vi "main BK20240228.vi"() -> ()   [LabVIEW 2024]
doc: "Main VI for FLS imaging system."
uses:
  <userlib>/_OpenG.lib/file/file.llb/openg_file.lvlib
  <vilib>/event_ctls.llb/usereventprio.ctl
  <instrlib>/niScope/Acquire/Fetch/niScope Multi Fetch Binary 16.vi
  <instrlib>/niScope/Controls/niScope trigger source.ctl
  <userlib>/_OpenG.lib/time/time.llb/openg_time.lvlib
  LaguerreDeconLib/DeconEngineClass/LaguerreDeconEngineClass.lvclass
  SubVI/GlobalVariables.vi
  SubVI/LabJack/LJ Pin Setting.ctl
  <vilib>/Utility/error.llb/DialogType.ctl
  <vilib>/Analysis/NI_AALBase.lvlib
  <vilib>/Utility/miscctls.llb/LVMinMaxIncTypeDef.ctl
  <vilib>/Analysis/baseanly.llb/Mean (DBL).vi
  <vilib>/Utility/miscctls.llb/LVPointTypeDef.ctl
  SubVI/APD/APDClass.lvclass
  ConfigFiles/AimingBeamVideoConfig.ctl
  <vilib>/addons/control/pid/NI_PID_pid.lvlib
  <vilib>/addons/control/pid/pid.llb/PID (DBL).vi
  <vilib>/Instr/_visa.llb/VISA Configure Serial Port (Instr).vi
  SubVI/DigitizerConfiguration/FLImDAQ.ctl
panel:
  out "RunStartTime":u32
  out "Dig1 Temp":dbl
  out "Dig2 Temp":dbl
  out "Visualization PC video source":T1
  in  "V target(1.0)":dbl=1.0 caption="V target(1.5)" min=0.3 max=1.5 step=0.1 format="%#_4g"
  out "SNR3":dbl format="%#_3g"
  out "SNR2":dbl format="%#_3g"
  out "SNR1":dbl format="%#_3g"
  in  "Show BG removed?":bool=TRUE
  out "IntR3":dbl format="%#_2g"
  out "IntR2":dbl format="%#_2g"
  out "IntR1":dbl format="%#_2g"
  in  "Video Display":bool
  out "Gain3":dbl
  out "Gain2":dbl
  out "Gain1":dbl
  in  "Skip Data Save?":bool
  out "Aq Loop?":bool
  out "ML?":bool
  out "aquisition loop Error Out":errorcluster
  out "Laser f (Hz)":dbl
  out "Record Backlog":i32
  out "Fetch Record #":i32
  out "Sync Success?":bool
  out "Disclamer":picture
  out "Calibration #":i8
  out "BG #":i8
  in  "TCP Connect":bool
  out "Help":string
  in  "355nm Laser toggle":bool caption="355nm 460Hz"
  in  "Cali&iRF alignment":bool
  in  "Background":bool
  in  "Aiming beam toggle":bool caption="445nm 15Hz 35mA"
  out "Lifetime 3":dbl
  out "Lifetime 2":dbl
  in  "Auto gain ch3":bool=TRUE
  in  "Auto gain ch2":bool=TRUE
  in  "Auto gain ch1":bool=TRUE
  out "Run #":i8
  in  "StopButton":bool caption="Stop"
  out "Aquisition Status:":bool
  in  "StartButton":bool caption="Start"
  in  "V 3":dbl caption="Gain 3" min=0.0 max=4.6494 step=0.1
  in  "V 2":dbl caption="Gain 2" min=0.0 max=4.61 step=0.1
  out "Lifetime 1":dbl
  in  "V 1":dbl caption="Gain 1" min=0.0 max=4.6492 step=0.1 format="%#_4g"
  in  "Video Source":enum32{"Camera", "FrameGrabber"}(radio)
  out "Case #":string
  out "System Hardware Connection Status":T2
  out "Channel 3":dbl[][](graph)
  out "Channel 2":dbl[][](graph)
  out "Channel 1":dbl[][](graph)
  in  "Tab Control":T3(tab)
  out "display loop timing(ms)":u32
  out "Aquisition loop timing(ms)":u32 format="%.2f"
  out "DisplayLoop":i32
  out "PID loop":i32 caption="processing loop"
  out "PID loop timing(ms)":u32 caption="processing loop timing(ms)"
  out "Communication loop(ms)":u32
  out "laser EM lamp V":dbl format="%0.6f"
  out "Decon Loop timing (ms)":dbl
  out "Auisition Loop idx":i32
  in  "Show BG":bool
  out "iRF length":i32
  out "BG length":i32
  out "data length":i32
  out "SysConfigCluster":T4
  out "LJ Pinout":T5={"Ch1 Bias"="DAC0", "Ch2 Bias"="DAC1", "Ch3 Bias"="DAC2", "Ch4 Bias"="DAC0", "355 PWM"="FIO0", "AimingBeam PWM"="FIO2", "Laser Ready"="FIO3", "Interlock"="FIO1", "Laser Start/Stop"="FIO1", "Red LED"="FIO1", "Green LED"="DIO3", "Foot Pedal"="DIO15"}
  out "FLImDAQ":T6={"Digitizer 1"="", "Digitizer 2"="", "Channel"=enum."Channel 0", "trigger source"="VAL_EXTERNAL", "trigger level"=0.5, "trigger delay"=1.35e-07, "min sample rate"=12500000000.0, "min record length"=2500, "vertical range"=1.0, "vertical offset"=-0.25, "Waveform to Avg"=2000} caption="FLIm DAQ Configuration" {"trigger delay" format="%^#.4e"; "trigger level" min=0.0 max=3.5 step=0.5 format="%.2f"; "vertical offset" format="%.4f"; "vertical range" format="%.2f"; "min sample rate" format="%#.2p"}
  in  "Sys Reconfig":bool
  out "data out(communcation loop)":string
  out "PID loop error out":errorcluster caption="processing Error Out"
  out "decon error out":errorcluster
  out "Laser Rep Rate":dbl
  in  "Data Class":enum16{"Data", "BG", "Cali"}(ring)
  out "V1 Size":i32
  out "V2 Size":i32
  out "V3 Size":i32
  out "data Size":i32[](array[numeric])
  out "State log":string
  in  "Ch3 PID gains":T8={"proportional gain (Kc)"=30.0, "integral time (Ti, min)"=0.0003, "derivative time (Td, min)"=1e-05}
  in  "Ch2 PID gains":T8={"proportional gain (Kc)"=30.0, "integral time (Ti, min)"=0.0003, "derivative time (Td, min)"=1e-05}
  in  "Ch1 PID gains":T8={"proportional gain (Kc)"=30.0, "integral time (Ti, min)"=0.0003, "derivative time (Td, min)"=1e-05}
  in  "Quit":bool
  in  "Radio Buttons":enum32{"No Selection", "Ch1", "Ch2", "Ch3"}(radio)=enum."Ch2" caption="DeCon Chan"
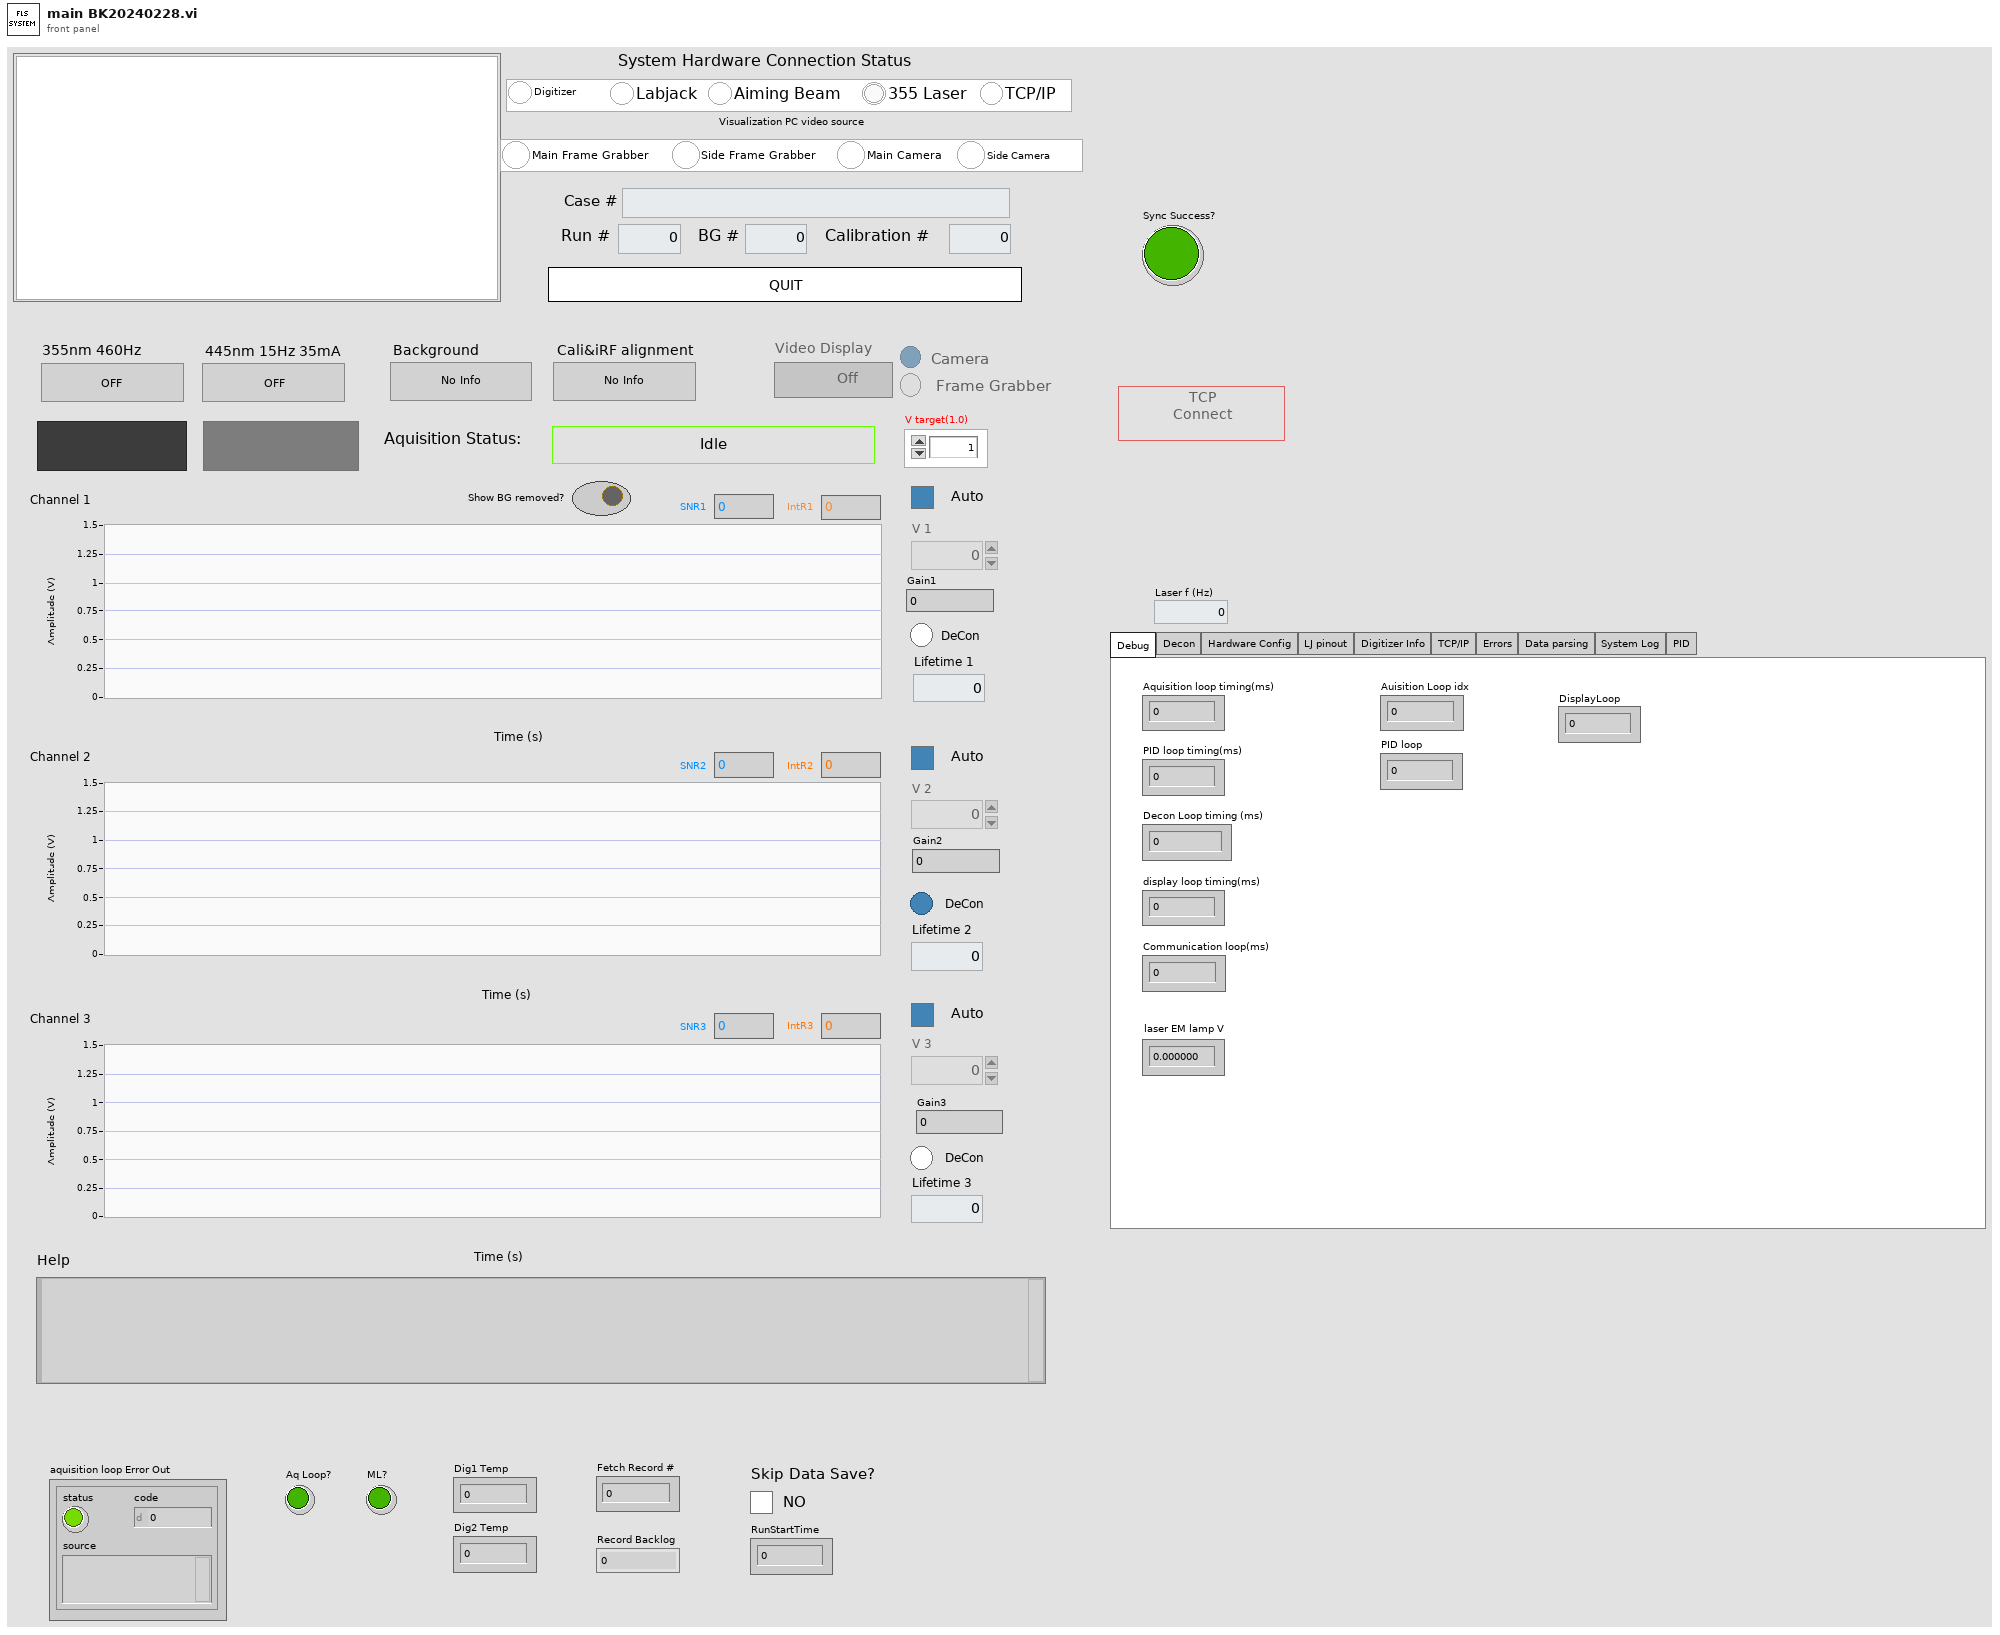
[diagram p1: front panel]
types:
  T1 = cluster{"Main Frame Grabber":bool, "Side Frame Grabber":bool, "Main Camera":bool, "Side Camera":bool}
  T2 = cluster{"Digitizer":bool, "Labjack":bool, "Aiming Beam":bool, "355 Laser":bool, "TCP/IP":bool}
  T3 = enum32{"Debug", "Decon", "Hardware Config", "LJ pinout", "Digitizer Info", "TCP/IP", "Errors", "Data parsing", "System Log", "PID"}
  T4 = cluster{"Ch1Enable?":bool, "Ch2Enable?":bool, "Ch3Enable?":bool, "Ch1AutoGain?":bool, "Ch2AutoGain?":bool, "Ch3AutoGain?":bool, "AimingBeamEnable?":bool}
  T5 = typedef "LJ Pin Setting.ctl" = cluster{"Ch1 Bias":string, "Ch2 Bias":string, "Ch3 Bias":string, "Ch4 Bias":string, "355 PWM":string, "AimingBeam PWM":string, "Laser Ready":string, "Interlock":string, "Laser Start/Stop":string, "Red LED":string, "Green LED":string, "Foot Pedal":string}
  T6 = typedef "FLImDAQ.ctl" = cluster{"Digitizer 1":refnum<k15>, "Digitizer 2":refnum<k15>, "Channel":enum16{"Channel 0", "Channel 1", "Channel 0&1"}, "trigger source":T7, "trigger level":dbl, "trigger delay":dbl, "min sample rate":dbl, "min record length":i32, "vertical range":dbl, "vertical offset":dbl, "Waveform to Avg":i16}
  T7 = typedef "niScope trigger source.ctl" = string
  T8 = cluster{"proportional gain (Kc)":dbl, "integral time (Ti, min)":dbl, "derivative time (Td, min)":dbl}
  T9 = cluster{"remote start event":refnum<user-event>, "remote stop  event":refnum<user-event>}
  T10 = enum8{"Enabled", "Disabled", "Disabled and Grayed Out"}
  T11 = enum16{"open", "replace", "create", "open or create", "replace or create", "replace or create with confirmation"}
  T12 = cluster{"CH1":dbl[][], "CH2":dbl[][], "CH3":dbl[][], "Gain cluster":cluster{"V1":dbl, "V2":dbl, "V3":dbl}}
  T13 = cluster{"idx":i32, "CH1&2":dbl[][], "CH3":dbl[][], "V cluster":cluster{"V1":dbl, "V2":dbl, "V3":dbl}}
  T14 = typedef "usereventprio.ctl" = enum32{"high priority", "normal priority"}
  T15 = cluster{"actualSamples":i32, "absoluteInitialX":dbl, "relativeInitialX":dbl, "xIncrement":dbl, "offset":dbl, "gain":dbl, "reserved1":dbl, "reserved2":dbl}[]
  T16 = cluster{"V1 out":dbl, "V2 out":dbl, "V3 out":dbl}
  T17 = cluster{i32, dbl[][], dbl[][], cluster{"V1 out":dbl, "V2 out":dbl, "V3 out":dbl}}
  T18 = cluster{"Ch1 WF":dbl[], "Ch2 WF":dbl[], "Ch3 WF":dbl[], "V1":dbl, "V2":dbl, "V3":dbl}
  T19 = enum16{"open", "open or create", "create or replace", "create", "open (read-only)"}
  T20 = enum32{"Invalid", "Standard", "Closed", "Hidden", "Minimized", "Maximized"}
  T21 = enum32{"invalid app kind", "Development System", "Run Time System", "Student Edition", "Embedded LabVIEW", "Evaluation", "Custom"}
  T22 = enum32{"Bad", "Idle", "Run top level", "Running"}
  T23 = enum16{"Standard", "Buffered", "CRLF", "Immediate"}
  T24 = typedef "AimingBeamVideoConfig.ctl" = cluster{"DeCon Channel":enum16{"1", "2", "3"}, "Scale Bar":bool, "Scale Low":dbl, "Scale High":dbl, "ANSI":dbl, "Radius":dbl, "3D?":bool, "Firefly?":bool, "Pentero?":bool}
  T25 = cluster{"Core":cluster{"Current VI Reference":refnum<vi>, "Close Panel on Exit?":bool}, "SysConfigCluster":cluster{"Ch1Enable?":bool, "Ch2Enable?":bool, "Ch3Enable?":bool, "Ch1AutoGain?":bool, "Ch2AutoGain?":bool, "Ch3AutoGain?":bool, "AimingBeamEnable?":bool}, "System Status":cluster{"Digitizer":bool, "Labjack":bool, "Aiming Beam":bool, "355 Laser":bool, "TCP/IP":bool}, "IDs":cluster{"RunID":i8, "BG ID":i8, "Cali ID":i8}, "CaseID":string, "DefaultPath":path, "Pathes":cluster{"DataPath":path, "BG Path":path, "iRFPath":path, "CaliPath":path}, "FLImDAQ":cluster{"resource name":refnum<k15>, "resource name 2":refnum<k15>, "Channel":enum16{"Channel 0", "Channel 1", "Channel 0&1"}, "trigger source":T7, "trigger level":dbl, "trigger delay":dbl, "min sample rate":dbl, "min record length":i32, "vertical range":dbl, "vertical offset":dbl, "Waveform to Avg":i32}, "SysRunning?":bool, "AB Cluster":cluster{"Aiming Beam COM Port":refnum<visa-resource-name>, "Min Current":dbl, "Max Current":dbl, "Default Current":dbl, "Freq":i32}, "LJ Pinout":T5, "355 PWM setting":cluster{"DIO_EF_CLOCK1_DIVISOR":i16, "DIO_EF_CLOCK1_ROLL_VALUE":i32, "DIO#_EF_INDEX":i16, "DIO#_EF_OPTIONS":i16, "DIO#_EF_CONFIG_A":i32}, "AB PWM setting":cluster{"DIO_EF_CLOCK1_DIVISOR":i16, "DIO_EF_CLOCK1_ROLL_VALUE":i32, "DIO#_EF_INDEX":i16, "DIO#_EF_OPTIONS":i16, "DIO#_EF_CONFIG_A":i32}, "Last Trigger":u32, "niTClk sessions":refnum<k20>[], "Laser start tic":u32, "TCP attempt count":i32, "Ch1Data":dbl[][], "Ch2Data":dbl[][], "Ch3Data":dbl[][], "V1":dbl[], "V2":dbl[], "V3":dbl[], "SlowTimer":u32, "FastTimer":u32, "listener ID":refnum<k5>, "TempPath":path, "LED vi reference":refnum<vi>, "Aquisition Timer":u32, "APDSerialNum":cluster{"Ch1APDSerial#":string, "Ch2APDSerial#":string, "Ch3APDSerial#":string}, "VideoConfig":T24, "CaliPath":path, "LED vi ref open?":bool, "video source":cluster{"Main Frame Grabber":bool, "Side Frame Grabber":bool, "Main Camera":bool, "Side Camera":bool}, "bothVidSourceAvail":bool}
  T26 = typedef "LVCursorListTypeDef.ctl" = cluster{"Name":string, "Color":u32, "Style":u8, "Point Style":u8, "Name Visible":bool, "Allow Drag":bool, "Cursor Mode":u32, "Plot":i32, "Index":i32, "Position":cluster{"X":dbl, "Y":dbl}, "X Scale":u32, "Y Scale":u32, "Watch Plots":i32[], "Watch All Plots":bool, "Plot Area":i32, "Label Offset":cluster{"X":dbl, "Y":dbl}}[]
  T27 = cluster{"Name":string, "Color":u32, "Style":u8, "Point Style":u8, "Name Visible":bool, "Allow Drag":bool, "Cursor Mode":u32, "Plot":i32, "Index":i32, "Position":cluster{"X":dbl, "Y":dbl}, "X Scale":u32, "Y Scale":u32, "Watch Plots":i32[], "Watch All Plots":bool, "Plot Area":i32, "Label Offset":cluster{"X":dbl, "Y":dbl}}
  T28 = cluster{"Ch1APDSerial#":string, "Ch2APDSerial#":string, "Ch3APDSerial#":string}
  T29 = cluster{"DataPath":path, "BG Path":path, "iRFPath":path, "CaliPath":path}
  T30 = cluster{"DIO_EF_CLOCK1_DIVISOR":i16, "DIO_EF_CLOCK1_ROLL_VALUE":i32, "DIO#_EF_INDEX":i16, "DIO#_EF_OPTIONS":i16, "DIO#_EF_CONFIG_A":i32}
  T31 = cluster{"Aiming Beam COM Port":refnum<visa-resource-name>, "Min Current":dbl, "Max Current":dbl, "Default Current":dbl, "Freq":i32}
  T32 = cluster{"resource name":refnum<k15>, "resource name 2":refnum<k15>, "Channel":enum16{"Channel 0", "Channel 1", "Channel 0&1"}, "trigger source":T7, "trigger level":dbl, "trigger delay":dbl, "min sample rate":dbl, "min record length":i32, "vertical range":dbl, "vertical offset":dbl, "Waveform to Avg":i32}
  T33 = cluster{"Current VI Reference":refnum<vi>, "Close Panel on Exit?":bool}
  T34 = typedef "iRFData.ctl" = cluster{"dt":dbl, "NumOfWFs":i32, "WFLength":i32, "iRFCtrlV":dbl[], "iRFWFsAvg":dbl[][], "iRFRaw":dbl[][]}
  T35 = cluster{"iRFWFsAvg":dbl[], "iRFWFsAvg":dbl[], "iRFWFsAvg":dbl[]}
  T36 = cluster{"V 1":dbl[], "V 2":dbl[], "V 3":dbl[], "V 4":dbl[]}
  T37 = cluster{"Channel 1":dbl[], "Channel 2":dbl[], "Channel 3":dbl[], "Channel 4":dbl[]}
  T38 = cluster{"DataPath":path, "CaseID":string, "RunID":i8, "Ch1Data":dbl[][], "Ch2Data":dbl[][], "Ch3Data":dbl[][], "V1":dbl[], "V2":dbl[], "V3":dbl[], "LaserRepRate":u32, "WFAverage":i16, "RunStartTime":u32}
  T39 = typedef "DialogType.ctl" = u16
  T40 = cluster{"Ch1 iRF":dbl[], "Ch2 iRF":dbl[], "Ch3 iRF":dbl[], "Ch4 iRF":dbl[]}
  T41 = cluster{"Ch1APDSerial#":string, "Ch2APDSerial#":string, "Ch3APDSerial#":string, "Ch4APDSerial#":string}
  T42 = typedef "LJ PWM Setting.ctl" = cluster{"DIO_EF_CLOCK1_DIVISOR":i16, "DIO_EF_CLOCK1_ROLL_VALUE":i32, "DIO#_EF_INDEX":i16, "DIO#_EF_OPTIONS":i16, "DIO#_EF_CONFIG_A":i32}
  T43 = typedef "AimingBeam.ctl" = cluster{"Aiming Beam COM Port":refnum<visa-resource-name>, "Min Current":dbl, "Max Current":dbl, "Default Current":dbl, "Frequency(Hz)":u32}
  T44 = cluster{"DC1":i32, "DC2":i32, "BG1":i32, "BG2":i32}
  T45 = typedef "LVMinMaxIncTypeDef.ctl" = cluster{"Minimum":dbl, "Maximum":dbl, "Increment":dbl}
  T46 = typedef "LVBoundsTypeDef.ctl" = cluster{"Width":u32, "Height":u32}
  T47 = typedef "imagedata.ctl" = cluster{"image type":i32, "image depth":i32, "image":u8[], "mask":u8[], "colors":u32[], "Rectangle":cluster{"left":i16, "top":i16, "right":i16, "bottom":i16}}
  T48 = enum32{"No Selection", "Ch1", "Ch2", "Ch3", "Ch4"}
  T49 = cluster{"DC Idx1":i32, "DC Idx2":i32, "BG Idx1":i32, "BG Idx2":i32}
  T50 = cluster{dbl[][], dbl[][], dbl[][], "V cluster":cluster{"V1":dbl, "V2":dbl, "V3":dbl}}
  T51 = typedef "LVPointTypeDef.ctl" = cluster{"Horizontal":i16, "Vertical":i16}
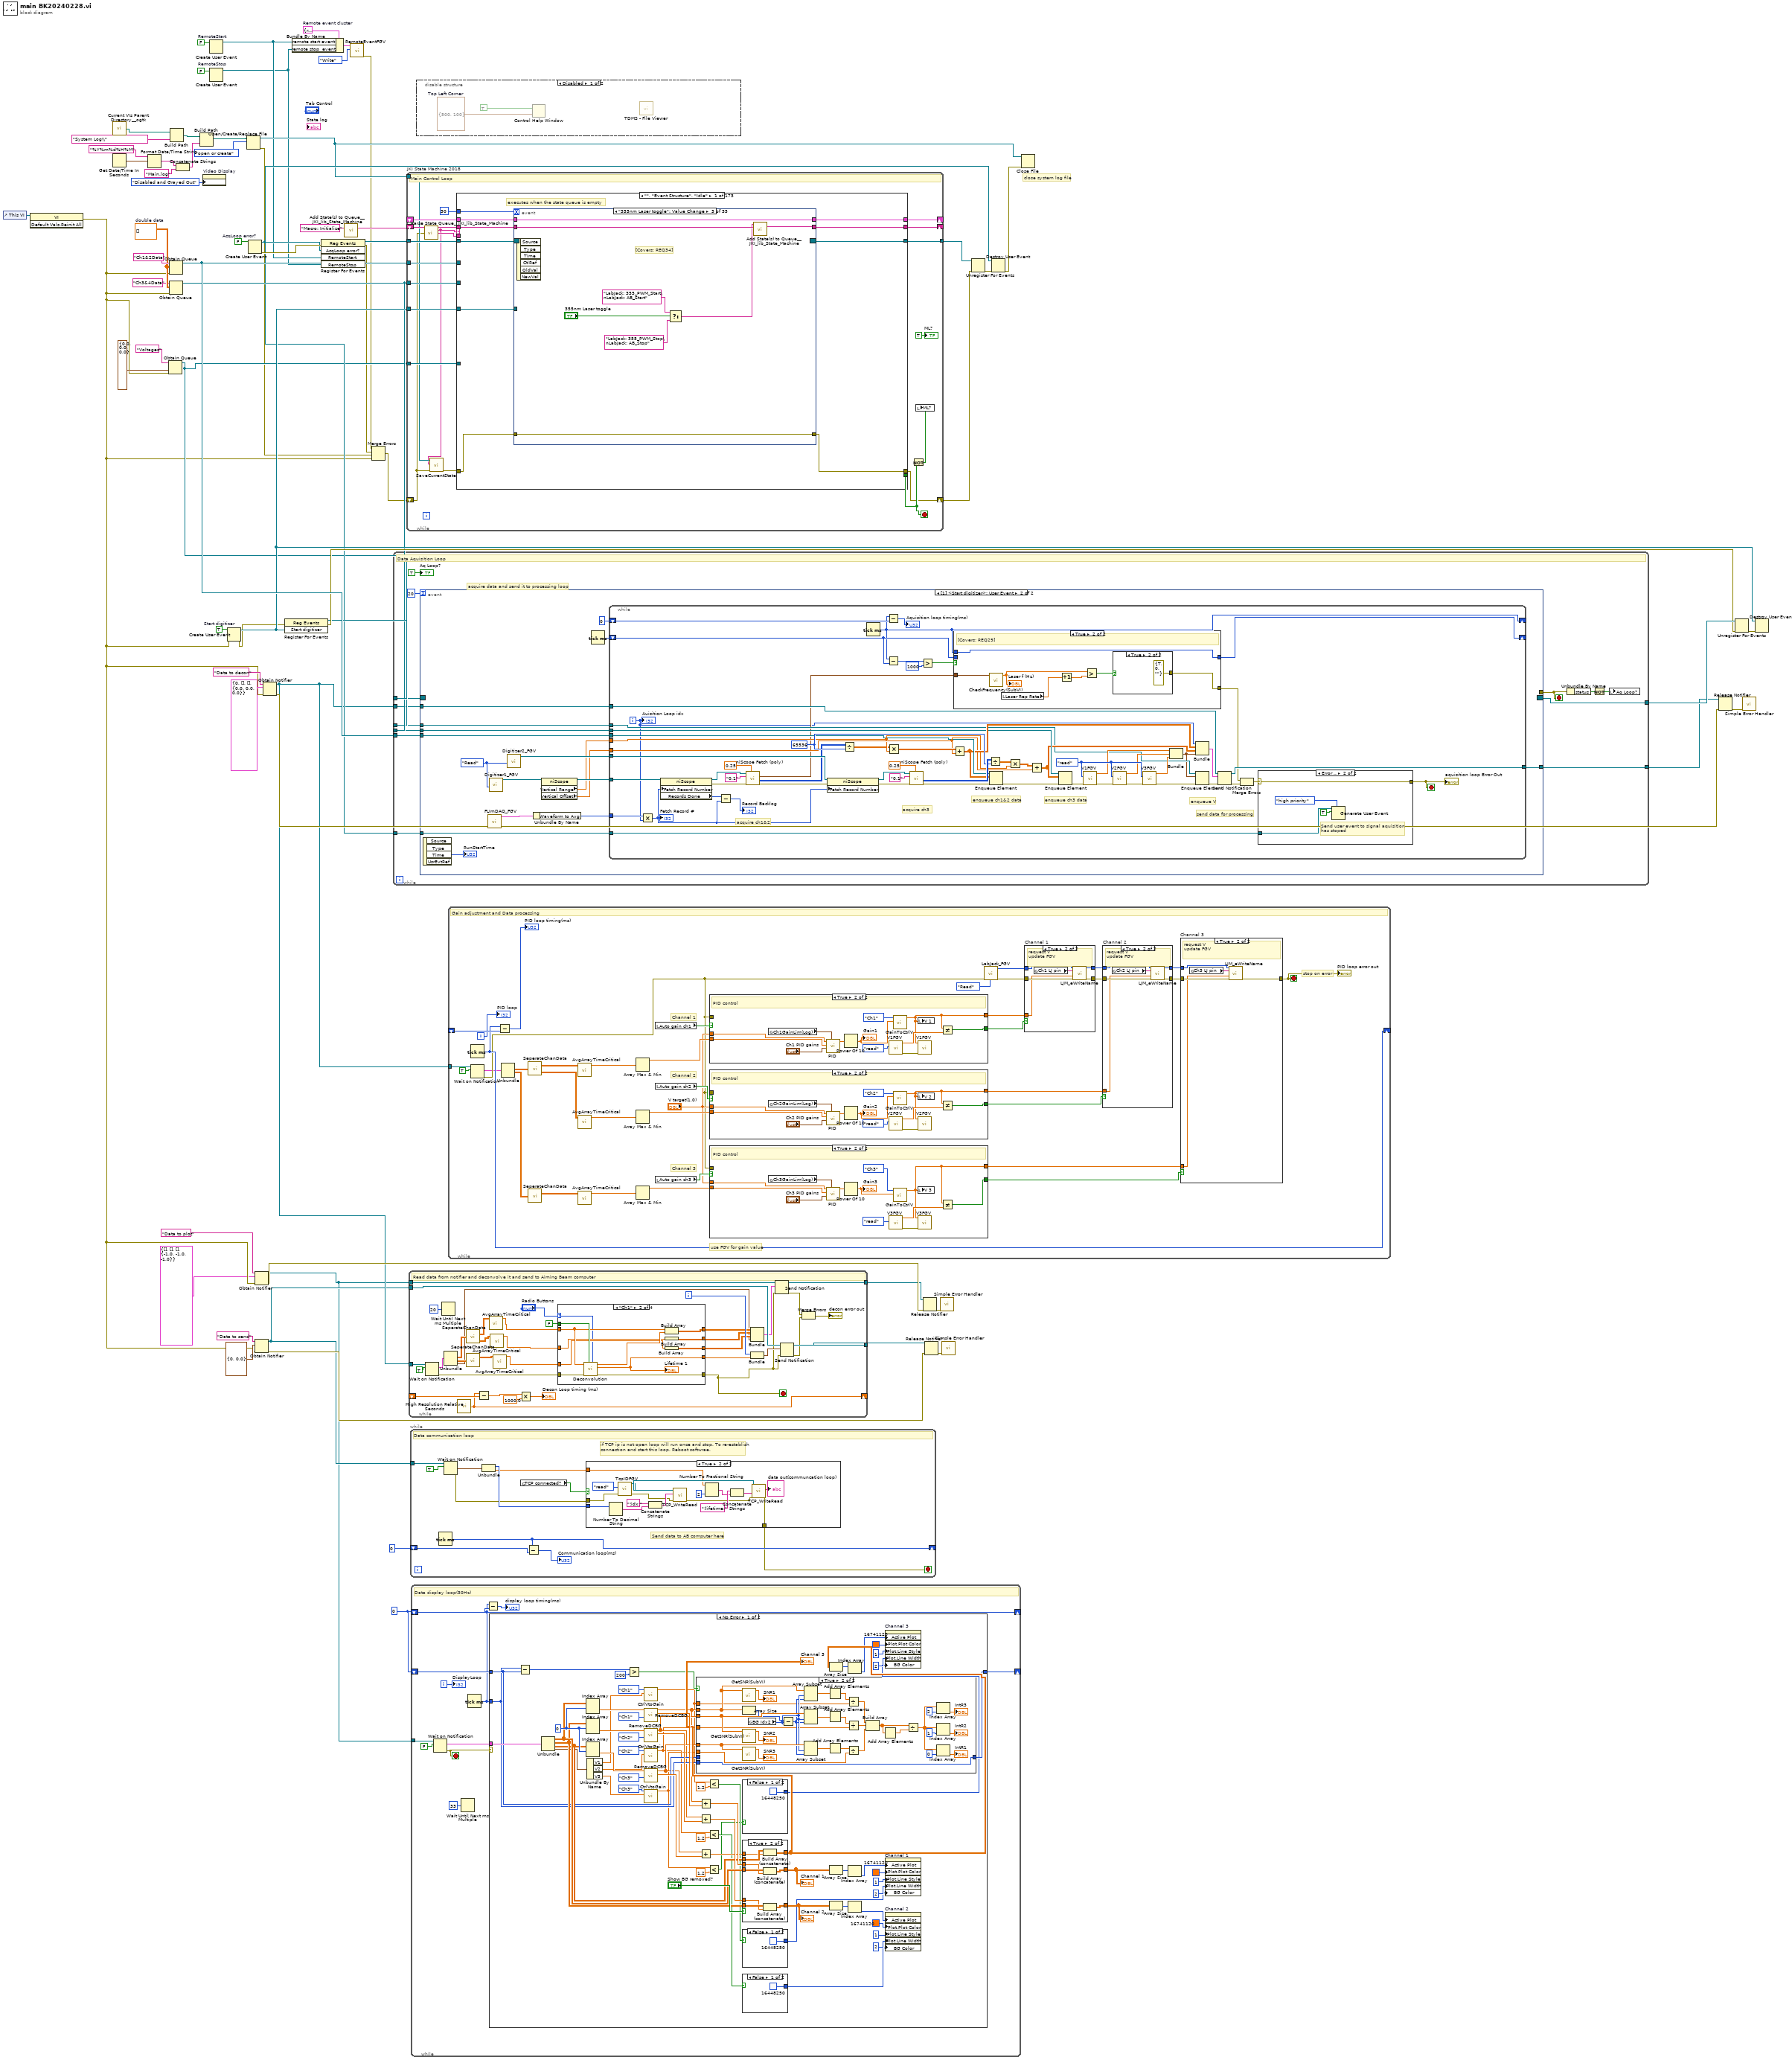
[diagram p0: block diagram]
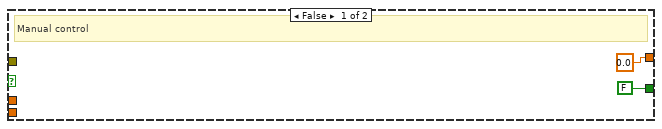
[diagram p2: hidden frame]
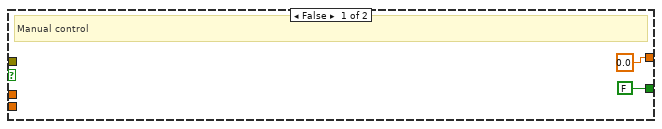
[diagram p6: hidden frame]
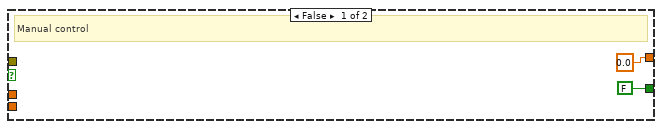
[diagram p7: hidden frame]
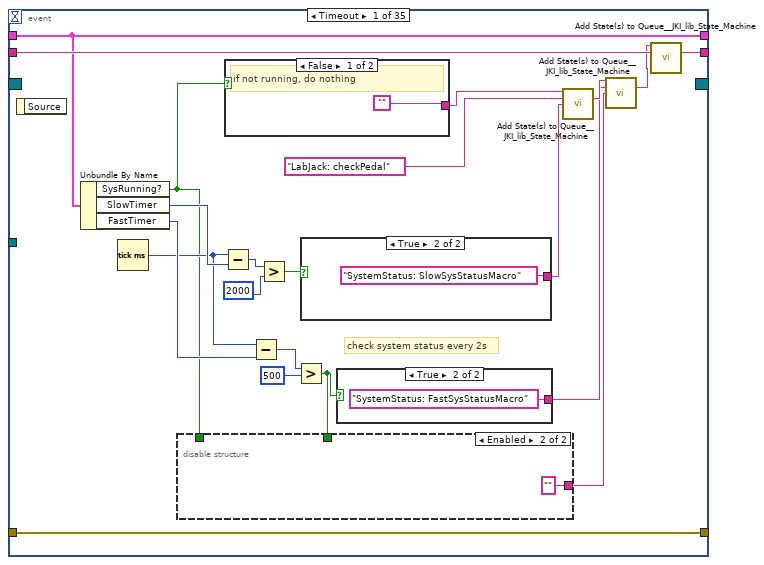
[diagram p8: hidden frame]
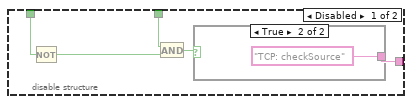
[diagram p9: hidden frame]
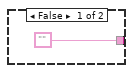
[diagram p10: hidden frame]
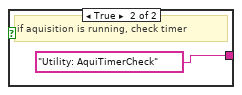
[diagram p11: hidden frame]
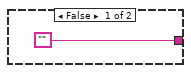
[diagram p12: hidden frame]
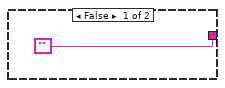
[diagram p13: hidden frame]
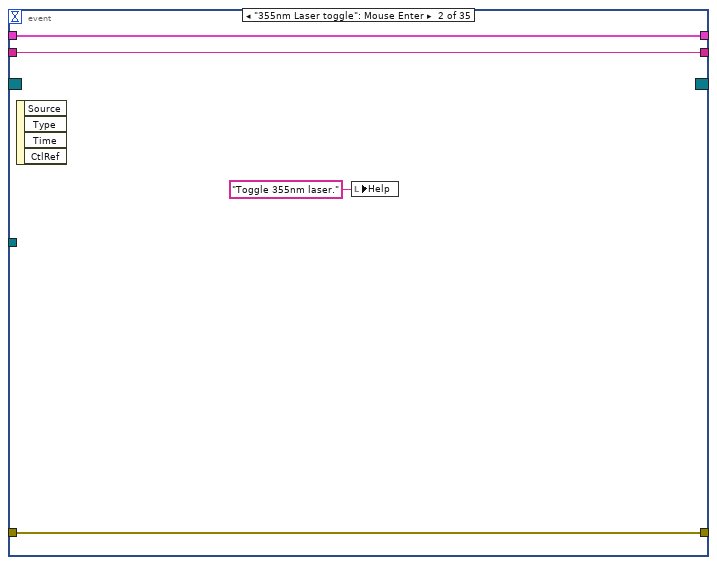
[diagram p14: hidden frame]
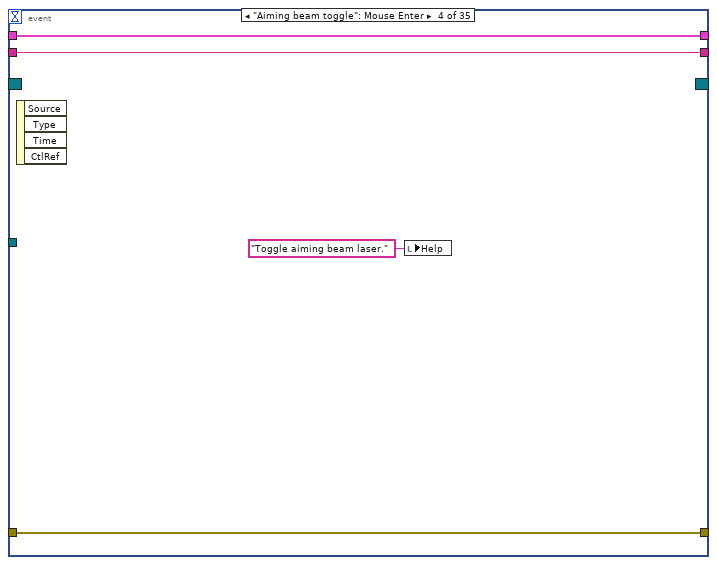
[diagram p15: hidden frame]
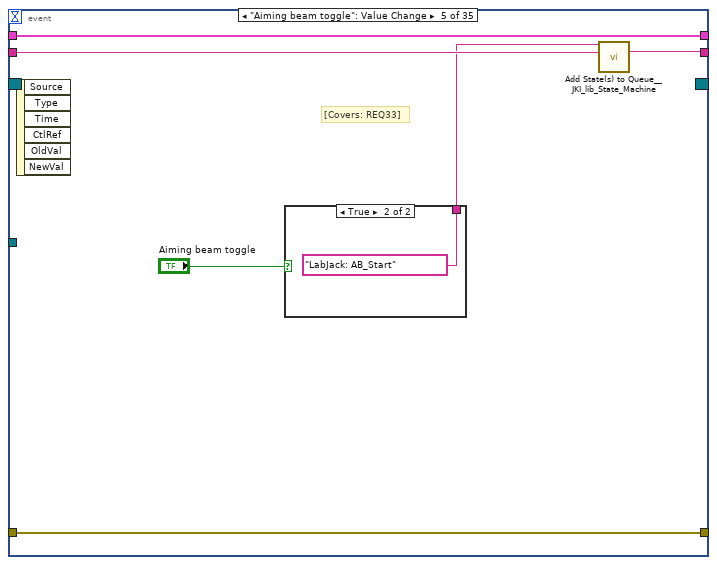
[diagram p16: hidden frame]
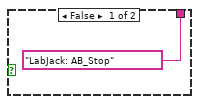
[diagram p17: hidden frame]
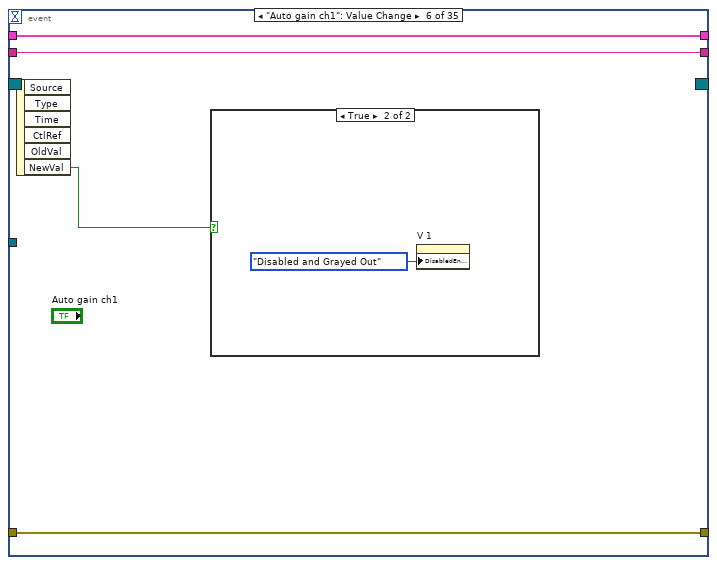
[diagram p18: hidden frame]
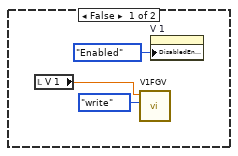
[diagram p19: hidden frame]
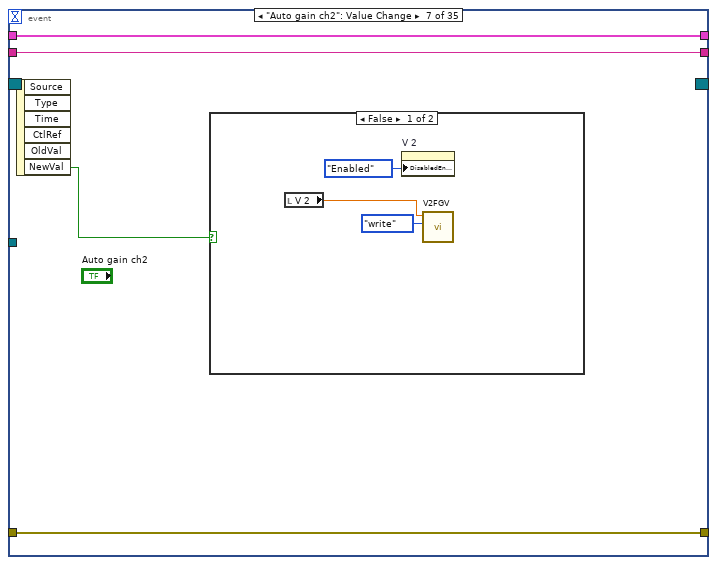
[diagram p20: hidden frame]
diagram:
  w7 = T9 {"remote start event"=refnum, "remote stop  event"=refnum}  # Remote event cluster
  w10 = FALSE  # RemoteStop
  w11 = FALSE  # RemoteStart
  w14 = u32 0 ("millisecond timer value")
  w53 = FALSE  # AcqLoop error?
  w63 = TRUE  # Start digitizer
  w66 = dbl[][] []  # double data
  # "close system log file"
  n1 = control-ref of="This VI"() -> (w68:refnum<vi>)
  n2 = invoke on="Invoke Node" class="VI" method="Default Vals.Reinit All"(reference=w68) -> (error out=w22:errorcluster)  [unwired: 2 in, 2 out]
  n3 = call <userlib>:"Current VIs Parent Directory__ogtk.vi"() -> ("Parent Directory (+ Relative)"=w33:path)  [unwired: 5 in]
  n4 = Get Date/Time In Seconds() -> (seconds since 1Jan1904=w31:timestamp)
  n5 = Format Date/Time String(time format string (%c)="%Y%m%d%H%M", seconds (now)=w31) -> (date/time string=w28:string)  [unwired: 1 in]
  n6 = Obtain Queue(name (unnamed)="Voltages", element data type=cluster{"V1":dbl, "V2":dbl, "V3":dbl} {"V1"=0.0, "V2"=0.0, "V3"=0.0}, error in (no error)=w22) -> (queue out=w34:refnum<queue>)  [unwired: 2 in, 2 out]
  n7 = Obtain Queue(name (unnamed)="Ch3&4Data", element data type=w66, error in (no error)=w22) -> (queue out=w47:refnum<queue>)  [unwired: 2 in, 2 out]
  n8 = Obtain Queue(name (unnamed)="Ch1&2Data", element data type=w66, error in (no error)=w22) -> (queue out=w64:refnum<queue>)  [unwired: 2 in, 2 out]
  n9 = Build Path(base path=w33, name or relative path="System Log\\") -> (appended path=w24:path)
  n10 = Concatenate Strings(w28, "Main.log" ("string")) -> (w26:string)
  n11 = Build Path(base path=w24, name or relative path=w26) -> (appended path=w29:path)
  n12 = property on="Video Display" class="Bool (strict)"("DisabledEnum"=T10."Disabled and Grayed Out" ("Disabled")) -> ()  [unwired: 2 in, 2 out]
  n13 = Create User Event(user event datatype=w11) -> (user event=w9:refnum<user-event>)  [unwired: 1 in, 1 out]
  n14 = Create User Event(user event datatype=w10) -> (user event=w8:refnum<user-event>)  [unwired: 1 in, 1 out]
  n15 = Create User Event(user event datatype=w63, error in=w22) -> (user event=w52:refnum<user-event>, error out=w39:errorcluster)
  n16 = Open/Create/Replace File(file path (use dialog)=w29, operation (0:open)=T11."open or create") -> (refnum out=w20:refnum<file>, error out=w21:errorcluster)  [unwired: 4 in, 1 out]
  n17 = Create User Event(user event datatype=w53) -> (user event=w38:refnum<user-event>, error out=w40:errorcluster)  [unwired: 1 in]
  n18 = Obtain Notifier(name (unnamed)="Data to plot", notification data type=T12 {"CH1"=[], "CH2"=[], "CH3"=[], "Gain cluster"={"V1"=-1.0, "V2"=-1.0, "V3"=-1.0}}, error in (no error)=w22) -> (notifier out=w12:refnum<notifier>, error out=w48:errorcluster)  [unwired: 1 in, 1 out]
  n19 = Obtain Notifier(name (unnamed)="Data to send", notification data type=cluster{"idx":i32, "lifetime":dbl} {"idx"=0, "lifetime"=0.0}, error in (no error)=w22) -> (notifier out=w17:refnum<notifier>, error out=w37:errorcluster)  [unwired: 1 in, 1 out]
  n20 = Obtain Notifier(name (unnamed)="Data to decon", notification data type=T13 {"idx"=0, "CH1&2"=[], "CH3"=[], "V cluster"={"V1"=0.0, "V2"=0.0, "V3"=0.0}}, error in (no error)=w22) -> (notifier out=w18:refnum<notifier>, error out=w57:errorcluster)  [unwired: 1 in, 1 out]
  n21 = register-events(error in=w39, w52) -> (reference out=w54:refnum<event-registration>, error out=w60:errorcluster)  [unwired: 1 in]
  n22 = Bundle By Name(cluster=w7, "remote start event"=w9, "remote stop  event"=w8) -> (w5:T9)
  n23 = register-events(error in=w40, w38, w9, w8) -> (reference out=w46:refnum<event-registration>, error out=w4:errorcluster)  [unwired: 1 in]
  n24 = call <vilib>:"Add State(s) to Queue__JKI_lib_State_Machine.vi"("State(s) in (\"\")"="Macro: Initialize") -> ("States Out"=w70:string)  [unwired: 14 in]
  n25 = call "RemoteEventFGV.vi"("Operation (Read)"=enum16{"Read", "Write"}."Write", "Remote Event in"=w5) -> ("Error Out"=w1:errorcluster)  [unwired: 8 in, 1 out]
  n26 = Merge Errors(w1, w4, w21, w22) -> (w23:errorcluster)
  n27 = while {
    tunnel: w64 -> [w83]
    tunnel: w54 -> [w82]
    tunnel: [w81] -> w62
    tunnel: w18 -> [w80]
    tunnel: [w79] -> w58
    tunnel: w38 -> [w77]
    tunnel: w47 -> [w76]
    tunnel: w34 -> [w71]
    stop <- w74 stop-if-true
    # "acquire data and send it to processing loop"
    # "Data Aquisition Loop"
    n28 = event shown="[1] <Start digitizer>: User Event" {
      selector: w82 -> [_ _]
      dyn-events: [_ _] -> w81
      timeout: 20 -> [_ _]
      tunnel: w83 -> [w89 w99]
      tunnel: [w84 _] -> w74
      tunnel: w80 -> [w88 w106]
      tunnel: [w88 w105] -> w79
      tunnel: w77 -> [_ w103]
      tunnel: w76 -> [w87 w98]
      tunnel: w71 -> [_ w96]
      event Timeout {
        # "use queue to stop data loop\nwhen queue ref is released, error will stop this loop"
        n29 = event-data() -> ()  [unwired: 1 in, 3 out]
        n30 = Get Queue Status(queue=w89) -> (error out=w86:errorcluster)  [unwired: 2 in, 7 out]
        n31 = Get Queue Status(queue=w87) -> (error out=w85:errorcluster)  [unwired: 2 in, 7 out]
        n32 = Merge Errors(w86, w85) -> (w84:errorcluster)
      }
      event User Event {
        w104 = enum16{"Write", "Read"}."Read" ("Operation")
        n33 = event-data() -> ("Time"=→"RunStartTime":u32)  [unwired: 1 in, 3 out]
        n34 = call "FLImDAQ_FGV.vi"() -> ("Read data"=w101:T6)  [unwired: 10 in, 1 out]
        n35 = call "Digitizer1_FGV.vi"("Operation (Read)"=w104) -> ("Read data"=w95:refnum<k15>)  [unwired: 9 in, 1 out]
        n36 = call "Digitizer2_FGV.vi"("Operation (Read)"=w104) -> ("Read data"=w102:refnum<k15>)  [unwired: 9 in, 1 out]
        n37 = Unbundle By Name(w101) -> ("Waveform to Avg"=w100:i16)
        n38 = property on="Property Node" class="niScope"(reference=w95) -> (reference out=w94:refnum<k15>, "Vertical Range"=w93:dbl, "Vertical Offset"=w92:dbl)  [unwired: 1 in, 1 out]
        n39 = Tick Count (ms)() -> (millisecond timer value=w91:u32)
        n40 = while {
          tunnel: w106 -> [w161]
          tunnel: [w160] -> w105
          tunnel: w102 -> [w154]
          tunnel: w94 -> [w153]
          tunnel: w103 -> [w152]
          shift-right: [w115] -> _
          shift-left: u32 0 ("millisecond timer value") -> [w146]
          tunnel: w100 -> [w143]
          tunnel: w99 -> [w141]
          tunnel: w98 -> [w139]
          tunnel: w96 -> [w130]
          tunnel: w93 -> [w126]
          tunnel: w92 -> [w127]
          shift-right: [w121] -> _
          shift-left: w91 -> [w120]
          i -> [w107]
          stop <- w118 stop-if-true
          w134 = enum16{"write", "read"}."read" ("action")
          w147 = 65536
          # "enqueue V"
          # "enqueue ch3 data"
          # "enqueue ch1&2 data"
          # "acquire ch3"
          # "acquire ch1&2"
          # "send data for processing"
          n41 = Multiply(x=w143, y=w107) -> (x*y=w128:i32)
          "Fetch Record #" <- w128
          n42 = property on="Property Node" class="niScope"(reference=w153, "Fetch Record Number"=w128) -> (reference out=w165:refnum<k15>, error out=w164:errorcluster, "Records Done"=w129:i32)  [unwired: 1 in]
          n43 = Subtract(x=w129, y=w128) -> (x-y=→"Record Backlog":i32)
          n44 = call-poly <instrlib>:"niScope Fetch (poly).vi"("timeout"=0.25, "error in"=w164, "channels"="0,1", "instrument handle"=w165) -> ("error out"=w111:errorcluster, "wfm"=w144:i16[][], "wfm info"=w125:T15)  [unwired: 4 in, 1 out]
          n45 = property on="Property Node" class="niScope"(reference=w154, error in=w111, "Fetch Record Number"=w128) -> (reference out=w158:refnum<k15>, error out=w155:errorcluster)
          n46 = Divide(x=w144, y=w147) -> (x/y=w114:dbl[][])
          n47 = Tick Count (ms)() -> (millisecond timer value=w115:u32)
          n48 = Subtract(x=w115, y=w146) -> (x-y=→"Aquisition loop timing(ms)":u32)
          n49 = Subtract(x=w115, y=w120) -> (x-y=w124:u32)
          n50 = Multiply(x=w114, y=w126) -> (x*y=w151:dbl[][])
          n51 = call-poly <instrlib>:"niScope Fetch (poly).vi"("timeout"=0.25, "error in"=w155, "channels"="0,1", "instrument handle"=w158) -> ("error out"=w110:errorcluster, "wfm"=w148:i16[][])  [unwired: 4 in, 2 out]
          n52 = Greater?(x=w124, y=u32 1000) -> (0:w122:bool)
          n53 = Add(x=w151, y=w127) -> (x+y=w140:dbl[][])
          n54 = case shown="True" w122 {
            tunnel: w125 -> [_ w174]
            tunnel: w115 -> [_ w173]
            tunnel: [w167 w173] -> w121
            tunnel: w120 -> [w167 _]
            tunnel: [errorcluster {"status"=FALSE, "code"=0, "source"=""} ("error constant") w170] -> w116
            frame False {
            }
            frame True {
              # "[Covers: REQ29]"
              n55 = call "CheckFrequency(SubVI).vi"("wfm info"=w174) -> ("f (Hz)"=w172:dbl)  [unwired: 10 in]
              "Laser f (Hz)" <- w172
              n56 = local read "Laser Rep Rate"() -> (w169:dbl)
              n57 = Increment(x=w169) -> (x+1=w168:dbl)
              n58 = Greater?(x=w172, y=w168) -> (0:w171:bool)
              n59 = case shown="True" w171 {
                tunnel: [errorcluster {"status"=FALSE, "code"=0, "source"=""} ("error constant") errorcluster {"status"=TRUE, "code"=0, "source"=""} ("error constant")] -> w170
                frame False {
                }
                frame True {
                }
              }
            }
          }
          n60 = Divide(x=w148, y=w147) -> (x/y=w150:dbl[][])
          n61 = Enqueue Element(queue=w141, element=w140, error in (no error)=w110) -> (error out=w119:errorcluster)  [unwired: 1 in, 2 out]
          n62 = Multiply(x=w150, y=w126) -> (x*y=w149:dbl[][])
          n63 = Add(x=w149, y=w127) -> (x+y=w138:dbl[][])
          n64 = Enqueue Element(queue=w139, element=w138, error in (no error)=w119) -> (error out=w109:errorcluster)  [unwired: 1 in, 2 out]
          n65 = call "V1FGV.vi"("Error In"=w109, "action (write)"=w134) -> ("Error Out"=w136:errorcluster, "V1 out"=w133:dbl)  [unwired: 8 in]
          n66 = call "V2FGV.vi"("Error In"=w136, "action(write)"=w134) -> ("Error Out"=w135:errorcluster, "V2 out"=w132:dbl)  [unwired: 8 in]
          n67 = call "V3FGV.vi"("Error In"=w135, "action(write)"=w134) -> ("Error Out"=w112:errorcluster, "V3 out"=w131:dbl)  [unwired: 8 in]
          n68 = Bundle("V1 out"=w133, "V2 out"=w132, "V3 out"=w131) -> (w113:T16)  [unwired: 1 in]
          n69 = Bundle(w107, w140, w138, w113) -> (w142:T17)  [unwired: 1 in]
          n70 = Enqueue Element(queue=w130, element=w113, error in (no error)=w112) -> (error out=w108:errorcluster)  [unwired: 1 in, 2 out]
          n71 = Send Notification(notification=w142, notifier=w161, error in (no error)=w108) -> (notifier out=w160:refnum<notifier>, error out=w117:errorcluster)
          n72 = Merge Errors(w116, w117) -> (w137:errorcluster)
          n73 = case shown="Error .." w137 {
            selector: w137 -> [w177 w178]
            tunnel: w152 -> [_ w181]
            tunnel: [w177 w178] -> w118
            frame No Error {
            }
            frame Error {
              # "Send user event to signal aquisition has stoped"
              n74 = Generate User Event(priority (normal)=usereventprio."high priority", user event=w181, event data cluster=TRUE ("event data")) -> ()  [unwired: 1 in, 2 out]
            }
          }
          "aquisition loop Error Out" <- w118
          "Auisition Loop idx" <- w107
        }
      }
    }
    n75 = Unbundle By Name(w74) -> ("status"=w73:bool)
    n76 = Not(x=w73) -> (.not. x?=w72:bool)
    n77 = local write "Aq Loop?"(w72) -> ()
    "Aq Loop?" <- TRUE ("Aq L?")
  }
  n78 = while "JKI State Machine 2018" {
    shift-right: [w198] -> _
    shift-left: _ -> [w197]
    shift-right: [w182] -> w3
    shift-left: w23 -> [w184]
    shift-right: [w199] -> _
    shift-left: w70 -> [w200]
    tunnel: w64 -> [w195]
    tunnel: w47 -> [w194]
    tunnel: w52 -> [w193]
    tunnel: w46 -> [w192]
    tunnel: [w191] -> w45
    tunnel: w34 -> [w187]
    tunnel: w20 -> [w186]
    stop <- w190 stop-if-true
    # "Main Control Loop"
    n79 = call <vilib>:"Parse State Queue__JKI_lib_State_Machine.vi"("State Queue"=w200, "Error In (no error)"=w184) -> ("Remaining States"=w202:string, "Current State"=w185:string, "Arguments"=w201:string)  [unwired: 11 in]
    n80 = call "SaveCurrentState.vi"("error in (no error)"=w184, "Current State"=w185, "Byte Stream File in"=w186) -> ("error out"=w183:errorcluster)  [unwired: 8 in]
    n81 = case shown="\"\", \"Event Structure\", \"Idle\"" w185 {
      selector: w185 -> [_ _ _ _ _ _ _ _ _ _ _ _ _ _ _ _ _ _ _ _ _ _ _ w1047 _ _ _ _ _ _ _ _ _ _ _ _ _ _ _ _ _ _ _ _ _ _ _ _ _ _ _ _ _ _ _ _ _ _ _ _ _ _ _ _ _ _ _ _ _ _ _ _ _ _ _ _ _ _ _ _ _ _ _ _ _ _ _ _ _ _ _ _ _ _ _ _ _ _ _ _ _ _ _ _ _ _ _ _ _ _ _ _ _ _ _ _ _ _ _ _ _ _ _ _ _ _ _ _ _ _ _ _ _ _ _ _ _ _ _ _ _ _ _ _ _ _ _ _ _ _ _ _ _ _ _ _ _ _ _ _ _ _ _ _ _ _ _ _ _ _ _ _ _]
      tunnel: w202 -> [w212 w566 w575 w581 w587 w609 w622 w662 w696 w711 w740 w778 w790 w814 w842 w854 w880 w893 w959 w992 w1027 w1040 w1045 w1051 w1078 w1086 w1109 w1114 w1127 w1146 w1174 w1202 w1240 w1245 w1251 w1277 w1303 w1329 w1334 w1351 w1398 w1420 w1436 w1451 w1471 w1476 w1488 w1517 w1541 w1553 w1591 w1602 w1608 w1619 w1631 w1662 w1675 w1689 w1704 w1723 w1758 w1763 w1777 w1787 w1803 w1815 w1827 w1855 w1870 w1875 w1886 w1898 w1903 w1911 w1919 w1928 w1937 w1942 w1950 w1959 w1977 w1993 w2013 w2024 w2046 w2061 w2078 w2083 w2091 w2099 w2104 w2112 w2119 w2127 w2134 w2144 w2172 w2180 w2187 w2195 w2200 w2208 w2215 w2221 w2230 w2246 w2251 w2258 w2270 w2340 w2352 w2361 w2378 w2387 w2410 w2427 w2438 w2451 w2476 w2499 w2505 w2521 w2543 w2551 w2557 w2562 w2569 w2579 w2591 w2600 w2605 w2617 w2622 w2632 w2640 w2648 w2653 w2658 w2663 w2673 w2695 w2714 w2719 w2730 w2751 w2773 w2792 w2797 w2812 w2863 w2909 w2954 w2965 w2983 w3003 w3017 w3030 w3038 w3055 w3077 w3101 w3120 w3138 w3156 w3174 w3188 w3202 w3221 w3235 w3250 w3265 w3274 w3279]
      tunnel: w201 -> [_ _ _ _ _ _ _ _ _ _ _ _ _ _ _ _ _ _ _ _ _ _ _ _ _ _ _ _ _ _ _ _ _ _ _ _ _ _ _ _ _ _ _ _ _ _ _ _ _ _ _ _ _ _ w1629 _ _ _ _ _ _ _ _ _ _ _ _ _ _ _ _ _ _ _ _ _ _ _ _ _ _ _ _ _ _ _ _ _ _ _ _ _ _ _ _ w2135 _ _ _ _ _ _ _ _ _ _ _ w2253 w2264 _ _ _ _ w2384 _ _ _ _ _ w2495 _ _ _ _ _ _ w2564 _ _ _ _ _ _ w2628 _ _ _ _ _ _ _ _ _ _ _ _ _ _ _ _ _ _ _ _ _ _ _ _ _ _ _ _ _ _ _ _ _ _ _ _ _ _ _]
      tunnel: w197 -> [w210 w563 w571 w578 w584 w606 w619 _ w693 w701 w736 w774 w786 w806 w832 w851 w877 w890 w918 w984 w1014 w1035 w1042 w1049 w1071 w1083 w1107 w1111 w1115 w1136 w1166 w1194 w1236 w1242 w1248 w1255 w1282 w1308 w1331 w1344 w1388 w1417 w1421 w1448 w1468 w1473 w1477 w1506 w1531 w1546 w1570 w1600 w1605 w1612 w1627 w1645 w1670 w1681 w1699 w1716 w1741 w1760 w1773 w1781 w1800 w1812 w1824 w1843 w1859 w1872 w1884 w1896 w1900 w1905 w1912 w1924 w1933 w1939 w1946 w1956 w1964 w1980 w2008 w2014 w2043 w2054 w2076 w2080 w2084 w2092 w2101 w2110 w2116 w2124 w2131 w2141 w2169 w2177 w2184 w2192 w2197 w2202 w2213 w2218 w2224 w2243 w2248 w2256 w2266 w2337 w2342 w2355 w2376 w2385 w2400 w2424 w2435 w2445 w2469 w2496 w2502 w2514 w2539 w2548 w2554 w2559 w2566 w2573 w2587 w2597 w2602 w2614 w2619 w2625 w2637 w2645 w2650 w2655 w2660 w2670 w2693 w2712 w2716 w2728 w2749 w2771 w2790 w2794 w2805 w2857 w2905 w2951 w2961 w2978 w2998 w3012 w3026 w3032 w3050 w3072 w3096 w3115 w3133 w3151 w3169 w3183 w3197 w3216 w3230 w3245 w3262 w3272 w3276]
      tunnel: [w203 w564 w573 w579 w585 w607 w620 w660 w691 w709 w732 w770 w788 w794 w819 w843 w868 w891 w953 w981 w1013 w1036 w1043 w1053 w1075 errorcluster {"status"=FALSE, "code"=0, "source"=""} ("error out") w1106 w1112 w1125 w1144 w1158 w1181 w1238 w1243 w1249 w1256 w1283 w1309 w1332 w1335 w1380 w1411 w1425 w1449 w1459 w1474 w1480 w1504 w1527 w1545 w1558 w1594 w1606 w1617 w1621 w1636 w1665 w1677 w1695 w1715 w1732 w1761 w1765 w1783 w1798 w1810 w1822 w1845 w1860 w1873 w1876 w1893 w1901 w1909 w1917 w1921 w1930 w1940 w1943 w1952 w1967 w1988 w2007 w2018 w2036 w2058 w2074 w2081 w2089 w2097 w2102 w2109 w2117 w2125 w2132 w2142 w2170 w2178 w2185 w2193 w2198 w2206 w2212 w2219 w2227 w2244 w2249 w2254 w2267 w2338 w2346 w2358 w2368 w2381 w2401 w2425 w2434 w2447 w2471 w2497 w2503 w2511 w2533 w2549 w2555 w2560 w2567 w2577 w2589 w2598 w2603 w2615 w2620 w2630 w2638 w2646 w2651 w2656 w2661 w2671 w2683 w2705 w2717 w2721 w2735 w2761 w2782 w2795 w2799 w2858 w2906 w2952 w2960 w2980 w3000 w3014 w3028 w3034 w3052 w3074 w3098 w3117 w3135 w3153 w3171 w3185 w3199 w3218 w3232 w3246 w3263 w3270 w3277] -> w182
      tunnel: w183 -> [w209 w564 w573 w579 w585 w607 w620 w660 w691 w709 w730 w771 w788 w795 w828 w843 w858 w891 w953 w982 w1016 w1037 w1043 w1052 w1075 w1079 w1106 w1112 w1125 w1144 w1157 w1193 w1238 w1243 w1249 w1260 w1287 w1313 w1332 w1342 w1383 w1410 w1424 w1449 w1461 w1474 w1479 w1505 w1530 w1551 w1563 w1593 w1606 w1614 w1624 w1635 w1664 w1680 w1694 w1714 w1731 w1761 w1771 w1784 w1797 w1809 w1821 w1844 w1861 w1873 w1880 w1888 w1901 w1909 w1917 w1920 w1929 w1940 w1944 w1953 w1972 w1987 w2006 w2017 w2042 w2057 w2073 w2081 w2089 w2097 w2102 w2109 w2117 w2125 w2132 w2142 w2170 w2178 w2185 w2193 w2198 w2206 w2212 w2219 w2227 w2244 w2249 w2255 w2268 w2338 w2347 w2357 w2364 w2380 w2402 w2425 w2434 w2442 w2474 w2497 w2503 w2516 w2532 w2549 w2555 w2560 w2567 w2577 w2589 w2598 w2603 w2615 w2620 w2630 w2638 w2646 w2651 w2656 w2661 w2671 w2682 w2704 w2717 w2720 w2734 w2766 w2787 w2795 _ w2859 w2906 w2952 w2959 w2979 w2999 w3013 w3028 w3033 w3051 w3073 w3097 w3116 w3134 w3152 w3170 w3184 w3198 w3217 w3231 w3244 w3263 w3269 w3277]
      tunnel: [w211 w565 w574 w580 w586 w608 w621 w661 w695 w710 w739 w777 w789 w813 w841 w853 w879 w892 w958 w991 w1026 w1039 w1044 w1050 w1077 w1085 w1108 w1113 w1126 w1145 w1173 w1201 w1239 w1244 w1250 w1276 w1302 w1328 w1333 w1350 w1397 w1419 w1435 w1450 w1470 w1475 w1487 w1516 w1540 w1552 w1590 w1601 w1607 w1618 w1630 w1661 w1674 w1688 w1703 w1722 w1757 w1762 w1776 w1786 w1802 w1814 w1826 w1854 w1869 w1874 w1885 w1897 w1902 w1910 w1918 w1927 w1936 w1941 w1949 w1958 w1976 w1992 w2012 w2023 w2045 w2060 w2077 w2082 w2090 w2098 w2103 w2111 w2118 w2126 w2133 w2143 w2171 w2179 w2186 w2194 w2199 w2207 w2214 w2220 w2229 w2245 w2250 w2257 w2269 w2339 w2351 w2360 w2377 w2386 w2409 w2426 w2437 w2450 w2475 w2498 w2504 w2520 w2542 w2550 w2556 w2561 w2568 w2578 w2590 w2599 w2604 w2616 w2621 w2631 w2639 w2647 w2652 w2657 w2662 w2672 w2694 w2713 w2718 w2729 w2750 w2772 w2791 w2796 w2811 w2862 w2908 w2953 w2964 w2982 w3002 w3016 w3029 w3037 w3054 w3076 w3100 w3119 w3137 w3155 w3173 w3187 w3201 w3220 w3234 w3249 w3264 w3273 w3278] -> w199
      tunnel: [_ _ _ _ _ _ _ _ _ _ _ _ _ _ _ _ _ _ _ _ _ _ _ _ _ _ TRUE _ _ _ _ _ _ _ _ _ _ _ _ _ _ _ _ _ _ _ _ _ _ _ _ _ _ _ _ _ _ _ _ _ _ _ _ _ _ _ _ _ _ _ _ _ _ _ _ _ _ _ _ _ _ _ _ _ _ _ _ _ _ _ _ _ _ _ _ _ _ _ _ _ _ _ _ _ _ _ _ _ _ _ _ _ _ _ _ _ _ _ _ _ _ _ _ _ _ _ _ _ _ _ _ _ _ _ _ _ _ _ _ _ _ _ _ _ _ _ _ _ _ _ _ _ _ _ _ _ _ _ _ _ _ _ _ _ _ _ _ _ _ _ _ _ _] -> w190
      tunnel: [w208 w563 w571 w578 w584 w606 w619 w635 w693 w701 w736 w774 w786 w806 w832 w851 w877 w890 w918 w985 w1015 w1035 w1042 w1049 w1076 w1083 w1107 w1111 w1116 w1137 w1167 w1195 w1237 w1242 w1248 w1255 w1282 w1308 w1331 w1344 w1389 w1417 w1422 w1448 w1469 w1473 w1478 w1506 w1531 w1550 w1570 w1600 w1605 w1615 w1627 w1645 w1670 w1681 w1699 w1716 w1741 w1760 w1774 w1781 w1800 w1812 w1824 w1843 w1859 w1872 w1884 w1896 w1900 w1906 w1913 w1925 w1934 w1939 w1947 w1957 w1965 w1986 w1995 w2019 w2044 w2055 w2076 w2080 w2085 w2093 w2101 w2110 w2116 w2124 w2131 w2141 w2169 w2177 w2184 w2192 w2197 w2202 w2213 w2218 w2224 w2243 w2248 w2256 w2266 w2337 w2343 w2356 w2376 w2385 w2400 w2424 w2435 w2446 w2470 w2496 w2502 w2515 w2539 w2548 w2554 w2559 w2566 w2574 w2587 w2597 w2602 w2614 w2619 w2625 w2637 w2645 w2650 w2655 w2660 w2670 w2693 w2712 w2716 w2728 w2749 w2771 w2790 w2794 w2810 w2856 w2905 w2951 w2961 w2978 w2998 w3012 w3026 w3032 w3050 w3072 w3096 w3115 w3133 w3151 w3169 w3183 w3197 w3216 w3230 w3247 w3262 w3272 w3276] -> w198
      tunnel: 30 ("Timeout") -> [w207 _ _ _ _ _ _ _ _ _ _ _ _ _ _ _ _ _ _ _ _ _ _ _ _ _ _ _ _ _ _ _ _ _ _ _ _ _ _ _ _ _ _ _ _ _ _ _ _ _ _ _ _ _ _ _ _ _ _ _ _ _ _ _ _ _ _ _ _ _ _ _ _ _ _ _ _ _ _ _ _ _ _ _ _ _ _ _ _ _ _ _ _ _ _ _ _ _ _ _ _ _ _ _ _ _ _ _ _ _ _ _ _ _ _ _ _ _ _ _ _ _ _ _ _ _ _ _ _ _ _ _ _ _ _ _ _ _ _ _ _ _ _ _ _ _ _ _ _ _ _ _ _ _ _ _ _ _ _ _ _ _ _ _ _ _ _ _ _ _ _ _ _]
      tunnel: w195 -> [_ _ _ _ _ _ _ _ _ _ _ _ _ _ _ _ _ _ _ w989 _ _ _ _ _ _ _ _ _ _ _ _ _ _ _ _ _ _ _ _ _ _ _ _ _ _ _ _ _ _ _ _ _ _ _ _ _ _ _ _ _ _ _ _ _ _ _ _ _ _ w1881 w1892 _ _ _ _ _ _ _ _ _ _ _ _ _ _ _ _ _ _ _ _ _ _ _ _ _ _ _ _ _ _ _ _ _ _ _ _ _ _ _ _ _ _ _ _ _ _ _ _ _ _ _ _ _ _ _ _ _ _ _ _ _ _ _ _ _ _ _ _ _ _ _ _ _ _ _ _ _ _ _ _ _ _ _ _ _ _ _ _ _ _ _ _ _ _ _ _ _ _ _ _ _]
      tunnel: w194 -> [_ _ _ _ _ _ _ _ _ _ _ _ _ _ _ _ _ _ _ w988 _ _ _ _ _ _ _ _ _ _ _ _ _ _ _ _ _ _ _ _ _ _ _ _ _ _ _ _ _ _ _ _ _ _ _ _ _ _ _ _ _ _ _ _ _ _ _ _ _ _ w1882 w1891 _ _ _ _ _ _ _ _ _ _ _ _ _ _ _ _ _ _ _ _ _ _ _ _ _ _ _ _ _ _ _ _ _ _ _ _ _ _ _ _ _ _ _ _ _ _ _ _ _ _ _ _ _ _ _ _ _ _ _ _ _ _ _ _ _ _ _ _ _ _ _ _ _ _ _ _ _ _ _ _ _ _ _ _ _ _ _ _ _ _ _ _ _ _ _ _ _ _ _ _ _]
      tunnel: w193 -> [w206 _ _ _ _ _ _ _ _ _ _ _ _ _ _ _ _ _ _ _ _ _ _ _ _ _ _ _ _ _ _ _ _ _ _ _ _ _ _ _ _ w1413 _ _ _ _ _ _ _ _ _ _ _ _ _ _ _ _ _ _ _ _ _ _ _ _ _ _ _ _ _ _ _ _ _ _ _ _ _ _ _ _ _ _ _ _ _ _ _ _ _ _ _ _ _ _ _ _ _ _ _ _ _ _ _ _ _ _ _ _ _ _ _ _ _ _ _ _ _ _ _ _ _ _ _ _ _ _ _ _ _ _ _ _ _ _ _ _ _ _ _ _ _ _ _ _ _ _ _ _ _ _ _ _ _ _ _ _ _ _ _ _ _ _ _ _ _ _ _ _ _ _ _]
      tunnel: w192 -> [w205 w562 w572 w577 w583 w598 w618 w645 w694 w708 w738 w776 w787 w812 w840 w852 w878 w889 w957 w990 w1025 w1034 w1041 w1046 w1063 w1082 w1105 w1110 w1124 w1143 w1172 w1192 w1235 w1241 w1247 w1254 w1281 w1307 w1330 w1339 w1363 w1418 w1434 w1447 w1456 w1472 w1486 w1515 w1539 w1544 w1589 w1592 w1604 w1611 w1620 w1632 w1663 w1679 w1693 w1713 w1728 w1759 w1775 w1785 w1801 w1813 w1825 w1853 w1856 w1871 w1883 w1890 w1899 w1908 w1916 w1923 w1932 w1938 w1948 w1951 w1963 w1981 w1996 w2015 w2041 w2059 w2075 w2079 w2087 w2095 w2100 w2108 w2115 w2123 w2130 w2140 w2168 w2176 w2183 w2188 w2196 w2205 w2211 w2217 w2226 w2238 w2247 w2252 w2263 w2336 w2341 w2353 w2363 w2379 w2408 w2423 w2436 w2448 w2472 w2492 w2500 w2513 w2541 w2546 w2552 w2558 w2565 w2576 w2588 w2596 w2601 w2613 w2618 w2629 w2636 w2644 w2649 w2654 w2659 w2669 w2692 w2711 w2715 w2727 w2748 w2770 w2789 w2793 w2809 w2861 w2907 w2948 w2963 w2981 w3001 w3015 w3027 w3036 w3053 w3075 w3099 w3118 w3136 w3154 w3172 w3186 w3200 w3219 w3233 w3248 w3261 w3271 w3275]
      tunnel: [w204 w562 w572 w577 w583 w598 w618 w645 w694 w708 w738 w776 w787 w812 w840 w852 w878 w889 w957 w990 w1025 w1034 w1041 w1046 w1063 w1082 w1105 w1110 w1124 w1143 w1172 w1192 w1235 w1241 w1247 w1254 w1281 w1307 w1330 w1339 w1363 w1418 w1434 w1447 w1456 w1472 w1486 w1515 w1539 w1544 w1589 w1592 w1604 w1611 w1620 w1632 w1663 w1679 w1693 w1713 w1728 w1759 w1775 w1785 w1801 w1813 w1825 w1853 w1856 w1871 w1883 w1890 w1899 w1908 w1916 w1923 w1932 w1938 w1948 w1951 w1963 w1981 w1996 w2015 w2041 w2059 w2075 w2079 w2087 w2095 w2100 w2108 w2115 w2123 w2130 w2140 w2168 w2176 w2183 w2188 w2196 w2205 w2211 w2217 w2226 w2238 w2247 w2252 w2263 w2336 w2341 w2353 w2363 w2379 w2408 w2423 w2436 w2448 w2472 w2492 w2500 w2513 w2541 w2546 w2552 w2558 w2565 w2576 w2588 w2596 w2601 w2613 w2618 w2629 w2636 w2644 w2649 w2654 w2659 w2669 w2692 w2711 w2715 w2727 w2748 w2770 w2789 w2793 w2809 w2861 w2907 w2948 w2963 w2981 w3001 w3015 w3027 w3036 w3053 w3075 w3099 w3118 w3136 w3154 w3172 w3186 w3200 w3219 w3233 w3248 w3261 w3271 w3275] -> w191
      tunnel: w187 -> [_ _ _ _ _ _ _ _ _ _ _ _ _ _ _ _ _ _ _ w983 _ _ _ _ _ _ _ _ _ _ _ _ _ _ _ _ _ _ _ _ _ _ _ _ _ _ _ _ _ _ _ _ _ _ _ _ _ _ _ _ _ _ _ _ _ _ _ _ _ _ w1878 w1889 _ _ _ _ _ _ _ _ _ _ _ _ _ _ _ _ _ _ _ _ _ _ _ _ _ _ _ _ _ _ _ _ _ _ _ _ _ _ _ _ _ _ _ _ _ _ _ _ _ _ _ _ _ _ _ _ _ _ _ _ _ _ _ _ _ _ _ _ _ _ _ _ _ _ _ _ _ _ _ _ _ _ _ _ _ _ _ _ _ _ _ _ _ _ _ _ _ _ _ _ _]
      frame "", "Event Structure", "Idle" {
        # "executes when the state queue is empty"
        n82 = event shown="[2] \"355nm Laser toggle\": Value Change" {
          selector: w205 -> [_ _ _ _ _ _ _ _ _ _ _ _ _ _ _ _ _ _ _ _ _ _ _ _ _ _ _ _ _ _ _ _ _ _ _]
          dyn-events: [_ _ _ _ _ _ _ _ _ _ _ _ _ _ _ _ _ _ _ _ _ _ _ _ _ _ _ _ _ _ _ _ _ _ _] -> w204
          timeout: w207 -> [_ _ _ _ _ _ _ _ _ _ _ _ _ _ _ _ _ _ _ _ _ _ _ _ _ _ _ _ _ _ _ _ _ _ _]
          tunnel: w212 -> [w232 w251 w259 w263 w267 w275 w281 w289 w299 w306 w331 w347 w363 w367 w374 w397 w411 w425 w430 w433 w439 w446 w453 w459 w465 w471 w478 w491 w502 w514 w521 w525 w529 w545 w561]
          tunnel: [w233 w251 w258 w263 w266 w275 w281 w289 w299 w305 w331 w347 w363 w367 w373 w397 w411 w425 w429 w432 w439 w447 w454 w458 w464 w471 w479 w492 w502 w515 w521 w525 w528 w546 w560] -> w211
          tunnel: w210 -> [w216 w249 w253 w261 w268 w274 w282 w290 w297 w301 w329 w345 w361 w365 w369 w396 w410 w424 w426 w434 w437 w442 w449 w461 w466 w469 w473 w486 w500 w510 w519 w523 w530 w543 w558]
          tunnel: [w231 w250 w254 w262 w269 w273 w280 w288 w298 w307 w330 w346 w362 w366 w375 w394 w398 w421 w428 w435 w438 w443 w450 w462 w467 w470 w477 w490 w501 w511 w520 w524 w531 w547 w559] -> w203
          tunnel: w209 -> [w231 w250 w254 w262 w269 w273 w280 w288 w298 w307 w330 w346 w362 w366 w375 w391 w400 w412 w428 w435 w438 w443 w450 w462 w467 w470 w477 w490 w501 w513 w520 w524 w531 w547 w559]
          tunnel: [w216 w249 w253 w261 w268 w274 w282 w290 w297 w302 w329 w345 w361 w365 w370 w396 w410 w424 w426 w434 w437 w444 w451 w461 w466 w469 w474 w487 w500 w516 w519 w523 w530 w544 w558] -> w208
          tunnel: w206 -> [_ _ _ _ _ _ _ _ _ _ _ _ _ _ _ _ _ _ _ _ _ _ _ _ _ _ _ _ _ _ _ _ _ _ _]
          event Timeout {
            # "check system status every 2s"
            n83 = event-data() -> ()  [unwired: 1 in, 1 out]
            n84 = Unbundle By Name(w216) -> ("SysRunning?"=w214:bool, "SlowTimer"=w230:u32, "FastTimer"=w224:u32)
            n85 = Tick Count (ms)() -> (millisecond timer value=w217:u32)
            n86 = Subtract(x=w217, y=w230) -> (x-y=w227:u32)
            n87 = case shown="False" w214 {
              tunnel: ["" "Utility: AquiTimerCheck" ("State(s) in Front (\"\")")] -> w222
              frame False {
                # "if not running, do nothing"
              }
              frame True {
                # "if aquisition is running, check timer"
              }
            }
            n88 = Subtract(x=w217, y=w224) -> (x-y=w225:u32)
            n89 = Greater?(x=w227, y=u32 2000) -> (0:w228:bool)
            n90 = Greater?(x=w225, y=u32 500) -> (0:w215:bool)
            n91 = disable-structure shown="Enabled" {
              disable-tunnel: w215 -> [w238 _]
              disable-tunnel: w214 -> [w237 _]
              disable-tunnel: [w234 "" ("State(s) at Back (\"\")")] -> w213
              frame Disabled {
                n92 = Not(x=w237) -> (.not. x?=w236:bool)
                n93 = And(x=w238, y=w236) -> (x .and. y?=w235:bool)
                n94 = case shown="True" w235 {
                  tunnel: ["" ("Empty String Constant") "TCP: checkSource" ("State(s) in Front (\"\")")] -> w234
                  frame False {
                  }
                  frame True {
                  }
                }
              }
              frame Enabled {
              }
            }
            n95 = case shown="True" w228 {
              tunnel: ["" ("Empty String Constant") "SystemStatus: SlowSysStatusMacro" ("State(s) in Front (\"\")")] -> w220
              frame False {
              }
              frame True {
              }
            }
            n96 = case shown="True" w215 {
              tunnel: ["" ("Empty String Constant") "SystemStatus: FastSysStatusMacro" ("State(s) in Front (\"\")")] -> w218
              frame False {
              }
              frame True {
              }
            }
            n97 = call <vilib>:"Add State(s) to Queue__JKI_lib_State_Machine.vi"("State(s) in Front (\"\")"=w222, "State(s) in (\"\")"="LabJack: checkPedal" ("State(s) in Front (\"\")"), "State(s) at Back (\"\")"=w220) -> ("States Out"=w219:string)  [unwired: 12 in]
            n98 = call <vilib>:"Add State(s) to Queue__JKI_lib_State_Machine.vi"("State(s) in Front (\"\")"=w219, "State(s) in (\"\")"=w218, "State(s) at Back (\"\")"=w213) -> ("States Out"=w223:string)  [unwired: 12 in]
            n99 = call <vilib>:"Add State(s) to Queue__JKI_lib_State_Machine.vi"("State(s) in Front (\"\")"=w223, "State(s) in (\"\")"=w232) -> ("States Out"=w233:string)  [unwired: 13 in]
          }
          event "355nm Laser toggle": Mouse Enter {
            n100 = event-data() -> ()  [unwired: 1 in, 4 out]
            n101 = local write "Help"("Toggle 355nm laser." ("Help")) -> ()
          }
          event "355nm Laser toggle": Value Change {
            # "[Covers: REQ34]"
            n102 = event-data() -> ()  [unwired: 1 in, 6 out]
            n103 = Select(t="LabJack: 355_PWM_Start\nLabJack: AB_Start", s="355nm Laser toggle", f="LabJack: 355_PWM_Stop\nLabJack: AB_Stop") -> (s? t:f=w256:string)
            n104 = call <vilib>:"Add State(s) to Queue__JKI_lib_State_Machine.vi"("State(s) in Front (\"\")"=w256, "State(s) in (\"\")"=w259) -> ("States Out"=w258:string)  [unwired: 13 in]
          }
          event "Aiming beam toggle": Mouse Enter {
            n105 = event-data() -> ()  [unwired: 1 in, 4 out]
            n106 = local write "Help"("Toggle aiming beam laser." ("Help")) -> ()
          }
          event "Aiming beam toggle": Value Change {
            # "[Covers: REQ33]"
            n107 = event-data() -> ()  [unwired: 1 in, 6 out]
            n108 = case shown="True" "Aiming beam toggle" {
              tunnel: ["LabJack: AB_Stop" ("State(s) in Front (\"\")") "LabJack: AB_Start" ("State(s) in Front (\"\")")] -> w265
              frame False {
              }
              frame True {
              }
            }
            n109 = call <vilib>:"Add State(s) to Queue__JKI_lib_State_Machine.vi"("State(s) in Front (\"\")"=w265, "State(s) in (\"\")"=w267) -> ("States Out"=w266:string)  [unwired: 13 in]
          }
          event "Auto gain ch1": Value Change {
            n110 = event-data() -> ("NewVal"=w272:bool)  [unwired: 1 in, 5 out]
            n111 = case shown="True" w272 {
              frame False {
                n112 = local read "V 1"() -> (w276:dbl)
                n113 = call "V1FGV.vi"("action (write)"=enum16{"write", "read"}."write" ("action"), "V1 in"=w276) -> ()  [unwired: 8 in, 2 out]
                n114 = property on="V 1" class="DigNum (strict)"("DisabledEnum"=T10."Enabled" ("Disabled")) -> ()  [unwired: 2 in, 2 out]
              }
              frame True {
                n115 = property on="V 1" class="DigNum (strict)"("DisabledEnum"=T10."Disabled and Grayed Out" ("Disabled")) -> ()  [unwired: 2 in, 2 out]
              }
            }
          }
          event "Auto gain ch2": Value Change {
            n116 = event-data() -> ("NewVal"=w283:bool)  [unwired: 1 in, 5 out]
            n117 = case shown="False" w283 {
              frame False {
                n118 = local read "V 2"() -> (w284:dbl)
                n119 = property on="V 2" class="DigNum (strict)"("DisabledEnum"=T10."Enabled" ("Disabled")) -> ()  [unwired: 2 in, 2 out]
                n120 = call "V2FGV.vi"("action(write)"=enum16{"write", "read"}."write" ("action"), "V2 in"=w284) -> ()  [unwired: 8 in, 2 out]
              }
              frame True {
                n121 = property on="V 2" class="DigNum (strict)"("DisabledEnum"=T10."Disabled and Grayed Out" ("Disabled")) -> ()  [unwired: 2 in, 2 out]
              }
            }
          }
          event "Auto gain ch3": Value Change {
            n122 = event-data() -> ("NewVal"=w291:bool)  [unwired: 1 in, 5 out]
            n123 = case shown="False" w291 {
              frame False {
                n124 = local read "V 3"() -> (w292:dbl)
                n125 = property on="V 3" class="DigNum (strict)"("DisabledEnum"=T10."Enabled" ("Disabled")) -> ()  [unwired: 2 in, 2 out]
                n126 = call "V3FGV.vi"("action(write)"=enum16{"write", "read"}."write" ("action"), "V3 in"=w292) -> ()  [unwired: 8 in, 2 out]
              }
              frame True {
                n127 = property on="V 3" class="DigNum (strict)"("DisabledEnum"=T10."Disabled and Grayed Out" ("Disabled")) -> ()  [unwired: 2 in, 2 out]
              }
            }
          }
          event "Background": Mouse Enter {
            n128 = event-data() -> ()  [unwired: 1 in, 4 out]
            n129 = local write "Help"("Click to record a background." ("Help")) -> ()
          }
          event "Background": Value Change {
            n130 = event-data() -> ("NewVal"=w303:bool)  [unwired: 1 in, 5 out]
            n131 = case shown="True" w303 {
              tunnel: ["Utility: SetAllChanManualGain\nQueue: Flash\nUtility: Dewelling >> 2500\nLabJack: 355_PWM_Stop\nLabJack: AB_Stop" "Utility: SetDataClass >> Bg\nUI: Update\nLabJack: 355_PWM_Start\nLabJack: AB_Start\nUtility: SaveDeconChan\nUtility: Dewelling >> 50\nLabJack: SetV\nDigitizer: Start\nUtility: AquiTimerReset\nLED: BreathGreen\nUI: duringBGAcquire"] -> w304
              tunnel: [FALSE TRUE] -> w300
              frame False {
                n132 = local read "Skip Data Save?"() -> (w308:bool)
                n133 = case shown="False" w308 {
                  frame False {
                    n134 = property on="Background" class="Bool (strict)"("BoolText.Text"="Done!" ("Boolean Text.Text")) -> ()  [unwired: 2 in, 2 out]
                  }
                  frame True {
                  }
                }
              }
              frame True {
                # "[Covers: REQ6]"
                n135 = property on="Background" class="Bool (strict)"("BoolText.Text"="Running" ("Boolean Text.Text"), "Colors [4]"=cluster{u32, u32}[] [{6618880, 6618880}, {16711680, 16711680}]) -> ()  [unwired: 2 in, 2 out]
              }
            }
            n136 = Bundle By Name(cluster=w301, "SysRunning?"=w300) -> (w302:T25)
            n137 = call <vilib>:"Add State(s) to Queue__JKI_lib_State_Machine.vi"("State(s) in Front (\"\")"=w304, "State(s) in (\"\")"=w306) -> ("States Out"=w305:string)  [unwired: 13 in]
          }
          event "Channel 1": Cursor Move {
            n138 = event-data() -> ("CursIdx"=w320:i32, "CursLoc"=w327:cluster{"X":dbl, "Y":dbl})  [unwired: 1 in, 7 out]
            n139 = Unbundle By Name(w327) -> ("X"=w325:dbl)
            n140 = property on="Channel 2" class="WFGraph (strict)"() -> ("CrsrList"=w324:T26)  [unwired: 2 in, 2 out]
            n141 = property on="Channel 3" class="WFGraph (strict)"() -> ("CrsrList"=w321:T26)  [unwired: 2 in, 2 out]
            n142 = Index Array(array=w324, index=w320) -> (element=w328:T27)
            n143 = Index Array(array=w321, index=w320) -> (element=w326:T27)
            n144 = Bundle By Name(cluster=w326, "Position.X"=w325) -> (w319:T27)
            n145 = Bundle By Name(cluster=w328, "Position.X"=w325) -> (w323:T27)
            n146 = control-ref of="Channel 1"() -> (w316:refnum<vi>)
            n147 = Replace Array Subset(array=w324, new element=w323, index=w320) -> (w322:T26)
            n148 = Replace Array Subset(array=w321, new element=w319, index=w320) -> (w318:T26)
            n149 = property on="Channel 2" class="WFGraph (strict)"("CrsrList"=w322) -> ()  [unwired: 2 in, 2 out]
            n150 = property on="Channel 3" class="WFGraph (strict)"("CrsrList"=w318) -> (error out=w317:errorcluster)  [unwired: 2 in, 1 out]
            n151 = call "UpdateCurserIdx(SubVI).vi"("error in (no error)"=w317, "WaveformGraph in"=w316) -> ()  [unwired: 9 in, 1 out]
          }
          event "Channel 2": Cursor Move {
            n152 = event-data() -> ("CursIdx"=w338:i32, "CursLoc"=w344:cluster{"X":dbl, "Y":dbl})  [unwired: 1 in, 7 out]
            n153 = Unbundle By Name(w344) -> ("X"=w341:dbl)
            n154 = property on="Channel 1" class="WFGraph (strict)"() -> ("CrsrList"=w336:T26)  [unwired: 2 in, 2 out]
            n155 = property on="Channel 3" class="WFGraph (strict)"() -> ("CrsrList"=w339:T26)  [unwired: 2 in, 2 out]
            n156 = Index Array(array=w336, index=w338) -> (element=w343:T27)
            n157 = Index Array(array=w339, index=w338) -> (element=w342:T27)
            n158 = Bundle By Name(cluster=w343, "Position.X"=w341) -> (w340:T27)
            n159 = Bundle By Name(cluster=w342, "Position.X"=w341) -> (w337:T27)
            n160 = Replace Array Subset(array=w336, new element=w340, index=w338) -> (w335:T26)
            n161 = Replace Array Subset(array=w339, new element=w337, index=w338) -> (w334:T26)
            n162 = control-ref of="Channel 1"() -> (w333:refnum<vi>)
            n163 = property on="Channel 1" class="WFGraph (strict)"("CrsrList"=w335) -> ()  [unwired: 2 in, 2 out]
            n164 = property on="Channel 3" class="WFGraph (strict)"("CrsrList"=w334) -> (error out=w332:errorcluster)  [unwired: 2 in, 1 out]
            n165 = call "UpdateCurserIdx(SubVI).vi"("error in (no error)"=w332, "WaveformGraph in"=w333) -> ()  [unwired: 9 in, 1 out]
          }
          event "Channel 3": Cursor Move {
            n166 = event-data() -> ("CursIdx"=w353:i32, "CursLoc"=w360:cluster{"X":dbl, "Y":dbl})  [unwired: 1 in, 7 out]
            n167 = Unbundle By Name(w360) -> ("X"=w357:dbl)
            n168 = property on="Channel 1" class="WFGraph (strict)"() -> ("CrsrList"=w356:T26)  [unwired: 2 in, 2 out]
            n169 = property on="Channel 2" class="WFGraph (strict)"() -> ("CrsrList"=w354:T26)  [unwired: 2 in, 2 out]
            n170 = Index Array(array=w356, index=w353) -> (element=w359:T27)
            n171 = Index Array(array=w354, index=w353) -> (element=w358:T27)
            n172 = Bundle By Name(cluster=w359, "Position.X"=w357) -> (w355:T27)
            n173 = Bundle By Name(cluster=w358, "Position.X"=w357) -> (w352:T27)
            n174 = Replace Array Subset(array=w356, new element=w355, index=w353) -> (w351:T26)
            n175 = Replace Array Subset(array=w354, new element=w352, index=w353) -> (w350:T26)
            n176 = control-ref of="Channel 1"() -> (w348:refnum<vi>)
            n177 = property on="Channel 1" class="WFGraph (strict)"("CrsrList"=w351) -> ()  [unwired: 2 in, 2 out]
            n178 = property on="Channel 2" class="WFGraph (strict)"("CrsrList"=w350) -> (error out=w349:errorcluster)  [unwired: 2 in, 1 out]
            n179 = call "UpdateCurserIdx(SubVI).vi"("error in (no error)"=w349, "WaveformGraph in"=w348) -> ()  [unwired: 9 in, 1 out]
          }
          event "Cali&iRF alignment": Mouse Enter {
            n180 = event-data() -> ()  [unwired: 1 in, 4 out]
            n181 = local write "Help"("Click to run system intensity calibration and irf alignment" ("Help")) -> ()
          }
          event "Cali&iRF alignment": Value Change {
            n182 = event-data() -> ("NewVal"=w371:bool)  [unwired: 1 in, 5 out]
            n183 = case shown="False" w371 {
              tunnel: ["Utility: SetAllChanManualGain\nQueue: Flash\nUtility: Dewelling >> 2500\nLabJack: 355_PWM_Stop\nLabJack: AB_Stop" "Utility: SetDataClass >> Cali\nUI: Update\nUtility: SaveDeconChan\nLabJack: 355_PWM_Start\nLabJack: AB_Start\nLabJack: SetV\nDigitizer: Start\nUtility: AquiTimerReset\nLED: BreathGreen\nUI: duringIRFAlign"] -> w372
              tunnel: [FALSE TRUE] -> w368
              frame False {
                n184 = local read "Skip Data Save?"() -> (w376:bool)
                n185 = case shown="False" w376 {
                  frame False {
                    n186 = property on="Cali&iRF alignment" class="Bool (strict)"("BoolText.Text"="Done!" ("Boolean Text.Text")) -> ()  [unwired: 2 in, 2 out]
                  }
                  frame True {
                  }
                }
              }
              frame True {
                n187 = property on="Cali&iRF alignment" class="Bool (strict)"("BoolText.Text"="Running" ("Boolean Text.Text"), "Colors [4]"=cluster{u32, u32}[] [{6618880, 6618880}, {16711680, 16711680}]) -> ()  [unwired: 2 in, 2 out]
              }
            }
            n188 = Bundle By Name(cluster=w369, "SysRunning?"=w368) -> (w370:T25)
            n189 = call <vilib>:"Add State(s) to Queue__JKI_lib_State_Machine.vi"("State(s) in Front (\"\")"=w372, "State(s) in (\"\")"=w374) -> ("States Out"=w373:string)  [unwired: 13 in]
          }
          event "V 1": Value Change {
            n190 = event-data() -> ()  [unwired: 1 in, 6 out]
            n191 = call "LabJack_FGV.vi"("Operation(Read)"=enum16{"Write", "Read"}."Read" ("Operation"), "error in (no error)"=w391) -> ("error out"=w388:errorcluster, "Read data"=w389:i32)  [unwired: 8 in]
            n192 = global read "GlobalVariables.vi" "Ch1 LJ pin"() -> (w387:string)
            n193 = call "LJM_eWriteName.vi"("Handle In"=w389, "Name"=w387, "Value"="V 1", "error in"=w388) -> ("error out"=w385:errorcluster)  [unwired: 10 in, 1 out]
            n194 = call "V1FGV.vi"("Error In"=w385, "action (write)"=enum16{"write", "read"}."write" ("action"), "V1 in"="V 1") -> ("Error Out"=w384:errorcluster)  [unwired: 7 in, 1 out]
            n195 = call "CtrlVtoGain.vi"("error in (no error)"=w384, "CtrlV(V)"="V 1", "Channel"=enum16{"Ch1", "Ch2", "Ch3"}."Ch1" ("Enum")) -> ("error out"=w394:errorcluster, "Gain"=w393:dbl)  [unwired: 7 in]
            n196 = local write "Gain1"(w393) -> ()
          }
          event "V 2": Value Change {
            n197 = event-data() -> ()  [unwired: 1 in, 6 out]
            n198 = call "LabJack_FGV.vi"("Operation(Read)"=enum16{"Write", "Read"}."Read" ("Operation"), "error in (no error)"=w400) -> ("error out"=w405:errorcluster, "Read data"=w406:i32)  [unwired: 8 in]
            n199 = global read "GlobalVariables.vi" "Ch2 LJ pin"() -> (w404:string)
            n200 = call "LJM_eWriteName.vi"("Handle In"=w406, "Name"=w404, "Value"="V 2", "error in"=w405) -> ("error out"=w403:errorcluster)  [unwired: 10 in, 1 out]
            n201 = call "V2FGV.vi"("Error In"=w403, "action(write)"=enum16{"write", "read"}."write" ("action"), "V2 in"="V 2") -> ("Error Out"=w402:errorcluster)  [unwired: 7 in, 1 out]
            n202 = call "CtrlVtoGain.vi"("error in (no error)"=w402, "CtrlV(V)"="V 2", "Channel"=enum16{"Ch1", "Ch2", "Ch3"}."Ch2" ("Enum")) -> ("error out"=w398:errorcluster, "Gain"=w399:dbl)  [unwired: 7 in]
            n203 = local write "Gain2"(w399) -> ()
          }
          event "V 3": Value Change {
            n204 = event-data() -> ()  [unwired: 1 in, 6 out]
            n205 = call "LabJack_FGV.vi"("Operation(Read)"=enum16{"Write", "Read"}."Read" ("Operation"), "error in (no error)"=w412) -> ("error out"=w417:errorcluster, "Read data"=w418:i32)  [unwired: 8 in]
            n206 = global read "GlobalVariables.vi" "Ch3 LJ pin"() -> (w416:string)
            n207 = call "LJM_eWriteName.vi"("Handle In"=w418, "Name"=w416, "Value"="V 3", "error in"=w417) -> ("error out"=w414:errorcluster)  [unwired: 10 in, 1 out]
            n208 = call "V3FGV.vi"("Error In"=w414, "action(write)"=enum16{"write", "read"}."write" ("action"), "V3 in"="V 3") -> ("Error Out"=w413:errorcluster)  [unwired: 7 in, 1 out]
            n209 = call "CtrlVtoGain.vi"("error in (no error)"=w413, "CtrlV(V)"="V 3", "Channel"=enum16{"Ch1", "Ch2", "Ch3"}."Ch3" ("Enum")) -> ("error out"=w421:errorcluster, "Gain"=w420:dbl)  [unwired: 7 in]
            n210 = local write "Gain3"(w420) -> ()
          }
          event "Quit": Value Change {
            # "Exit Button Value Change (pressed) Event\n(when pressed.  quite)"
            n211 = event-data() -> ()  [unwired: 1 in, 1 out]
            n212 = call <vilib>:"Add State(s) to Queue__JKI_lib_State_Machine.vi"("State(s) in Front (\"\")"="LED: Off\nMacro: Exit", "State(s) in (\"\")"=w430) -> ("States Out"=w429:string)  [unwired: 13 in]
          }
          event "Show BG": Value Change {
            n213 = event-data() -> ()  [unwired: 1 in, 6 out]
            n214 = call <vilib>:"Add State(s) to Queue__JKI_lib_State_Machine.vi"("State(s) in Front (\"\")"="Data: showBG" ("State(s) in Front (\"\")"), "State(s) in (\"\")"=w433) -> ("States Out"=w432:string)  [unwired: 13 in]
          }
          event "StartButton": Mouse Enter {
            n215 = event-data() -> ()  [unwired: 1 in, 4 out]
            n216 = local write "Help"("Press to start aquisition." ("Help")) -> ()
          }
          event "StartButton": Value Change {
            # "[Covers: REQ32]"
            # "start PWM before acquisition"
            # "Initialize both digitizer aquisition and\n send user event to trigger aquisition loop"
            n217 = event-data() -> ()  [unwired: 1 in, 6 out]
            n218 = local write "StartButton"(FALSE ("StartButton")) -> ()
            n219 = Bundle By Name(cluster=w442, "SysRunning?"=TRUE) -> (w444:T25)
            n220 = call <vilib>:"Add State(s) to Queue__JKI_lib_State_Machine.vi"("State(s) in Front (\"\")"="TCP: stopCam\nUtility: SetDataClass >> Data\nQueue: Flash\nUI: Update\nUtility: StartBeep\nLabJack: 355_PWM_Start\nLabJack: AB_Start\nLabJack: SetV\nDigitizer: Start\nUtility: AquiTimerReset\nUI: DuringAquisition\nLED: BreathGreen\nTCP: sendRunNum\nTCP: sendVideoSource\nTCP: sendChannel\nTCP: startRun", "State(s) in (\"\")"=w446) -> ("States Out"=w447:string)  [unwired: 13 in]
          }
          event User Event {
            # "[Covers: REQ32]"
            # "start PWM before acquisition"
            # "Initialize both digitizer aquisition and\n send user event to trigger aquisition loop"
            n221 = event-data() -> ()  [unwired: 1 in, 5 out]
            n222 = Bundle By Name(cluster=w449, "SysRunning?"=TRUE) -> (w451:T25)
            n223 = call <vilib>:"Add State(s) to Queue__JKI_lib_State_Machine.vi"("State(s) in Front (\"\")"="TCP: stopCam\nUtility: SetDataClass >> Data\nQueue: Flash\nUI: Update\nUtility: StartBeep\nLabJack: 355_PWM_Start\nLabJack: AB_Start\nLabJack: SetV\nDigitizer: Start\nUtility: AquiTimerReset\nUI: DuringAquisition\nLED: BreathGreen\nTCP: sendRunNum\nTCP: sendVideoSource\nTCP: sendChannel\nTCP: startRun", "State(s) in (\"\")"=w453) -> ("States Out"=w454:string)  [unwired: 13 in]
          }
          event "Video Display": Value Change {
            n224 = event-data() -> ("NewVal"=w460:bool)  [unwired: 1 in, 5 out]
            n225 = Select(t="TCP: startCam", s=w460, f="TCP: stopCam") -> (s? t:f=w457:string)
            n226 = call <vilib>:"Add State(s) to Queue__JKI_lib_State_Machine.vi"("State(s) in (\"\")"=w459, "State(s) at Back (\"\")"=w457) -> ("States Out"=w458:string)  [unwired: 13 in]
          }
          event "Video Source": Value Change {
            n227 = event-data() -> ()  [unwired: 1 in, 6 out]
            n228 = call <vilib>:"Add State(s) to Queue__JKI_lib_State_Machine.vi"("State(s) in Front (\"\")"="TCP: sendVideoSource" ("State(s) in Front (\"\")"), "State(s) in (\"\")"=w465) -> ("States Out"=w464:string)  [unwired: 13 in]
          }
          event "StopButton": Mouse Enter {
            n229 = event-data() -> ()  [unwired: 1 in, 4 out]
            n230 = local write "Help"("Press to stop data aquisition." ("Help")) -> ()
          }
          event "StopButton": Value Change {
            # "if system is running, send stop command, if not do nothing."
            # "stop aquisition\nupdate UI"
            n231 = event-data() -> ()  [unwired: 1 in, 6 out]
            n232 = Unbundle By Name(w473) -> ("SysRunning?"=w475:bool)
            n233 = case shown="True" w475 {
              tunnel: ["" ("Empty String Constant") "LabJack: AB_Stop\nLabJack: 355_PWM_Stop\n/*Digitizer: Abort"] -> w476
              tunnel: w473 -> [w480 w484]
              tunnel: [w480 w483] -> w474
              frame False {
              }
              frame True {
                n234 = Bundle By Name(cluster=w484, "SysRunning?"=FALSE) -> (w483:T25)
              }
            }
            n235 = call <vilib>:"Add State(s) to Queue__JKI_lib_State_Machine.vi"("State(s) in Front (\"\")"=w476, "State(s) in (\"\")"=w478) -> ("States Out"=w479:string)  [unwired: 13 in]
            n236 = local write "StopButton"(FALSE ("StopButton")) -> ()
          }
          event User Event {
            # "if system is running, send stop command, if not do nothing."
            # "stop aquisition\nupdate UI"
            n237 = event-data() -> ()  [unwired: 1 in, 5 out]
            n238 = Unbundle By Name(w486) -> ("SysRunning?"=w488:bool)
            n239 = case shown="True" w488 {
              tunnel: ["" ("Empty String Constant") "LabJack: AB_Stop\nLabJack: 355_PWM_Stop\n/*Digitizer: Abort"] -> w489
              tunnel: w486 -> [w493 w497]
              tunnel: [w493 w496] -> w487
              frame False {
              }
              frame True {
                n240 = Bundle By Name(cluster=w497, "SysRunning?"=FALSE) -> (w496:T25)
              }
            }
            n241 = call <vilib>:"Add State(s) to Queue__JKI_lib_State_Machine.vi"("State(s) in Front (\"\")"=w489, "State(s) in (\"\")"=w491) -> ("States Out"=w492:string)  [unwired: 13 in]
          }
          event "Sys Reconfig": Mouse Enter {
            n242 = event-data() -> ()  [unwired: 1 in, 4 out]
            n243 = local write "Help"("Click to reconfig digitizer settings." ("Help")) -> ()
          }
          event "Sys Reconfig": Value Change {
            # "everytime the user change data aquisition setting, need to reinitilize decon engine and realign iRF.\ncheck whether data length has changed, if changed, reinitialize Decon engine\nreset BG ready, need a new BG"
            # "update DAQ FGV"
            n244 = event-data() -> ()  [unwired: 1 in, 6 out]
            n245 = call "SystemConfigEditorV6.vi"("error in"=w513) -> ("error out"=w512:errorcluster, "FLImDAQ out"=w507:T6)  [unwired: 1 in]
            n246 = Unbundle By Name(w510) -> ("FLImDAQ.min record length"=w509:i32)
            n247 = Unbundle By Name(w507) -> ("min record length"=w508:i32)
            n248 = call "FLImDAQ_FGV.vi"("error in (no error)"=w512, "Operation (Read)"=enum16{"Write", "Read"}."Write" ("Operation"), "Write data"=w507) -> ("error out"=w511:errorcluster, "Read data"=w506:T6)  [unwired: 7 in]
            n249 = Equal?(x=w509, y=w508) -> (x = y?=w505:bool)
            n250 = case shown="False" w505 {
              tunnel: ["UI: Cursor Set >> Busy\nDigitizer: Config\nDeconEngine: InitializeCh1\nDeconEngine: InitializeCh2\nDeconEngine: InitializeCh3\nUI: CaliAndiRFNotReady\n/*UI iRF not ready\nUI: Update\nUI: Cursor Set >> Idle" "UI: Cursor Set >> Busy\nDigitizer: Config\nUI: Update\nUI: Cursor Set >> Idle"] -> w504
              frame False {
              }
              frame True {
              }
            }
            n251 = Bundle By Name(cluster=w510, "FLImDAQ"=w506) -> (w516:T25)
            n252 = call <vilib>:"Add State(s) to Queue__JKI_lib_State_Machine.vi"("State(s) in Front (\"\")"=w504, "State(s) in (\"\")"=w514) -> ("States Out"=w515:string)  [unwired: 13 in]
          }
          event "System Hardware Connection Status", "StartButton", "StopButton", "355nm Laser toggle", "Aiming beam toggle", "Cali&iRF alignment", "Background", "Sys Reconfig": Mouse Leave {
            n253 = event-data() -> ()  [unwired: 1 in, 4 out]
            n254 = invoke on="Help" class="Str" method="Reinit To Default"() -> ()  [unwired: 3 in, 3 out]
          }
          event "System Hardware Connection Status.Digitizer": Mouse Enter {
            n255 = event-data() -> ()  [unwired: 1 in, 4 out]
            n256 = local write "Help"("Status of hardware connections. TCP/IP is optional." ("Help")) -> ()
          }
          event "TCP Connect": Value Change {
            n257 = event-data() -> ("NewVal"=w526:bool)  [unwired: 1 in, 5 out]
            n258 = case shown="True" w526 {
              tunnel: ["TCP: Close\nUI: Update" ("State(s) in Front (\"\")") "TCP: SendSettingMacro\nUI: Update" ("State(s) in Front (\"\")")] -> w527
              frame False {
              }
              frame True {
              }
            }
            n259 = call <vilib>:"Add State(s) to Queue__JKI_lib_State_Machine.vi"("State(s) in Front (\"\")"=w527, "State(s) in (\"\")"=w529) -> ("States Out"=w528:string)  [unwired: 13 in]
          }
          event User Event {
            # "if aquisition loop is error out. Stop digitizer, update front panel indicator, stop both laser and \nOption 1: parse and save data\nOption 2: Flash queue if scout run. [Covers: REQ23]"
            n260 = event-data() -> ()  [unwired: 1 in, 5 out]
            n261 = case shown="\"BG\"" "Data Class" {
              tunnel: [w551 "UI: Cursor Set >> Busy\nUtility: SetAllChanAutoGain\nUtility: RestoreDeConChan\nData: parseRunData\nData: irfAlignment\nUI: Cursor Set >> Idle" "UI: Cursor Set >> Busy\nUtility: SetAllChanAutoGain\nUtility: RestoreDeConChan\nData: parseRunData\nData: saveBGtoFGV\nData: saveBGtoFile\nUI: Cursor Set >> Idle\nData: showBG\nRun: BGIncrement"] -> w541
              frame "Data", Default {
                n262 = local read "Video Display"() -> (w553:bool)
                n263 = Select(t="TCP: startCam", s=w553, f="") -> (s? t:f=w549:string)
                n264 = call <vilib>:"Add State(s) to Queue__JKI_lib_State_Machine.vi"("State(s) in Front (\"\")"="UI: Cursor Set >> Busy\nData: parseRunData\nData: saveRunData\nUI: Cursor Set>>Idle" ("State(s) in Front (\"\")"), "State(s) in (\"\")"=w549) -> ("States Out"=w551:string)  [unwired: 13 in]
              }
              frame "Cali" {
              }
              frame "BG" {
              }
            }
            n265 = Bundle By Name(cluster=w543, "SysRunning?"=FALSE) -> (w544:T25)
            n266 = Select(t="" ("State(s) in Front (\"\")"), s="Skip Data Save?", f=w541) -> (s? t:f=w538:string)
            n267 = call <vilib>:"Add State(s) to Queue__JKI_lib_State_Machine.vi"("State(s) in Front (\"\")"="TCP: stopRun\nUI: Update\nLabJack: AB_Stop\nLabJack: 355_PWM_Stop\nDigitizer: Abort\nLabJack: ZeroV\nUtility: EndBeep\nLED: BreathOff" ("State(s) in Front (\"\")"), "State(s) in (\"\")"=w538, "State(s) at Back (\"\")"="Macro: SysReadyForAq\nUI: Update" ("State(s) in Front (\"\")")) -> ("States Out"=w536:string)  [unwired: 12 in]
            n268 = call <vilib>:"Add State(s) to Queue__JKI_lib_State_Machine.vi"("State(s) in Front (\"\")"=w536, "State(s) in (\"\")"=w545) -> ("States Out"=w546:string)  [unwired: 13 in]
          }
          event Panel Close? {
            # "Discard the event because we'll close the front panel ourselves in Macro: Exit"
            # "Close Panel button (pressed) Event\n(this executes Macro: Exit to terminate the VI)"
            n269 = event-data() -> ()  [unwired: 1 in, 1 out]
            n270 = event-data ("Event Filter Node")("Discard?"=TRUE) -> ()  [unwired: 1 in, 1 out]
            n271 = call <vilib>:"Add State(s) to Queue__JKI_lib_State_Machine.vi"("State(s) in Front (\"\")"="Macro: Exit", "State(s) in (\"\")"=w561) -> ("States Out"=w560:string)  [unwired: 13 in]
          }
        }
      }
      frame "---------- Macro ----------" {
        # "Do not put any code in this frame.\n(It is a separator no-op. You can make a copy of this frame to create a new Macro frame)"
        n272 = call <vilib>:"Add State(s) to Queue__JKI_lib_State_Machine.vi"("State(s) in (\"\")"=w566) -> ("States Out"=w565:string)  [unwired: 14 in]
      }
      frame "Macro: Initialize" {
        # "load Labjack setting 1st as it contaisn laser pin infortmation"
        # "start laser 1st, need 7.5s for laser to get ready"
        # "Initialization Macro\n(This is called once, when the VI starts)"
        n273 = call <vilib>:"Add State(s) to Queue__JKI_lib_State_Machine.vi"("State(s) in Front (\"\")"="UI: showDisclaimer\nUI: Cursor Set >> Busy\nData: Initialize\nInitialize Core Data\nUI: Initialize\nUI: Front Panel State >> Open\nMacro: LoadSysConfig\nTCP: InitializeNew\nTCP: checkSource\nUI: Update\nLabJack: Open\nLabJack: SetDefaultSub\nLED: OpenVIRef\nLED: BreathOrange\nUI: Update\n355 Laser: CheckControllerStatus\n355 Laser: Laser enable\n355 Laser: Dewelling>>500\n355 Laser: CheckControllerStatus\nUI: Update\nLabJack: 355_PWM_Config\nLabJack: AB_PWM_Config\nUI: Update", "State(s) in (\"\")"="Digitizer: Initialize\nDigitizer: Config\nUI: Update\nAimingBeam: Initialize\nAimingBeam: Set Status>>Enable\nAimingBeam: Set Current\nUI: Update\n355 Laser: Check Dewelling\nUI: Cursor Set >> Idle\nCase: GetID\nUI: Update\nTCP: SendSettingMacro\nCase: CreatFileStruct\nUI: Update\nData: loadLastUseMacro\nDeconEngine: InitilizeMacro\nGraph: SetXMultiplier\nGraph: AddCursors\nAPD: Initialize\nAPD: LoadFromSerial\nAPD: UpdateCtrlVLimit\nAPD: GetGainLimits\nPID: loadPID\nLED: BreathOff\nMacro: SysReadyForAq") -> ("States Out"=w567:string)  [unwired: 13 in]
        n274 = call <vilib>:"Add State(s) to Queue__JKI_lib_State_Machine.vi"("State(s) in Front (\"\")"=w567, "State(s) in (\"\")"=w575) -> ("States Out"=w574:string)  [unwired: 13 in]
        "Help" <- "Hover over controls to see help!" ("Help")
      }
      frame "Macro: LoadSysConfig" {
        # "System configuration Macro. [Covers: REQ15]\n(Load configurations for different component of the system)"
        n275 = call <vilib>:"Add State(s) to Queue__JKI_lib_State_Machine.vi"("State(s) in Front (\"\")"="SysConfig: Load Sys Config\nSysConfig: Load Digitizer Setting\nSysConfig: Load AB setting\nSysConfig: Load LJ Pinout\nSysConfig: Load 355 PWM\nSysConfig: LoadAPDSerialNumber\nSysConfig: LoadABVideoSetting\nSysConfig: LoadCursorLocation", "State(s) in (\"\")"=w581) -> ("States Out"=w580:string)  [unwired: 13 in]
      }
      frame "Macro: SysReadyForAq" {
        # "Macro for system ready\n(It is a separator no-op. You can make a copy of this frame to create a new Macro frame)"
        n276 = call <vilib>:"Add State(s) to Queue__JKI_lib_State_Machine.vi"("State(s) in Front (\"\")"="UI: ReadyForAquisition\nLED: Green" ("State(s) in Front (\"\")"), "State(s) in (\"\")"=w587) -> ("States Out"=w586:string)  [unwired: 13 in]
      }
      frame "Macro: Exit" {
        # "close LJ last"
        # "check whether hardware is initilized, if so close, if not do nothing"
        # "Exit Macro, close all hardware\n(This is called once, when the VI exits)"
        n277 = Unbundle By Name(w606) -> ("System Status.Digitizer"=w602:bool, "System Status.Aiming Beam"=w601:bool, "System Status.355 Laser"=w600:bool, "System Status.Labjack"=w591:bool, "Core.Close Panel on Exit?"=w595:bool)
        n278 = case shown="True" w602 {
          tunnel: ["" ("Empty String Constant") "Digitizer: Close"] -> w597
          frame False {
          }
          frame True {
          }
        }
        n279 = case shown="True" w591 {
          tunnel: ["" ("Empty String Constant") "LabJack: SetDefaultAndClose"] -> w588
          frame False {
          }
          frame True {
          }
        }
        n280 = case shown="True" w601 {
          tunnel: ["" ("Empty String Constant") "AimingBeam: Set Status >> Disable\nAimingBeam: Close"] -> w590
          frame False {
          }
          frame True {
          }
        }
        n281 = case shown="True" w600 {
          tunnel: ["" ("Empty String Constant") "355 Laser: Close\n355 Laser: CheckControllerStatus"] -> w589
          frame False {
          }
          frame True {
          }
        }
        n282 = Select(t="UI: Front Panel State >> Close", s=w595, f="" ("Empty String Constant")) -> (s? t:f=w592:string)
        n283 = call <vilib>:"Add State(s) to Queue__JKI_lib_State_Machine.vi"("State(s) in Front (\"\")"="TCP: Close", "State(s) in (\"\")"=w597, "State(s) at Back (\"\")"=w590) -> ("States Out"=w599:string)  [unwired: 12 in]
        n284 = call <vilib>:"Add State(s) to Queue__JKI_lib_State_Machine.vi"("State(s) in Front (\"\")"=w599, "State(s) in (\"\")"=w589, "State(s) at Back (\"\")"=w588) -> ("States Out"=w594:string)  [unwired: 12 in]
        n285 = call <vilib>:"Add State(s) to Queue__JKI_lib_State_Machine.vi"("State(s) in Front (\"\")"=w594, "State(s) in (\"\")"="UI: Update\nUI: Reset\nGraph: SaveCursorLoc\nLED: CloseVIRef\nQueue: Destory\nData: Cleanup\nExit", "State(s) at Back (\"\")"=w592) -> ("States Out"=w603:string)  [unwired: 12 in]
        n286 = call <vilib>:"Add State(s) to Queue__JKI_lib_State_Machine.vi"("State(s) in Front (\"\")"=w603, "State(s) in (\"\")"=w609) -> ("States Out"=w608:string)  [unwired: 13 in]
      }
      frame "---------- Data ----------" {
        # "Do not put any code in this frame.\n(It is a separator no-op. You can make a copy of this frame to create a new Data frame)"
        n287 = call <vilib>:"Add State(s) to Queue__JKI_lib_State_Machine.vi"("State(s) in (\"\")"=w622) -> ("States Out"=w621:string)  [unwired: 14 in]
      }
      frame "Data: Initialize" {
        w623 = FALSE  # bothVidSourceAvail
        w624 = T1 {"Main Frame Grabber"=FALSE, "Side Frame Grabber"=FALSE, "Main Camera"=FALSE, "Side Camera"=FALSE}  # video source
        w625 = FALSE  # LED vi ref open?
        w627 = path ""  # CaliPath
        w628 = T24 {"DeCon Channel"=enum."1", "Scale Bar"=FALSE, "Scale Low"=3.0, "Scale High"=8.0, "ANSI"=20.0, "Radius"=1.0, "3D?"=FALSE, "Firefly?"=FALSE, "Pentero?"=FALSE}  # VideoConfig
        w629 = T28 {"Ch1APDSerial#"="", "Ch2APDSerial#"="", "Ch3APDSerial#"=""}  # APDSerialNum
        w630 = u32 0  # Aquisition Timer
        w631 = cluster{"RunID":i8, "BG ID":i8, "Cali ID":i8} {"RunID"=1, "BG ID"=1, "Cali ID"=1}  # IDs
        w632 = refnum<vi> refnum  # LED vi reference
        w633 = path ""  # TempPath
        w634 = T29 {"DataPath"=path "", "BG Path"=path "", "iRFPath"=path "", "CaliPath"=path ""}  # Pathes
        w636 = dbl[] []  # V3
        w637 = dbl[] []  # V2
        w638 = dbl[] []  # V1
        w640 = u32 0  # FastTimer
        w641 = u32 0  # SlowTimer
        w642 = dbl[][] []  # Ch3Data
        w643 = dbl[][] []  # Ch2Data
        w626 = dbl[][] []  # Ch1Data
        w646 = T2 {"Digitizer"=FALSE, "Labjack"=FALSE, "Aiming Beam"=FALSE, "355 Laser"=FALSE, "TCP/IP"=FALSE}  # System Status
        w647 = T30 {"DIO_EF_CLOCK1_DIVISOR"=16, "DIO_EF_CLOCK1_ROLL_VALUE"=25000, "DIO#_EF_INDEX"=0, "DIO#_EF_OPTIONS"=1, "DIO#_EF_CONFIG_A"=6250}  # AB PWM setting
        w648 = T5 {"Ch1 Bias"="TDA11", "Ch2 Bias"="DAC10", "Ch3 Bias"="DAC0", "Ch4 Bias"="DAC0", "355 PWM"="FIO0", "AimingBeam PWM"="FIO2", "Laser Ready"="FIO3", "Interlock"="FIO1", "Laser Start/Stop"="FIO1", "Red LED"="FIO1", "Green LED"="FIO1", "Foot Pedal"="DIO15"}  # LJ Pinout
        w649 = 0  # TCP attempt count
        w650 = u32 0  # Laser start tic
        w651 = refnum<k20>[] []  # niTClk sessions
        w652 = u32 0  # Last Trigger
        w653 = T30 {"DIO_EF_CLOCK1_DIVISOR"=16, "DIO_EF_CLOCK1_ROLL_VALUE"=25000, "DIO#_EF_INDEX"=0, "DIO#_EF_OPTIONS"=1, "DIO#_EF_CONFIG_A"=6250}  # 355 PWM setting
        w654 = T31 {"Aiming Beam COM Port"="COM3", "Min Current"=0.0, "Max Current"=63.0, "Default Current"=20.0, "Freq"=0}  # AB Cluster
        w655 = T32 {"resource name"="", "resource name 2"="", "Channel"=enum."Channel 0", "trigger source"="VAL_EXTERNAL", "trigger level"=0.5, "trigger delay"=1.35e-07, "min sample rate"=12500000000.0, "min record length"=2500, "vertical range"=1.0, "vertical offset"=-0.25, "Waveform to Avg"=2000}  # FLImDAQ
        w656 = FALSE  # SysRunning?
        w644 = path ""  # DefaultPath
        w657 = ""  # CaseID
        w658 = T4 {"Ch1Enable?"=FALSE, "Ch2Enable?"=FALSE, "Ch3Enable?"=FALSE, "Ch1AutoGain?"=FALSE, "Ch2AutoGain?"=FALSE, "Ch3AutoGain?"=FALSE, "AimingBeamEnable?"=FALSE}  # SysConfigCluster
        w659 = T33 {"Current VI Reference"=refnum, "Close Panel on Exit?"=FALSE}  # Core
        # "Initialize the shift-register data, here.\n(data names are defined by what you wire into the bundle function)"
        n288 = Bundle("Core"=w659, "SysConfigCluster"=w658, "System Status"=w646, "IDs"=w631, "CaseID"=w657, "DefaultPath"=w644, "Pathes"=w634, "FLImDAQ"=w655, "SysRunning?"=w656, "AB Cluster"=w654, "LJ Pinout"=w648, "355 PWM setting"=w653, "AB PWM setting"=w647, "Last Trigger"=w652, "niTClk sessions"=w651, "Laser start tic"=w650, "TCP attempt count"=w649, "Ch1Data"=w626, "Ch2Data"=w643, "Ch3Data"=w642, "V1"=w638, "V2"=w637, "V3"=w636, "SlowTimer"=w641, "FastTimer"=w640, "listener ID"=refnum<k5> refnum, "TempPath"=w633, "LED vi reference"=w632, "Aquisition Timer"=w630, "APDSerialNum"=w629, "VideoConfig"=w628, "CaliPath"=w627, "LED vi ref open?"=w625, "video source"=w624, "bothVidSourceAvail"=w623) -> (w635:T25)  [unwired: 1 in]
        n289 = call <vilib>:"Add State(s) to Queue__JKI_lib_State_Machine.vi"("State(s) in (\"\")"=w662) -> ("States Out"=w661:string)  [unwired: 14 in]
      }
      frame "Data: LoadAPDData" {
        # "only load the last iRF for the moment"
        # "Load APD detector data\n(It is a separator no-op. You can make a copy of this frame to create a new Data frame)"
        n290 = Unbundle By Name(w693) -> ("APDSerialNum.Ch1APDSerial#"=w692:string, "APDSerialNum.Ch2APDSerial#"=w664:string, "APDSerialNum.Ch3APDSerial#"=w663:string)
        n291 = call "CreatFromSerialNumNoRaw.vi"("error in (no error)"=w691, "APD Serial #"=w692) -> ("error out"=w689:errorcluster, "APDClass out"=w690:refnum<class "APDClass.lvclass">)  [unwired: 8 in]
        n292 = call "CreatFromSerialNumNoRaw.vi"("error in (no error)"=w691, "APD Serial #"=w664) -> ("error out"=w678:errorcluster, "APDClass out"=w679:refnum<class "APDClass.lvclass">)  [unwired: 8 in]
        n293 = call "CreatFromSerialNumNoRaw.vi"("error in (no error)"=w691, "APD Serial #"=w663) -> ("error out"=w671:errorcluster, "APDClass out"=w672:refnum<class "APDClass.lvclass">)  [unwired: 8 in]
        n294 = call-dynamic "Read iRFData.vi"("error in (no error)"=w689, "APDClass in"=w690) -> ("iRFData"=w688:T34)  [unwired: 7 in, 2 out]
        n295 = call-dynamic "Read iRFData.vi"("error in (no error)"=w678, "APDClass in"=w679) -> ("iRFData"=w683:T34)  [unwired: 7 in, 2 out]
        n296 = call-dynamic "Read iRFData.vi"("error in (no error)"=w671, "APDClass in"=w672) -> ("iRFData"=w676:T34)  [unwired: 7 in, 2 out]
        n297 = Unbundle By Name(w688) -> ("iRFWFsAvg"=w687:dbl[][])
        n298 = Unbundle By Name(w683) -> ("iRFWFsAvg"=w682:dbl[][])
        n299 = Unbundle By Name(w676) -> ("iRFWFsAvg"=w675:dbl[][])
        n300 = Array Size(array=w687) -> (size(s)=w686:i32[])
        n301 = Array Size(array=w682) -> (size(s)=w677:i32[])
        n302 = Array Size(array=w675) -> (size(s)=w670:i32[])
        n303 = Index Array(array=w686, index=1) -> (element=w684:i32)
        n304 = Index Array(array=w677, index=1) -> (element=w680:i32)
        n305 = Index Array(array=w670, index=1) -> (element=w673:i32)
        n306 = Index Array(array=w687, index (row)=w684) -> (element=w669:dbl[])  [unwired: 1 in]
        n307 = Index Array(array=w682, index (row)=w680) -> (element=w668:dbl[])  [unwired: 1 in]
        n308 = Index Array(array=w675, index (row)=w673) -> (element=w667:dbl[])  [unwired: 1 in]
        n309 = Bundle("iRFWFsAvg"=w669, "iRFWFsAvg"=w668, "iRFWFsAvg"=w667) -> (w666:T35)  [unwired: 1 in]
        n310 = global write "GlobalVariables.vi" "LastUseiRF"(w666) -> ()
        n311 = call <vilib>:"Add State(s) to Queue__JKI_lib_State_Machine.vi"("State(s) in Front (\"\")"="UI: CaliAndiRFLoaded" ("State(s) in Front (\"\")"), "State(s) in (\"\")"=w696) -> ("States Out"=w695:string)  [unwired: 13 in]
      }
      frame "Data: loadLastUseiRF" {
        # "Load last use iRF.\n()"
        n312 = Unbundle By Name(w701) -> ("TempPath"=w700:path)
        n313 = Build Path(base path=w700, name or relative path="iRF.tdms") -> (appended path=w706:path)
        n314 = TDMS Open(11:w706) -> (0:w704:errorcluster, 3:w705:refnum<k34>)  [unwired: 6 in]
        n315 = TDMS Read(0:w705, 11:w704, 12:dbl[][] []) -> (4:w698:refnum<k34>, 10:w702:dbl[][], 15:w697:errorcluster)  [unwired: 5 in, 3 out]
        n316 = TDMS Close(8:w697, 11:w698) -> ()  [unwired: 2 out]
        n317 = case shown="No Error" w697 {
          tunnel: w702 -> [w724 _]
          tunnel: ["UI: CaliAndiRFLoaded" ("State(s) in Front (\"\")") "" ("Empty String Constant")] -> w699
          frame No Error {
            n318 = Index Array(array=w724, index (row)=0) -> (element=w720:dbl[])  [unwired: 1 in]
            n319 = Index Array(array=w724, index (row)=1) -> (element=w717:dbl[])  [unwired: 1 in]
            n320 = Index Array(array=w724, index (row)=2) -> (element=w714:dbl[])  [unwired: 1 in]
            n321 = Add Array Elements(numeric array=w720) -> (sum=w719:dbl)
            n322 = Add Array Elements(numeric array=w717) -> (sum=w716:dbl)
            n323 = Add Array Elements(numeric array=w714) -> (sum=w713:dbl)
            n324 = Divide(x=w720, y=w719) -> (x/y=w718:dbl[])
            n325 = Divide(x=w717, y=w716) -> (x/y=w715:dbl[])
            n326 = Divide(x=w714, y=w713) -> (x/y=w712:dbl[])
            n327 = Bundle(w718, w715, w712) -> (w723:cluster{dbl[], dbl[], dbl[]})  [unwired: 1 in]
            n328 = global write "GlobalVariables.vi" "LastUseiRF"(w723) -> ()
            n329 = Array Size(array=w720) -> (size(s)=→"iRF length":i32)
          }
          frame Error {
          }
        }
        n330 = call <vilib>:"Add State(s) to Queue__JKI_lib_State_Machine.vi"("State(s) in Front (\"\")"=w699, "State(s) in (\"\")"=w711) -> ("States Out"=w710:string)  [unwired: 13 in]
      }
      frame "Data: loadSystemCali" {
        # "Load last use calibration.\n()"
        n331 = Unbundle By Name(w736) -> ("CaliPath"=w735:path)
        n332 = Build Path(base path=w735, name or relative path="Calibration.tdms") -> (appended path=w731:path)
        n333 = call "ReadBGorCali (SubVI).vi"("DataType"=enum16{"BG", "Cali"}."Cali", "error in (no error)"=w730, "file path in"=w731) -> ("error out"=w732:errorcluster, "CtrlVCluster"=w734:T36, "AvgDataCluster"=w733:T37)  [unwired: 6 in]
        n334 = case shown="No Error" w732 {
          tunnel: w734 -> [w751 _]
          tunnel: w733 -> [w750 _]
          frame No Error {
            n335 = Unbundle By Name(w751) -> ("V 1"=w746:dbl[], "V 2"=w745:dbl[], "V 3"=w744:dbl[])
            n336 = Unbundle By Name(w750) -> ("Channel 1"=w749:dbl[], "Channel 2"=w748:dbl[], "Channel 3"=w747:dbl[])
            n337 = Index Array(array=w744) -> (element=w741:dbl)  [unwired: 1 in]
            n338 = Index Array(array=w746) -> (element=w743:dbl)  [unwired: 1 in]
            n339 = Index Array(array=w745) -> (element=w742:dbl)  [unwired: 1 in]
            n340 = Bundle By Name(cluster=T18 {"Ch1 WF"=array[400 elements], "Ch2 WF"=array[400 elements], "Ch3 WF"=array[400 elements], "V1"=0.0, "V2"=0.0, "V3"=0.0} ("LastUseCaliData"), "Ch1 WF"=w749, "Ch2 WF"=w748, "Ch3 WF"=w747, "V1"=w743, "V2"=w742, "V3"=w741) -> (w752:T18)
            n341 = global write "GlobalVariables.vi" "SysCaliData"(w752) -> ()
          }
          frame Error {
          }
        }
        n342 = call <vilib>:"Add State(s) to Queue__JKI_lib_State_Machine.vi"("State(s) in (\"\")"=w740) -> ("States Out"=w739:string)  [unwired: 14 in]
      }
      frame "Data: loadLastUseBG" {
        w760 = enum16{"write", "read"}."write" ("action")
        # "Load last use BG.\n()"
        n343 = Unbundle By Name(w774) -> ("TempPath"=w773:path)
        n344 = Build Path(base path=w773, name or relative path="Background.tdms") -> (appended path=w772:path)
        n345 = call "ReadBGorCali (SubVI).vi"("DataType"=enum16{"BG", "Cali"}."BG", "error in (no error)"=w771, "file path in"=w772) -> ("error out"=w770:errorcluster, "AvgDataCluster"=w765:T37)  [unwired: 6 in, 1 out]
        n346 = Unbundle By Name(w765) -> ("Channel 1"=w756:dbl[], "Channel 2"=w764:dbl[], "Channel 3"=w755:dbl[])
        n347 = call "FLImDAQ_FGV.vi"() -> ("Read data"=w769:T6)  [unwired: 10 in, 1 out]
        n348 = Unbundle By Name(w769) -> ("min record length"=w761:i32)
        n349 = Array Size(array=w755) -> (size(s)=w763:i32)
        "BG length" <- w763
        n350 = Equal?(x=w763, y=w761) -> (x = y?=w762:bool)
        n351 = Select(t="UI: BGLoaded" ("State(s) in Front (\"\")"), s=w762, f="UI: BGSizeError" ("State(s) in Front (\"\")")) -> (s? t:f=w766:string)
        n352 = case shown="True" w762 {
          tunnel: w756 -> [_ w784]
          tunnel: w764 -> [_ w783]
          tunnel: w755 -> [_ w782]
          tunnel: w761 -> [w780 _]
          tunnel: [w779 w784] -> w759
          tunnel: [w779 w783] -> w758
          tunnel: [w779 w782] -> w757
          frame False {
            # "If error set BG all 0, update UI"
            n353 = for {
              N: w780 -> [_]
              tunnel: [0.0] -> w779 mode=indexing
            }
          }
          frame True {
            # "If no error, check size match"
          }
        }
        n354 = call "BG3FGV.vi"("action"=w760, "BG3 in"=w757) -> ()  [unwired: 8 in, 2 out]
        n355 = call "BG1FGV.vi"("action"=w760, "BG1 in"=w759) -> ()  [unwired: 8 in, 2 out]
        n356 = call "BG2FGV.vi"("action"=w760, "BG2 in"=w758) -> ()  [unwired: 8 in, 2 out]
        n357 = call <vilib>:"Add State(s) to Queue__JKI_lib_State_Machine.vi"("State(s) in Front (\"\")"=w766, "State(s) in (\"\")"=w778) -> ("States Out"=w777:string)  [unwired: 13 in]
      }
      frame "Data: loadLastUseMacro" {
        # "Load last use BG and Cali and iRF.\n(It is a separator no-op. You can make a copy of this frame to create a new Data frame)"
        n358 = call <vilib>:"Add State(s) to Queue__JKI_lib_State_Machine.vi"("State(s) in Front (\"\")"="Data: loadLastUseBG\nData: loadSystemCali\nData: loadLastUseiRF\n/*Data: LoadAPDData" ("State(s) in Front (\"\")"), "State(s) in (\"\")"=w790) -> ("States Out"=w789:string)  [unwired: 13 in]
      }
      frame "Data: saveCalibration" {
        # "Average data and save calibration file. [Covers: REQ11]\n(It is a separator no-op. You can make a copy of this frame to create a new Data frame)"
        n359 = Unbundle By Name(w806) -> ("Ch1Data"=w805:dbl[][], "V1"=w804:dbl[], "Ch2Data"=w803:dbl[][], "V2"=w802:dbl[], "Ch3Data"=w801:dbl[][], "V3"=w800:dbl[], "Pathes.CaliPath"=w809:path, "IDs.Cali ID"=w808:i8)
        n360 = Increment(x=w808) -> (x+1=w791:i8)
        n361 = Bundle("Ch1Data"=w805, "V1"=w804) -> (w799:cluster{"Ch1Data":dbl[][], "V1":dbl[]})  [unwired: 1 in]
        n362 = Bundle("Ch2Data"=w803, "V2"=w802) -> (w798:cluster{"Ch2Data":dbl[][], "V2":dbl[]})  [unwired: 1 in]
        n363 = Bundle("Ch3Data"=w801, "V3"=w800) -> (w797:cluster{"Ch3Data":dbl[][], "V3":dbl[]})  [unwired: 1 in]
        n364 = Format Value(string ("")="Calibration" ("default name"), format string="%02d", value (0)=w791) -> (output string=w811:string)
        n365 = Build Path(base path=w809, name or relative path=w811) -> (appended path=w796:path)
        n366 = call "SaveBGorCali (SubVI).vi"("DataType"=enum16{"BG", "Cali"}."Cali", "SytemID"="UCDMC", "BG path"=w796, "error in (no error)"=w795, "Channel 3"=w797, "Channel 2"=w798, "Channel1"=w799) -> ("error out"=w794:errorcluster)  [unwired: 4 in]
        n367 = call <vilib>:"Add State(s) to Queue__JKI_lib_State_Machine.vi"("State(s) in (\"\")"=w814) -> ("States Out"=w813:string)  [unwired: 14 in]
      }
      frame "Data: saveiRF" {
        w839 = enum16{"write", "read"}."read" ("action")
        # "Get iRF from decon stracture and save it on disk.\n(It is a separator no-op. You can make a copy of this frame to create a new Data frame)"
        n368 = Unbundle By Name(w832) -> ("TempPath"=w831:path)
        n369 = call "Ch1DeconEngineFGV.vi"("action(read)"=w839) -> ("Error Out"=w837:errorcluster, "Ch1DeconEngine out"=w838:refnum<class "LaguerreDeconEngineClass.lvclass">)  [unwired: 9 in]
        n370 = call "Ch2DeconEngineFGV.vi"("action(read)"=w839) -> ("Error Out"=w835:errorcluster, "Ch2DeconEngine out"=w836:refnum<class "LaguerreDeconEngineClass.lvclass">)  [unwired: 9 in]
        n371 = call "Ch3DeconEngineFGV.vi"("action(read)"=w839) -> ("Error Out"=w833:errorcluster, "Ch3DeconEngine out"=w834:refnum<class "LaguerreDeconEngineClass.lvclass">)  [unwired: 9 in]
        n372 = Build Path(base path=w831, name or relative path="iRF" ("default name")) -> (appended path=w829:path)
        n373 = call "getIRF.vi"("error in (no error)"=w837, "LaguerreDeconEngineClass in"=w838) -> ("iRF"=w818:dbl[])  [unwired: 7 in, 2 out]
        n374 = call "getIRF.vi"("error in (no error)"=w835, "LaguerreDeconEngineClass in"=w836) -> ("iRF"=w817:dbl[])  [unwired: 7 in, 2 out]
        n375 = call "getIRF.vi"("error in (no error)"=w833, "LaguerreDeconEngineClass in"=w834) -> ("iRF"=w816:dbl[])  [unwired: 7 in, 2 out]
        n376 = Build Array(w818, w817, w816) -> (w824:dbl[][])
        n377 = TDMS Open(8:w828, 10:T19."create or replace" ("operation (0:open)"), 11:w829) -> (0:w825:errorcluster, 3:w826:refnum<k34>)  [unwired: 4 in]
        n378 = Bundle("iRF"=w818, "iRF"=w817, "iRF"=w816) -> (w815:cluster{"iRF":dbl[], "iRF":dbl[], "iRF":dbl[]})  [unwired: 1 in]
        n379 = global write "GlobalVariables.vi" "LastUseiRF"(w815) -> ()
        n380 = TDMS Write(0:w826, 5:"iRF" ("group name in (Untitled)"), 7:string[] ["Ch1", "Ch2", "Ch3"] ("channel name(s) in (Untitled)"), 9:w824, 11:w825) -> (4:w821:refnum<k34>, 15:w820:errorcluster)  [unwired: 1 in, 2 out]
        n381 = TDMS Close(8:w820, 11:w821) -> (0:w819:errorcluster)  [unwired: 1 out]
        n382 = call <vilib>:"Add State(s) to Queue__JKI_lib_State_Machine.vi"("State(s) in (\"\")"=w842) -> ("States Out"=w841:string)  [unwired: 14 in]
      }
      frame "Data: saveBGtoFGV" {
        w848 = enum16{"write", "read"}."write" ("action")
        # "Save BG and pass it to FGV.\n(save BG to disk and set it to FGV)"
        n383 = Unbundle By Name(w851) -> ("Ch1Data"=w850:dbl[][], "Ch2Data"=w849:dbl[][], "Ch3Data"=w847:dbl[][])
        n384 = call "AvgArrayTimeCritical.vi"("2D array"=w850) -> ("1D Avg"=w846:dbl[])  [unwired: 10 in]
        n385 = call "AvgArrayTimeCritical.vi"("2D array"=w849) -> ("1D Avg"=w845:dbl[])  [unwired: 10 in]
        n386 = call "AvgArrayTimeCritical.vi"("2D array"=w847) -> ("1D Avg"=w844:dbl[])  [unwired: 10 in]
        n387 = call "BG1FGV.vi"("action"=w848, "BG1 in"=w846) -> ()  [unwired: 8 in, 2 out]
        n388 = call "BG2FGV.vi"("action"=w848, "BG2 in"=w845) -> ()  [unwired: 8 in, 2 out]
        n389 = call "BG3FGV.vi"("action"=w848, "BG3 in"=w844) -> ()  [unwired: 8 in, 2 out]
        n390 = call <vilib>:"Add State(s) to Queue__JKI_lib_State_Machine.vi"("State(s) in (\"\")"=w854) -> ("States Out"=w853:string)  [unwired: 14 in]
      }
      frame "Data: saveBGtoFile" {
        w873 = "Background" ("name or relative path")
        # "Save BG to file.\n(save BG to disk both data folder and temp folder)"
        n391 = Unbundle By Name(w877) -> ("Pathes.BG Path"=w870:path, "IDs.BG ID"=w869:i8, "Ch1Data"=w867:dbl[][], "V1"=w866:dbl[], "Ch2Data"=w865:dbl[][], "V2"=w864:dbl[], "Ch3Data"=w863:dbl[][], "V3"=w862:dbl[], "TempPath"=w875:path)
        n392 = Increment(x=w869) -> (x+1=w874:i8)
        n393 = Format Value(string ("")=w873, format string="%02d", value (0)=w874) -> (output string=w872:string)
        n394 = Build Path(base path=w875, name or relative path=w873) -> (appended path=w856:path)
        n395 = call "File Dialog2"("start path"=w870, "prompt"="Please select BG name, DO NOT CANCEL!", "default name"=w872) -> ("selected path"=w857:path)  [unwired: 9 in, 3 out]
        n396 = Bundle("Ch1Data"=w867, "V1"=w866) -> (w861:cluster{"Ch1Data":dbl[][], "V1":dbl[]})  [unwired: 1 in]
        n397 = Bundle("Ch2Data"=w865, "V2"=w864) -> (w860:cluster{"Ch2Data":dbl[][], "V2":dbl[]})  [unwired: 1 in]
        n398 = Bundle("Ch3Data"=w863, "V3"=w862) -> (w859:cluster{"Ch3Data":dbl[][], "V3":dbl[]})  [unwired: 1 in]
        n399 = Build Array(w857, w856) -> (w855:path[])
        n400 = for {
          tunnel: w861 -> [w887]
          tunnel: w860 -> [w886]
          tunnel: w859 -> [w885]
          shift-right: [w888] -> w868
          shift-left: w858 -> [w884]
          tunnel: w855 -> [w883] mode=indexing
          n401 = call "SaveBGorCali (SubVI).vi"("DataType"=enum16{"BG", "Cali"}."BG", "SytemID"="UCDMC", "BG path"=w883, "error in (no error)"=w884, "Channel 3"=w885, "Channel 2"=w886, "Channel1"=w887) -> ("error out"=w888:errorcluster)  [unwired: 4 in]
        }
        n402 = call <vilib>:"Add State(s) to Queue__JKI_lib_State_Machine.vi"("State(s) in (\"\")"=w880) -> ("States Out"=w879:string)  [unwired: 14 in]
      }
      frame "Data: showBG" {
        # "Show BG in seperate window.\n()"
        n403 = call "showBG.vi"() -> ()  [unwired: 12 in]
        n404 = call <vilib>:"Add State(s) to Queue__JKI_lib_State_Machine.vi"("State(s) in (\"\")"=w893) -> ("States Out"=w892:string)  [unwired: 14 in]
      }
      frame "Data: irfAlignment" {
        w940 = enum16{"write", "read"}."write" ("action")
        # "do iRF alignment in this state\n(It is a separator no-op. You can make a copy of this frame to create a new Data frame)"
        n405 = Unbundle By Name(w918) -> ("Ch1Data"=w956:dbl[][], "Ch2Data"=w955:dbl[][], "Ch3Data"=w954:dbl[][])
        n406 = call "Ch1DeconEngineFGV.vi"("Error In"=w953) -> ("Error Out"=w951:errorcluster, "Ch1DeconEngine out"=w952:refnum<class "LaguerreDeconEngineClass.lvclass">)  [unwired: 9 in]
        n407 = call "Ch2DeconEngineFGV.vi"("Error In"=w953) -> ("Error Out"=w949:errorcluster, "Ch2DeconEngine out"=w950:refnum<class "LaguerreDeconEngineClass.lvclass">)  [unwired: 9 in]
        n408 = call "Ch3DeconEngineFGV.vi"("Error In"=w953) -> ("Error Out"=w947:errorcluster, "Ch3DeconEngine out"=w948:refnum<class "LaguerreDeconEngineClass.lvclass">)  [unwired: 9 in]
        n409 = call "AvgArray.vi"("2D array in"=w955) -> ("1D Avg out"=w899:dbl[])  [unwired: 10 in]
        n410 = call "AvgArray.vi"("2D array in"=w954) -> ("1D Avg out"=w898:dbl[])  [unwired: 10 in]
        n411 = call "AvgArray.vi"("2D array in"=w956) -> ("1D Avg out"=w900:dbl[])  [unwired: 10 in]
        n412 = call "RemoveDCBG.vi"("WF in"=w900) -> ("DC"=w907:dbl, "WF out"=w897:dbl[])  [unwired: 8 in, 1 out]
        n413 = call "RemoveDCBG.vi"("WF in"=w899) -> ("DC"=w904:dbl, "WF out"=w910:dbl[])  [unwired: 8 in, 1 out]
        n414 = call "RemoveDCBG.vi"("WF in"=w898) -> ("DC"=w902:dbl, "WF out"=w909:dbl[])  [unwired: 8 in, 1 out]
        n415 = call "computeIRFAlignment.vi"("error in (no error)"=w951, "fIRF temp"=w897, "LaguerreDeconEngineClass in"=w952) -> ("error out"=w943:errorcluster, "LaguerreDeconEngineClass out"=w944:refnum<class "LaguerreDeconEngineClass.lvclass">)  [unwired: 6 in, 1 out]
        n416 = call "computeIRFAlignment.vi"("error in (no error)"=w949, "fIRF temp"=w910, "LaguerreDeconEngineClass in"=w950) -> ("error out"=w941:errorcluster, "LaguerreDeconEngineClass out"=w942:refnum<class "LaguerreDeconEngineClass.lvclass">)  [unwired: 6 in, 1 out]
        n417 = call "computeIRFAlignment.vi"("error in (no error)"=w947, "fIRF temp"=w909, "LaguerreDeconEngineClass in"=w948) -> ("error out"=w945:errorcluster, "LaguerreDeconEngineClass out"=w946:refnum<class "LaguerreDeconEngineClass.lvclass">)  [unwired: 6 in, 1 out]
        n418 = call "Ch1DeconEngineFGV.vi"("Error In"=w943, "action(read)"=w940, "Ch1DeconEngine in"=w944) -> ("Error Out"=w938:errorcluster, "Ch1DeconEngine out"=w939:refnum<class "LaguerreDeconEngineClass.lvclass">)  [unwired: 7 in]
        n419 = call "Ch2DeconEngineFGV.vi"("Error In"=w941, "action(read)"=w940, "Ch2DeconEngine in"=w942) -> ("Error Out"=w928:errorcluster, "Ch2DeconEngine out"=w929:refnum<class "LaguerreDeconEngineClass.lvclass">)  [unwired: 7 in]
        n420 = call "Ch3DeconEngineFGV.vi"("Error In"=w945, "action(read)"=w940, "Ch3DeconEngine in"=w946) -> ("Error Out"=w922:errorcluster, "Ch3DeconEngine out"=w923:refnum<class "LaguerreDeconEngineClass.lvclass">)  [unwired: 7 in]
        n421 = call "setfIRF.vi"("error in (no error)"=w922, "fIRF"=w909, "LaguerreDeconEngineClass in"=w923) -> ("error out"=w926:errorcluster, "LaguerreDeconEngineClass out"=w927:refnum<class "LaguerreDeconEngineClass.lvclass">)  [unwired: 7 in]
        n422 = call "setfIRF.vi"("error in (no error)"=w928, "fIRF"=w910, "LaguerreDeconEngineClass in"=w929) -> ("error out"=w932:errorcluster, "LaguerreDeconEngineClass out"=w933:refnum<class "LaguerreDeconEngineClass.lvclass">)  [unwired: 7 in]
        n423 = call "setfIRF.vi"("error in (no error)"=w938, "fIRF"=w897, "LaguerreDeconEngineClass in"=w939) -> ("error out"=w936:errorcluster, "LaguerreDeconEngineClass out"=w937:refnum<class "LaguerreDeconEngineClass.lvclass">)  [unwired: 7 in]
        n424 = Unbundle By Name(w918) -> ("V1"=w895:dbl[], "V2"=w917:dbl[], "V3"=w916:dbl[])
        n425 = call "computeLCs.vi"("error in (no error)"=w936, "LaguerreDeconClass in"=w937) -> ("error out"=w934:errorcluster, "LaguerreDeconClass out"=w935:refnum<class "LaguerreDeconEngineClass.lvclass">)  [unwired: 8 in]
        n426 = call "computeLCs.vi"("error in (no error)"=w932, "LaguerreDeconClass in"=w933) -> ("error out"=w930:errorcluster, "LaguerreDeconClass out"=w931:refnum<class "LaguerreDeconEngineClass.lvclass">)  [unwired: 8 in]
        n427 = call "computeLCs.vi"("error in (no error)"=w926, "LaguerreDeconClass in"=w927) -> ("error out"=w924:errorcluster, "LaguerreDeconClass out"=w925:refnum<class "LaguerreDeconEngineClass.lvclass">)  [unwired: 8 in]
        n428 = call-poly <vilib>:"Mean.vi"("X"=w895) -> ("mean"=w894:dbl)  [unwired: 1 out]
        n429 = call "getFitting.vi"("error in (no error)"=w934, "LaguerreDeconEngineClass in"=w935) -> ("Fitting"=w906:dbl[])  [unwired: 7 in, 2 out]
        n430 = call "getFitting.vi"("error in (no error)"=w930, "LaguerreDeconEngineClass in"=w931) -> ("Fitting"=w903:dbl[])  [unwired: 7 in, 2 out]
        n431 = call "getFitting.vi"("error in (no error)"=w924, "LaguerreDeconEngineClass in"=w925) -> ("Fitting"=w896:dbl[])  [unwired: 7 in, 2 out]
        n432 = call-poly <vilib>:"Mean.vi"("X"=w917) -> ("mean"=w915:dbl)  [unwired: 1 out]
        n433 = Add(x=w907, y=w906) -> (x+y=w908:dbl[])
        n434 = Add(x=w904, y=w903) -> (x+y=w905:dbl[])
        n435 = call-poly <vilib>:"Mean.vi"("X"=w916) -> ("mean"=w914:dbl)  [unwired: 1 out]
        n436 = Add(x=w902, y=w896) -> (x+y=w901:dbl[])
        n437 = Build Array(w900, w908) -> (w921:dbl[][])
        n438 = Build Array(w899, w905) -> (w920:dbl[][])
        n439 = Build Array(w898, w901) -> (w919:dbl[][])
        n440 = Bundle("mean"=w894, "mean"=w915, "mean"=w914) -> (w913:cluster{"mean":dbl, "mean":dbl, "mean":dbl})  [unwired: 1 in]
        n441 = call "Calib_and_iRFAlign_confirm.vi"("Ch4 Data"=w913, "Ch3 Data"=w919, "Ch2 Data"=w920, "Ch1 Data"=w921) -> ("Save?"=w912:bool)  [unwired: 7 in]
        n442 = case shown="True" w912 {
          tunnel: ["" ("Empty String Constant") "Data: saveCalibration\nData: saveiRF\nRun: CaliIncrement"] -> w911
          frame False {
          }
          frame True {
            # "[Covers: REQ2]"
          }
        }
        n443 = call <vilib>:"Add State(s) to Queue__JKI_lib_State_Machine.vi"("State(s) in Front (\"\")"=w911, "State(s) in (\"\")"=w959) -> ("States Out"=w958:string)  [unwired: 13 in]
      }
      frame "Data: parseRunData" {
        # "All APD bias"
        # "flash queue"
        # "Ch3&4"
        # "Ch1&2"
        # "Flash data from queue and save it in structure\n()"
        n444 = Flush Queue(queue=w989, error in (no error)=w982) -> (remaining elements=w987:cluster{"double data":dbl[][]}[], error out=w980:errorcluster)  [unwired: 1 out]
        n445 = Flush Queue(queue=w983, error in (no error)=w982) -> (remaining elements=w977:cluster{"V1":dbl, "V2":dbl, "V3":dbl}[], error out=w978:errorcluster)  [unwired: 1 out]
        n446 = Flush Queue(queue=w988, error in (no error)=w982) -> (remaining elements=w986:cluster{"double data":dbl[][]}[], error out=w979:errorcluster)  [unwired: 1 out]
        n447 = for {
          tunnel: w986 -> [w999] mode=indexing
          tunnel: [w998] -> w972 mode=concatenating
          n448 = Unbundle By Name(w999) -> ("double data"=w997:dbl[][])
          n449 = call "SeperateChanData.vi"("Input (Ch1&2)"=w997) -> ("Ch1"=w998:dbl[][])  [unwired: 1 out]
        }
        n450 = call "FLImDAQ_FGV.vi"() -> ("Read data"=w969:T6)  [unwired: 10 in, 1 out]
        n451 = Unbundle By Name(w969) -> ("Waveform to Avg"=w962:i16)
        n452 = for {
          tunnel: w977 -> [w996] mode=indexing
          tunnel: [w995] -> w968 mode=indexing
          tunnel: [w994] -> w966 mode=indexing
          tunnel: [w993] -> w964 mode=indexing
          n453 = Unbundle By Name(w996) -> ("V1"=w995:dbl, "V2"=w994:dbl, "V3"=w993:dbl)
        }
        n454 = for {
          tunnel: w987 -> [w1003] mode=indexing
          tunnel: [w1001] -> w971 mode=concatenating
          tunnel: [w1000] -> w973 mode=concatenating
          n455 = Unbundle By Name(w1003) -> ("double data"=w1002:dbl[][])
          n456 = call "SeperateChanData.vi"("Input (Ch1&2)"=w1002) -> ("Ch1"=w1001:dbl[][], "Ch2"=w1000:dbl[][])
        }
        n457 = call "DuplicateV(SubVI).vi"("Averaging"=w962, "V in"=w968) -> ("V out"=w967:dbl[])  [unwired: 9 in]
        n458 = call "DuplicateV(SubVI).vi"("Averaging"=w962, "V in"=w966) -> ("V out"=w965:dbl[])  [unwired: 9 in]
        n459 = call "DuplicateV(SubVI).vi"("Averaging"=w962, "V in"=w964) -> ("V out"=w963:dbl[])  [unwired: 9 in]
        n460 = Array Size(array=w967) -> (size(s)=→"V1 Size":i32)
        n461 = Array Size(array=w965) -> (size(s)=→"V2 Size":i32)
        n462 = Array Size(array=w963) -> (size(s)=→"V3 Size":i32)
        n463 = Bundle By Name(cluster=w984, "Ch1Data"=w971, "Ch2Data"=w973, "Ch3Data"=w972, "V1"=w967, "V2"=w965, "V3"=w963) -> (w985:T25)
        n464 = Array Size(array=w972) -> (size(s)=→"data Size":i32[])
        n465 = Merge Errors(w980, w979, w978) -> (w981:errorcluster)
        n466 = call <vilib>:"Add State(s) to Queue__JKI_lib_State_Machine.vi"("State(s) in (\"\")"=w992) -> ("States Out"=w991:string)  [unwired: 14 in]
      }
      frame "Data: saveRunData" {
        w1010 = T38 {"DataPath"=path "", "CaseID"="", "RunID"=0, "Ch1Data"=[], "Ch2Data"=[], "Ch3Data"=[], "V1"=[], "V2"=[], "V3"=[], "LaserRepRate"=0, "WFAverage"=0, "RunStartTime"=0}  # Data cluster
        # "Save FLIm data to disk.\n(Save to LV tdms file format)"
        n467 = Unbundle By Name(w1014) -> ("Pathes.DataPath"=w1009:path, "CaseID"=w1023:string, "IDs.RunID"=w1012:i8, "Ch1Data"=w1022:dbl[][], "Ch2Data"=w1021:dbl[][], "Ch3Data"=w1008:dbl[][], "V1"=w1020:dbl[], "V2"=w1019:dbl[], "V3"=w1018:dbl[])
        n468 = call "FLImDAQ_FGV.vi"() -> ("Read data"=w1006:T6)  [unwired: 10 in, 1 out]
        n469 = Unbundle By Name(w1006) -> ("Waveform to Avg"=w1005:i16)
        n470 = local read "Laser Rep Rate"() -> (w1007:dbl)
        n471 = Increment(x=w1012) -> (x+1=w1011:i8)
        n472 = local read "RunStartTime"() -> (w1004:u32)
        n473 = Bundle By Name(cluster=w1010, "DataPath"=w1009, "CaseID"=w1023, "RunID"=w1011, "Ch1Data"=w1022, "Ch2Data"=w1021, "Ch3Data"=w1008, "V1"=w1020, "V2"=w1019, "V3"=w1018, "LaserRepRate"=w1007, "WFAverage"=w1005, "RunStartTime"=w1004) -> (w1017:T38)
        n474 = call "SaveRunData(SubVI).vi"("Data cluster"=w1017, "error in (no error)"=w1016) -> ("error out"=w1013:errorcluster)  [unwired: 13 in]
        n475 = flat-sequence {
          tunnel: w1014 -> [w1031]
          tunnel: [w1028] -> w1015
          tunnel: w1013 -> [_]
          frame #0 {
            w1029 = dbl[][] [] ("Ch1Data")
            w1030 = dbl[] [] ("V1")
            n476 = Bundle By Name(cluster=w1031, "Ch1Data"=w1029, "Ch2Data"=w1029, "Ch3Data"=w1029, "V1"=w1030, "V2"=w1030, "V3"=w1030) -> (w1028:T25)
          }
        }
        n477 = case shown="No Error" w1013 {
          tunnel: ["Run: Increment" "" ("Empty String Constant")] -> w1024
          frame No Error {
          }
          frame Error {
          }
        }
        n478 = call <vilib>:"Add State(s) to Queue__JKI_lib_State_Machine.vi"("State(s) in Front (\"\")"=w1024, "State(s) in (\"\")"=w1027) -> ("States Out"=w1026:string)  [unwired: 13 in]
      }
      frame "Data: Cleanup" {
        # "Cleanup any data and references, here.\n(this is called automatically, by the Macro: Exit)"
        n479 = Unbundle By Name(w1035) -> ("Core.Current VI Reference"=w1038:refnum<vi>)
        n480 = Close Reference(reference=w1038, error in (no error)=w1037) -> (error out=w1036:errorcluster)
        n481 = call <vilib>:"Add State(s) to Queue__JKI_lib_State_Machine.vi"("State(s) in (\"\")"=w1040) -> ("States Out"=w1039:string)  [unwired: 14 in]
      }
      frame "---------- Core ----------" {
        # "Do not put any code in this frame.\n(it is a separator no-op)"
        n482 = call <vilib>:"Add State(s) to Queue__JKI_lib_State_Machine.vi"("State(s) in (\"\")"=w1045) -> ("States Out"=w1044:string)  [unwired: 14 in]
      }
      frame Default {
        w1056 = 42 items=["No error", "Argument error", "Memory is full", "Out of zone", "End of file", "File already open", "Generic file I/O error", "File not found", "File permission error", "Disk is full", "Duplicate path", "Too many files open", "System feature not enabled", "Resource file not found", "Cannot add resource", "Resource not found", "Image not found", "Image memory error", "Pen does not exist", "Config type invalid", "Config token not found", "Config parse error", "Config memory error", "Bad external code format", "Bad external code offset", "External code not present", "Null window", "Destroy window error", "Null menu", "Print aborted", "Bad print record", "Print driver error", "Windows error during printing", "Memory error during printing", "Print dialog error", "Generic print error", "Invalid device refnum", "Device not found", "Device parameter error", "Device unit error", "Cannot open device", "Device call aborted", "Generic error", "Cancelled by user", "Object ID too low", "Object ID too high", "Object not in heap", "Unknown heap", "Unknown object (invalid DefProc)", "Unknown object (DefProc not in table)", "Message out of range", "Invalid (null) method", "Unknown message", "Manager call not supported", "Bad address", "Network operation in progress", "Network operation timed out", "Connection is busy", "Network attribute not supported", "Network error", "Address in use", "System out of memory", "Connection aborted", "Connection refused", "Not connected", "Already connected", "Connection closed", "Initialization error (interapplication manager)", "Bad occurrence", "Wait on unbound occurrence handler", "Occurrence queue overflow", "Datalog type conflict", "Unused", "Unrecognized type (interapplication manager)", "Memory corrupt", "Failed to make temporary DLL", "Old CIN version", "Drag socket not found", "Failed to load drop-object", "Failed to register OLE object", "Failed to release OLE object", "Format specifier type mismatch", "Unknown format specifier", "Too few format specifiers", "Too many format specifiers", "Scan failed", "Newer CIN version", "Error converting to variant", "Runtime menu error", "Password tampered", "Variant attribute not found", "Incompatible variant data type", "Event data is not available", "Event Store is not present", "Occurrence is not found", "Event Queue is not created", "Event info is not available", "Refnum passed is NULL", "Error retrieving Class GUID", "Error retrieving CoClass GUID", "Error retrieving TypeLib GUID.", "Bad built application magic bytes.", "Specific driver is different from the specific driver associated with the Logical Name.", "There is no session opened to the class driver.", "Max Error", "MAX - Error with config objects", "MAX - Error loading configuration", "MAX - Group not supported"]
        # "Current State"
        # "Do not delete, rename, or modify this frame.\n(this is used to capture unhandled states and typos)"
        # "Handle mistyped state name (developer tool)"
        n483 = Format Into String(format string="Software Exception: Unhandled State \"%s\"." ("message"), error in=w1052, w1047) -> (resulting string=w1055:string, error out=w1054:errorcluster)  [unwired: 1 in]
        n484 = call <vilib>:"Error Cluster From Error Code.vi"("show call chain? (False)"=TRUE, "error in (no error)"=w1054, "error message (\"\")"=w1055, "error code (0)"=w1056) -> ("error out"=w1053:errorcluster)  [unwired: 5 in]
        n485 = call <vilib>:"Add State(s) to Queue__JKI_lib_State_Machine.vi"("State(s) in (\"\")"=w1051) -> ("States Out"=w1050:string)  [unwired: 14 in]
      }
      frame "Initialize Core Data" {
        # "Build default path based on the location of project"
        # "Do not delete, rename, or modify this frame.\n(this is used to determine panel behavior on exit)"
        # "originally closed?"
        # "exe?"
        # "If panel starts closed or is an EXE, then close it when we exit"
        n486 = call <vilib>:"Application Directory.vi"() -> ("Application Directory"=w1060:path)
        n487 = property on="Property Node" class="App"() -> ("App.Kind"=w1074:T21)  [unwired: 2 in, 2 out]
        n488 = property on="Property Node" class="VI"() -> ("FP.State"=w1068:T20)  [unwired: 2 in, 2 out]
        n489 = control-ref of="Current VI Reference"() -> (w1069:refnum<vi>)
        n490 = Equal?(x=w1068, y=T20."Closed" ("Front Panel Window:State")) -> (x = y?=w1066:bool)
        n491 = Equal?(x=w1074, y=T21."Run Time System" ("Application:Kind")) -> (x = y?=w1072:bool)
        n492 = Build Path(base path=w1060, name or relative path="Data") -> (appended path=w1064:path)
        n493 = Build Path(base path=w1060, name or relative path="SystemTemp") -> (appended path=w1061:path)
        n494 = Build Path(base path=w1060, name or relative path="SystemCalibrationFile") -> (appended path=w1058:path)
        n495 = Or(x=w1066, y=w1072) -> (x .or. y?=w1070:bool)
        n496 = Bundle By Name(cluster=w1071, "Core.Current VI Reference"=w1069, "Core.Close Panel on Exit?"=w1070, "DefaultPath"=w1064, "TempPath"=w1061, "CaliPath"=w1058) -> (w1076:T25)
        n497 = call <vilib>:"Add State(s) to Queue__JKI_lib_State_Machine.vi"("State(s) in (\"\")"=w1078) -> ("States Out"=w1077:string)  [unwired: 14 in]
      }
      frame "Error Handler" {
        # "Unhandled Error -- Display it"
        # "Handle any errors here.\nYou can also output any states to clean-up after errors occur"
        # "Clear error"
        n498 = Unbundle By Name(w1079) -> ("code"=w1081:i32)
        n499 = case shown="5001" w1081 {
          tunnel: ["Macro: Exit" w1091 w1097] -> w1080
          tunnel: w1079 -> [w1087 _ _]
          frame Default {
            w1089 = T39 1 items=["no dialog", "OK message", "continue or stop message", "OK message + warnings", "continue/stop + warnings"] ("type of dialog (OK msg:1)")
            n500 = call <vilib>:"General Error Handler.vi"("type of dialog (OK msg:1)"=w1089, "error in (no error)"=w1087) -> ()  [unwired: 9 in, 5 out]
          }
          frame 5002 {
            n501 = Two Button Dialog(message="Laser interlock open! Please close interlock and try again! ", 1:"Safely Shutdown" ("F button name (\"Cancel\")"), 2:"OK" ("T button name (\"OK\")")) -> (T button?=w1092:bool)
            n502 = case shown="True" w1092 {
              tunnel: ["Macro: Exit" "355 Laser: CheckControllerStatus"] -> w1091
              frame False {
              }
              frame True {
              }
            }
          }
          frame 5001 {
            n503 = Two Button Dialog(message="Unable to connect to imaging computer, do you want to run data aquisiton alone? ", 1:"No" ("F button name (\"Cancel\")"), 2:"Yes" ("T button name (\"OK\")")) -> (T button?=w1098:bool)
            n504 = case shown="False" w1098 {
              tunnel: ["Macro: Exit" "" ("Empty String Constant")] -> w1097
              frame False {
              }
              frame True {
              }
            }
          }
        }
        n505 = call <vilib>:"Add State(s) to Queue__JKI_lib_State_Machine.vi"("State(s) in Front (\"\")"=w1080, "State(s) in (\"\")"=w1086) -> ("States Out"=w1085:string)  [unwired: 13 in]
      }
      frame "Exit" {
        # "Do not put any code in this frame.\n(No errors that occur here will be handled.)"
        n506 = call <vilib>:"Add State(s) to Queue__JKI_lib_State_Machine.vi"("State(s) in (\"\")"=w1109) -> ("States Out"=w1108:string)  [unwired: 14 in]
      }
      frame "---------- Case ----------" {
        # "Template Separator\n(You can make a copy of, or modify, this frame)"
        n507 = call <vilib>:"Add State(s) to Queue__JKI_lib_State_Machine.vi"("State(s) in (\"\")"=w1114) -> ("States Out"=w1113:string)  [unwired: 14 in]
      }
      frame "Case: getCaliID" {
        # "Get Calibration file #\n(You can make a copy of, or modify, this frame)"
        n508 = Unbundle By Name(w1115) -> ("Pathes.CaliPath"=w1118:path)
        n509 = call <vilib>:"Recursive File List.vi"("pattern"="*.tdms", "Treat LLBs as Folders?"=FALSE, "Folder Path"=w1118) -> ("All Files in Dir"=w1123:path[])  [unwired: 4 in, 4 out]
        n510 = for {
          tunnel: w1123 -> [w1133] mode=indexing
          tunnel: [w1132] -> w1122 mode=indexing
          tunnel: "Calibration" -> [w1129]
          n511 = Strip Path(path=w1133) -> (name=w1130:string)  [unwired: 1 out]
          n512 = Search and Replace String(input string=w1130, search string=w1129) -> (result string=w1128:string)  [unwired: 6 in, 3 out]
          n513 = Scan From String(format string="%d" ("string"), input string=w1128) -> (output 1=w1132:i32)  [unwired: 3 in, 3 out]
        }
        n514 = Array Max & Min(array=w1122) -> (max value=w1121:i32)  [unwired: 3 out]
        n515 = Bundle By Name(cluster=w1115, "IDs.Cali ID"=w1121) -> (w1116:T25)
        n516 = call <vilib>:"Add State(s) to Queue__JKI_lib_State_Machine.vi"("State(s) in (\"\")"=w1127) -> ("States Out"=w1126:string)  [unwired: 14 in]
      }
      frame "Case: getBGID" {
        # "Get background #\n(You can make a copy of, or modify, this frame)"
        n517 = Unbundle By Name(w1136) -> ("Pathes.BG Path"=w1141:path)
        n518 = call <vilib>:"Recursive File List.vi"("pattern"="*.tdms", "Treat LLBs as Folders?"=FALSE, "Folder Path"=w1141) -> ("All Files in Dir"=w1139:path[])  [unwired: 4 in, 4 out]
        n519 = for {
          tunnel: w1139 -> [w1156] mode=indexing
          tunnel: "Background" ("name or relative path") -> [w1154]
          shift-right: [w1147] -> w1134
          shift-left: 0 -> [w1151]
          n520 = Strip Path(path=w1156) -> (name=w1155:string)  [unwired: 1 out]
          n521 = Search and Replace String(input string=w1155, search string=w1154) -> (number of replacements=w1153:i32)  [unwired: 6 in, 3 out]
          n522 = Greater Than 0?(x=w1153) -> (x > 0?=w1152:bool)
          n523 = Select(t=1, s=w1152, f=0) -> (s? t:f=w1150:i32)
          n524 = Add(x=w1150, y=w1151) -> (x+y=w1147:i32)
        }
        n525 = Bundle By Name(cluster=w1136, "IDs.BG ID"=w1134) -> (w1137:T25)
        n526 = call <vilib>:"Add State(s) to Queue__JKI_lib_State_Machine.vi"("State(s) in (\"\")"=w1146) -> ("States Out"=w1145:string)  [unwired: 14 in]
      }
      frame "Case: getRunID" {
        # "Check folder for run ID\n(You can make a copy of, or modify, this frame)"
        n527 = Unbundle By Name(w1166) -> ("Pathes.DataPath"=w1165:path, "CaseID"=w1161:string)
        n528 = Build Array("Background" ("name or relative path"), "Calibration", "3DScanData" ("element")) -> (w1171:string[])
        n529 = call <vilib>:"Recursive File List.vi"("Folders to Exclude"=w1171, "pattern"="*.tdms", "Treat LLBs as Folders?"=FALSE, "Folder Path"=w1165) -> ("All Files in Dir"=w1162:path[])  [unwired: 3 in, 4 out]
        n530 = for {
          tunnel: w1162 -> [w1180] mode=indexing
          tunnel: [w1179] -> w1168 mode=indexing
          tunnel: w1161 -> [w1176]
          n531 = Strip Path(path=w1180) -> (name=w1177:string)  [unwired: 1 out]
          n532 = Search and Replace String(input string=w1177, search string=w1176) -> (result string=w1175:string)  [unwired: 6 in, 3 out]
          n533 = Scan From String(format string="_%d" ("string"), input string=w1175) -> (output 1=w1179:i32)  [unwired: 3 in, 3 out]
        }
        n534 = Array Max & Min(array=w1168) -> (max value=w1159:i32)  [unwired: 3 out]
        n535 = Bundle By Name(cluster=w1166, "IDs.RunID"=w1159) -> (w1167:T25)
        n536 = call "RunIDFGV.vi"("Error In"=w1157, "RunID in"=w1159) -> ("Error Out"=w1158:errorcluster)  [unwired: 8 in, 1 out]
        n537 = call <vilib>:"Add State(s) to Queue__JKI_lib_State_Machine.vi"("State(s) in (\"\")"=w1174) -> ("States Out"=w1173:string)  [unwired: 14 in]
      }
      frame "Case: CreatFileStruct" {
        # "Creat case file structure"
        n538 = Unbundle By Name(w1194) -> ("DefaultPath"=w1200:path, "CaseID"=w1187:string)
        n539 = Build Path(base path=w1200, name or relative path=w1187) -> (appended path=w1199:path)
        n540 = call <vilib>:"Check if File or Folder Exists.vi"("error in (no error)"=w1193, "path"=w1199) -> ("error out"=w1196:errorcluster, "file or folder exists?"=w1198:bool, "dup path"=w1197:path)  [unwired: 7 in]
        n541 = case shown="True" w1198 {
          tunnel: w1197 -> [w1217 w1225]
          tunnel: w1196 -> [w1215 w1220]
          tunnel: [w1209 w1225] -> w1185
          tunnel: [w1213 w1227] -> w1184
          tunnel: [u32 0 u32 0] -> w1183
          tunnel: [w1211 w1230] -> w1191
          tunnel: "Background" ("name or relative path") -> [w1210 w1222]
          tunnel: "Calibration" -> [w1208 w1221]
          tunnel: [w1204 w1223] -> w1188
          tunnel: w1187 -> [_ _]
          tunnel: ["" ("Empty String Constant") "Case: getRunID\nCase: getBGID\nCase: getCaliID\nUI: Update"] -> w1186
          frame False {
            # "Folder not exist. Creat folders."
            n542 = Create Folder(path (use dialog)=w1217, error in=w1215) -> (created path=w1209:path, error out=w1206:errorcluster)  [unwired: 1 in, 1 out]
            n543 = Build Path(base path=w1209, name or relative path=w1208) -> (appended path=w1207:path)
            n544 = Build Path(base path=w1209, name or relative path=w1210) -> (appended path=w1216:path)
            n545 = Create Folder(path (use dialog)=w1216, error in=w1206) -> (created path=w1211:path, error out=w1212:errorcluster)  [unwired: 1 in, 1 out]
            n546 = Create Folder(path (use dialog)=w1207, error in=w1206) -> (created path=w1204:path, error out=w1205:errorcluster)  [unwired: 1 in, 1 out]
            n547 = Merge Errors(w1212, w1205) -> (w1213:errorcluster)
          }
          frame True {
            # "Folder exsit, check file #"
            n548 = Build Path(base path=w1225, name or relative path=w1221) -> (appended path=w1226:path)
            n549 = Build Path(base path=w1225, name or relative path=w1222) -> (appended path=w1231:path)
            n550 = call <vilib>:"Check if File or Folder Exists.vi"("path"=w1226) -> ("file or folder exists?"=w1224:bool, "dup path"=w1223:path)  [unwired: 8 in, 1 out]
            n551 = call <vilib>:"Check if File or Folder Exists.vi"("path"=w1231) -> ("file or folder exists?"=w1229:bool, "dup path"=w1230:path)  [unwired: 8 in, 1 out]
            n552 = And(x=w1229, y=w1224) -> (x .and. y?=w1228:bool)
            n553 = case shown="False" w1228 {
              tunnel: w1220 -> [_ w1233]
              tunnel: [errorcluster {"status"=TRUE, "code"=5003, "source"="File structure error."} ("error out") w1233] -> w1227
              frame False {
              }
              frame True {
              }
            }
          }
        }
        n554 = Bundle By Name(cluster=w1194, "Pathes.DataPath"=w1185, "Pathes.BG Path"=w1191, "Pathes.CaliPath"=w1188, "IDs.RunID"=w1183, "IDs.BG ID"=w1183, "IDs.Cali ID"=w1183) -> (w1195:T25)
        n555 = call "DataRootPathFGV.vi"("Error In"=w1184, "PathIn"=w1185) -> ("Error Out"=w1182:errorcluster)  [unwired: 8 in, 1 out]
        n556 = call "RunIDFGV.vi"("Error In"=w1182, "RunID in"=w1183) -> ("Error Out"=w1181:errorcluster)  [unwired: 8 in, 1 out]
        n557 = call <vilib>:"Add State(s) to Queue__JKI_lib_State_Machine.vi"("State(s) in Front (\"\")"=w1186, "State(s) in (\"\")"=w1202) -> ("States Out"=w1201:string)  [unwired: 13 in]
      }
      frame "Case: GetID" {
        # "Template Separator\n(You can make a copy of, or modify, this frame)"
        n558 = call "set_subjectID.vi"() -> ("subject_id"=w1234:string)  [unwired: 10 in]
        n559 = Bundle By Name(cluster=w1236, "CaseID"=w1234) -> (w1237:T25)
        n560 = call <vilib>:"Add State(s) to Queue__JKI_lib_State_Machine.vi"("State(s) in (\"\")"=w1240) -> ("States Out"=w1239:string)  [unwired: 14 in]
      }
      frame "---------- DeconEngine ----------" {
        # "start data aquisition and then set irfAligh to ture and decon channel to 1,2 and 3."
        # "Template Separator\n(You can make a copy of, or modify, this frame)"
        n561 = call <vilib>:"Add State(s) to Queue__JKI_lib_State_Machine.vi"("State(s) in (\"\")"=w1245) -> ("States Out"=w1244:string)  [unwired: 14 in]
      }
      frame "DeconEngine: InitilizeMacro" {
        # "start data aquisition and then set irfAligh to ture and decon channel to 1,2 and 3."
        # "Initilize Decon Engine for all channel\n(You can make a copy of, or modify, this frame)"
        n562 = call <vilib>:"Add State(s) to Queue__JKI_lib_State_Machine.vi"("State(s) in Front (\"\")"="DeconEngine: InitializeCh1\nDeconEngine: InitializeCh2\nDeconEngine: InitializeCh3" ("State(s) in Front (\"\")"), "State(s) in (\"\")"=w1251) -> ("States Out"=w1250:string)  [unwired: 13 in]
      }
      frame "DeconEngine: InitializeCh1" {
        w1275 = refnum<class "LaguerreDeconEngineClass.lvclass"> refnum  # Ch1DeconObj
        # "Initilize Laguerre Deconvolution engine Object\n(You can make a copy of, or modify, this frame)"
        n563 = call "FLImDAQ_FGV.vi"("error in (no error)"=w1260) -> ("error out"=w1271:errorcluster, "Read data"=w1270:T6)  [unwired: 9 in]
        n564 = global read "GlobalVariables.vi" "LastUseiRF"() -> (w1253:T40)
        n565 = Unbundle By Name(w1270) -> ("min record length"=w1269:i32)
        n566 = call "setLaguerreOrder.vi"("error in (no error)"=w1271, "LaguerreOrder"=u32 12, "LaguerreDeconClass in"=w1275) -> ("error out"=w1272:errorcluster, "LaguerreDeconClass out"=w1273:refnum<class "LaguerreDeconEngineClass.lvclass">)  [unwired: 7 in]
        n567 = Unbundle By Name(w1253) -> ("Ch1 iRF"=w1252:dbl[])
        n568 = call "setDataLength.vi"("error in (no error)"=w1272, "dataLength"=w1269, "LaguerreDeconClass in"=w1273) -> ("error out"=w1268:errorcluster, "LaguerreDeconClass out"=w1267:refnum<class "LaguerreDeconEngineClass.lvclass">)  [unwired: 7 in]
        n569 = call "setIRF.vi"("error in (no error)"=w1268, "iRF"=w1252, "LaguerreDeconClass in"=w1267) -> ("error out"=w1265:errorcluster, "LaguerreDeconClass out"=w1266:refnum<class "LaguerreDeconEngineClass.lvclass">)  [unwired: 7 in]
        n570 = call "computeAlpha.vi"("error in (no error)"=w1265, "LaguerreDeconClass in"=w1266) -> ("error out"=w1263:errorcluster, "LaguerreDeconClass out"=w1264:refnum<class "LaguerreDeconEngineClass.lvclass">)  [unwired: 8 in]
        n571 = call "dataInitilize.vi"("error in (no error)"=w1263, "LaguerreDeconClass in"=w1264) -> ("error out"=w1261:errorcluster, "LaguerreDeconClass out"=w1262:refnum<class "LaguerreDeconEngineClass.lvclass">)  [unwired: 8 in]
        n572 = call "computeDeconMatrix.vi"("error in (no error)"=w1261, "LaguerreDeconClass in"=w1262) -> ("error out"=w1257:errorcluster, "LaguerreDeconClass out"=w1259:refnum<class "LaguerreDeconEngineClass.lvclass">)  [unwired: 8 in]
        n573 = call "Ch1DeconEngineFGV.vi"("Error In"=w1257, "action(read)"=enum16{"write", "read"}."write" ("action"), "Ch1DeconEngine in"=w1259) -> ("Error Out"=w1256:errorcluster)  [unwired: 7 in, 1 out]
        n574 = call <vilib>:"Add State(s) to Queue__JKI_lib_State_Machine.vi"("State(s) in (\"\")"=w1277) -> ("States Out"=w1276:string)  [unwired: 14 in]
      }
      frame "DeconEngine: InitializeCh2" {
        w1301 = refnum<class "LaguerreDeconEngineClass.lvclass"> refnum  # Ch2DeconObj
        # "Initilize Laguerre Deconvolution engine Object\n(You can make a copy of, or modify, this frame)"
        n575 = global read "GlobalVariables.vi" "LastUseiRF"() -> (w1279:T40)
        n576 = call "FLImDAQ_FGV.vi"("error in (no error)"=w1287) -> ("error out"=w1280:errorcluster, "Read data"=w1297:T6)  [unwired: 9 in]
        n577 = call "setLaguerreOrder.vi"("error in (no error)"=w1280, "LaguerreOrder"=u32 12, "LaguerreDeconClass in"=w1301) -> ("error out"=w1298:errorcluster, "LaguerreDeconClass out"=w1299:refnum<class "LaguerreDeconEngineClass.lvclass">)  [unwired: 7 in]
        n578 = Unbundle By Name(w1297) -> ("min record length"=w1296:i32)
        n579 = Unbundle By Name(w1279) -> ("Ch2 iRF"=w1278:dbl[])
        n580 = call "setDataLength.vi"("error in (no error)"=w1298, "dataLength"=w1296, "LaguerreDeconClass in"=w1299) -> ("error out"=w1295:errorcluster, "LaguerreDeconClass out"=w1294:refnum<class "LaguerreDeconEngineClass.lvclass">)  [unwired: 7 in]
        n581 = call "setIRF.vi"("error in (no error)"=w1295, "iRF"=w1278, "LaguerreDeconClass in"=w1294) -> ("error out"=w1292:errorcluster, "LaguerreDeconClass out"=w1293:refnum<class "LaguerreDeconEngineClass.lvclass">)  [unwired: 7 in]
        n582 = call "computeAlpha.vi"("error in (no error)"=w1292, "LaguerreDeconClass in"=w1293) -> ("error out"=w1290:errorcluster, "LaguerreDeconClass out"=w1291:refnum<class "LaguerreDeconEngineClass.lvclass">)  [unwired: 8 in]
        n583 = call "dataInitilize.vi"("error in (no error)"=w1290, "LaguerreDeconClass in"=w1291) -> ("error out"=w1288:errorcluster, "LaguerreDeconClass out"=w1289:refnum<class "LaguerreDeconEngineClass.lvclass">)  [unwired: 8 in]
        n584 = call "computeDeconMatrix.vi"("error in (no error)"=w1288, "LaguerreDeconClass in"=w1289) -> ("error out"=w1284:errorcluster, "LaguerreDeconClass out"=w1286:refnum<class "LaguerreDeconEngineClass.lvclass">)  [unwired: 8 in]
        n585 = call "Ch2DeconEngineFGV.vi"("Error In"=w1284, "action(read)"=enum16{"write", "read"}."write" ("action"), "Ch2DeconEngine in"=w1286) -> ("Error Out"=w1283:errorcluster)  [unwired: 7 in, 1 out]
        n586 = call <vilib>:"Add State(s) to Queue__JKI_lib_State_Machine.vi"("State(s) in (\"\")"=w1303) -> ("States Out"=w1302:string)  [unwired: 14 in]
      }
      frame "DeconEngine: InitializeCh3" {
        w1304 = refnum<class "LaguerreDeconEngineClass.lvclass"> refnum  # Ch3DeconObj
        # "Initilize Laguerre Deconvolution engine Object\n(You can make a copy of, or modify, this frame)"
        n587 = call "FLImDAQ_FGV.vi"("error in (no error)"=w1313) -> ("error out"=w1324:errorcluster, "Read data"=w1323:T6)  [unwired: 9 in]
        n588 = global read "GlobalVariables.vi" "LastUseiRF"() -> (w1306:T40)
        n589 = call "setLaguerreOrder.vi"("error in (no error)"=w1324, "LaguerreOrder"=u32 12, "LaguerreDeconClass in"=w1304) -> ("error out"=w1325:errorcluster, "LaguerreDeconClass out"=w1326:refnum<class "LaguerreDeconEngineClass.lvclass">)  [unwired: 7 in]
        n590 = Unbundle By Name(w1323) -> ("min record length"=w1322:i32)
        n591 = Unbundle By Name(w1306) -> ("Ch3 iRF"=w1305:dbl[])
        n592 = call "setDataLength.vi"("error in (no error)"=w1325, "dataLength"=w1322, "LaguerreDeconClass in"=w1326) -> ("error out"=w1321:errorcluster, "LaguerreDeconClass out"=w1320:refnum<class "LaguerreDeconEngineClass.lvclass">)  [unwired: 7 in]
        n593 = call "setIRF.vi"("error in (no error)"=w1321, "iRF"=w1305, "LaguerreDeconClass in"=w1320) -> ("error out"=w1318:errorcluster, "LaguerreDeconClass out"=w1319:refnum<class "LaguerreDeconEngineClass.lvclass">)  [unwired: 7 in]
        n594 = call "computeAlpha.vi"("error in (no error)"=w1318, "LaguerreDeconClass in"=w1319) -> ("error out"=w1316:errorcluster, "LaguerreDeconClass out"=w1317:refnum<class "LaguerreDeconEngineClass.lvclass">)  [unwired: 8 in]
        n595 = call "dataInitilize.vi"("error in (no error)"=w1316, "LaguerreDeconClass in"=w1317) -> ("error out"=w1314:errorcluster, "LaguerreDeconClass out"=w1315:refnum<class "LaguerreDeconEngineClass.lvclass">)  [unwired: 8 in]
        n596 = call "computeDeconMatrix.vi"("error in (no error)"=w1314, "LaguerreDeconClass in"=w1315) -> ("error out"=w1310:errorcluster, "LaguerreDeconClass out"=w1312:refnum<class "LaguerreDeconEngineClass.lvclass">)  [unwired: 8 in]
        n597 = call "Ch3DeconEngineFGV.vi"("Error In"=w1310, "action(read)"=enum16{"write", "read"}."write" ("action"), "Ch3DeconEngine in"=w1312) -> ("Error Out"=w1309:errorcluster)  [unwired: 7 in, 1 out]
        n598 = call <vilib>:"Add State(s) to Queue__JKI_lib_State_Machine.vi"("State(s) in (\"\")"=w1329) -> ("States Out"=w1328:string)  [unwired: 14 in]
      }
      frame "---------- Digitizer ----------" {
        # "Template Separator\n(You can make a copy of, or modify, this frame)"
        n599 = call <vilib>:"Add State(s) to Queue__JKI_lib_State_Machine.vi"("State(s) in (\"\")"=w1334) -> ("States Out"=w1333:string)  [unwired: 14 in]
      }
      frame "Digitizer: Initialize" {
        # "reset digitizer to everytime the system runs"
        # "reset digitizer to everytime the system runs"
        # "Initialize digitizer.\nInitialize both digitizer and update status."
        n600 = call "FLImDAQ_FGV.vi"("error in (no error)"=w1342) -> ("error out"=w1336:errorcluster, "Read data"=w1341:T6)  [unwired: 9 in]
        n601 = Unbundle By Name(w1344) -> ("SysConfigCluster.Ch1Enable?"=w1349:bool, "SysConfigCluster.Ch2Enable?"=w1348:bool, "SysConfigCluster.Ch3Enable?"=w1346:bool)
        n602 = Unbundle By Name(w1341) -> ("Digitizer 1"=w1337:refnum<k15>, "Digitizer 2"=w1340:refnum<k15>)
        n603 = property on="Digitizer" class="Bool (strict)"("Blinking"=TRUE) -> ()  [unwired: 2 in, 2 out]
        n604 = Or(x=w1349, y=w1348) -> (x .or. y?=w1347:bool)
        n605 = case shown="True" w1347 {
          tunnel: w1336 -> [w1357 w1360]
          tunnel: [w1357 w1359] -> w1338
          tunnel: w1337 -> [_ w1361]
          frame False {
          }
          frame True {
            n606 = call <instrlib>:"niScope Initialize.vi"("resource name"=w1361, "reset device"=TRUE, "error in"=w1360) -> ("error out"=w1359:errorcluster)  [unwired: 11 in, 1 out]
          }
        }
        n607 = case shown="True" w1346 {
          tunnel: w1336 -> [w1352 w1354]
          tunnel: [w1352 w1356] -> w1343
          tunnel: w1340 -> [_ w1355]
          frame False {
          }
          frame True {
            n608 = call <instrlib>:"niScope Initialize.vi"("resource name"=w1355, "reset device"=TRUE, "error in"=w1354) -> ("error out"=w1356:errorcluster)  [unwired: 11 in, 1 out]
          }
        }
        n609 = Merge Errors(w1338, w1343) -> (w1335:errorcluster)
        n610 = call <vilib>:"Add State(s) to Queue__JKI_lib_State_Machine.vi"("State(s) in (\"\")"=w1351) -> ("States Out"=w1350:string)  [unwired: 14 in]
      }
      frame "Digitizer: Config" {
        # "Synchronize is taking time ~3s."
        # "Config  digitizer\nCall subVi to config digitizer"
        n611 = call "FLImDAQ_FGV.vi"() -> ("Read data"=w1379:T6)  [unwired: 10 in, 1 out]
        n612 = Unbundle By Name(w1388) -> ("SysConfigCluster.Ch1Enable?"=w1396:bool, "SysConfigCluster.Ch2Enable?"=w1395:bool, "SysConfigCluster.Ch3Enable?"=w1393:bool, "FLImDAQ"=w1390:T32)
        n613 = Unbundle By Name(w1379) -> ("Digitizer 1"=w1382:refnum<k15>, "Digitizer 2"=w1381:refnum<k15>)
        n614 = property on="Digitizer" class="Bool (strict)"(error in=w1383, "Blinking"=TRUE) -> (error out=w1384:errorcluster)  [unwired: 1 in, 1 out]
        n615 = Or(x=w1396, y=w1395) -> (x .or. y?=w1394:bool)
        n616 = case shown="True" w1394 {
          tunnel: w1390 -> [_ w1409]
          tunnel: w1384 -> [w1405 w1408]
          tunnel: [w1405 w1407] -> w1391
          tunnel: w1382 -> [_ w1406]
          frame False {
          }
          frame True {
            n617 = call "DigitizerConfig.vi"("error in (no error)"=w1408, "FLImDAQ"=w1409, "IVI Refnum in"=w1406) -> ("error out"=w1407:errorcluster)  [unwired: 7 in, 1 out]
          }
        }
        n618 = case shown="True" w1393 {
          tunnel: w1390 -> [_ w1404]
          tunnel: w1391 -> [w1399 w1403]
          tunnel: [w1399 w1402] -> w1367
          tunnel: w1381 -> [_ w1400]
          frame False {
          }
          frame True {
            n619 = call "DigitizerConfig.vi"("Config Trigger? (T)"=FALSE ("Config Trigge(T)r:"), "error in (no error)"=w1403, "FLImDAQ"=w1404, "IVI Refnum in"=w1400) -> ("error out"=w1402:errorcluster)  [unwired: 6 in, 1 out]
          }
        }
        n620 = call "Digitizer1_FGV.vi"("error in (no error)"=w1367) -> ("error out"=w1377:errorcluster, "Read data"=w1378:refnum<k15>)  [unwired: 9 in]
        n621 = call <instrlib>:"niScope Get Session Reference.vi"("instrument handle"=w1378, "error in"=w1377) -> ("session reference"=w1371:refnum<k20>, "error out"=w1369:errorcluster)  [unwired: 11 in, 1 out]
        n622 = call "Digitizer2_FGV.vi"("error in (no error)"=w1369) -> ("error out"=w1375:errorcluster, "Read data"=w1376:refnum<k15>)  [unwired: 9 in]
        n623 = call <instrlib>:"niScope Get Session Reference.vi"("instrument handle"=w1376, "error in"=w1375) -> ("session reference"=w1370:refnum<k20>, "error out"=w1368:errorcluster)  [unwired: 11 in, 1 out]
        n624 = Build Array(w1371, w1370) -> (w1374:refnum<k20>[])
        n625 = call <instrlib>:"niTClk Configure For Homogeneous Triggers.vi"("error in (no error)"=w1368, "sessions"=w1374) -> ("error out"=w1373:errorcluster, "sessions out"=w1372:refnum<k20>[])  [unwired: 8 in]
        n626 = call <instrlib>:"niTClk Synchronize.vi"("error in (no error)"=w1373, "sessions"=w1372) -> ("error out"=w1366:errorcluster, "sessions out"=w1364:refnum<k20>[])  [unwired: 8 in]
        n627 = call <userlib>:"Wait (ms)__ogtk.vi"("error in (no error)"=w1366, "milliseconds to wait"=u32 1500) -> ("error out"=w1362:errorcluster)  [unwired: 8 in, 1 out]
        n628 = Unbundle By Name(w1362) -> ("status"=w1387:bool)
        n629 = Not(x=w1387) -> (.not. x?=w1386:bool)
        n630 = Bundle By Name(cluster=w1388, "System Status.Digitizer"=w1386, "niTClk sessions"=w1364) -> (w1389:T25)
        n631 = property on="Digitizer" class="Bool (strict)"(error in=w1362, "Blinking"=FALSE) -> (error out=w1380:errorcluster)  [unwired: 1 in, 1 out]
        n632 = call <vilib>:"Add State(s) to Queue__JKI_lib_State_Machine.vi"("State(s) in (\"\")"=w1398) -> ("States Out"=w1397:string)  [unwired: 14 in]
      }
      frame "Digitizer: Start" {
        # "send trigger to start acquisition loop"
        # "initilize aquisition"
        # "Start Digitizer\n(TClk start)"
        n633 = Unbundle By Name(w1417) -> ("niTClk sessions"=w1416:refnum<k20>[])
        n634 = call <instrlib>:"niTClk Initiate.vi"("error in (no error)"=w1410, "sessions"=w1416) -> ("error out"=w1412:errorcluster)  [unwired: 8 in, 1 out]
        n635 = Generate User Event(priority (normal)=usereventprio."high priority", user event=w1413, event data cluster=TRUE ("event data"), error in=w1412) -> (error out=w1411:errorcluster)  [unwired: 1 out]
        n636 = call <vilib>:"Add State(s) to Queue__JKI_lib_State_Machine.vi"("State(s) in (\"\")"=w1420) -> ("States Out"=w1419:string)  [unwired: 14 in]
      }
      frame "Digitizer: Abort" {
        # "Template Separator\n(You can make a copy of, or modify, this frame)"
        n637 = call "Digitizer1_FGV.vi"("error in (no error)"=w1424, "Operation (Read)"=enum16{"Write", "Read"}."Read" ("Operation")) -> ("error out"=w1431:errorcluster, "Read data"=w1428:refnum<k15>)  [unwired: 8 in]
        n638 = call "Digitizer2_FGV.vi"("error in (no error)"=w1424, "Operation (Read)"=enum16{"Write", "Read"}."Read" ("Operation")) -> ("error out"=w1427:errorcluster, "Read data"=w1429:refnum<k15>)  [unwired: 8 in]
        n639 = Bundle By Name(cluster=w1421, "SysRunning?"=FALSE ("System Status")) -> (w1422:T25)
        n640 = call <instrlib>:"niScope Abort.vi"("instrument handle"=w1428, "error in"=w1431) -> ("error out"=w1433:errorcluster)  [unwired: 12 in, 1 out]
        n641 = call <instrlib>:"niScope Abort.vi"("instrument handle"=w1429, "error in"=w1427) -> ("error out"=w1432:errorcluster)  [unwired: 12 in, 1 out]
        n642 = Merge Errors(w1433, w1432) -> (w1425:errorcluster)
        n643 = call <vilib>:"Add State(s) to Queue__JKI_lib_State_Machine.vi"("State(s) in (\"\")"=w1436) -> ("States Out"=w1435:string)  [unwired: 14 in]
      }
      frame "Digitizer: checkTemp" {
        w1439 = 65.0 ("y")
        w1444 = enum16{"Write", "Read"}."Read" ("Operation")
        # "Template Separator\n(You can make a copy of, or modify, this frame)"
        n644 = call "Digitizer1_FGV.vi"("Operation (Read)"=w1444) -> ("error out"=w1445:errorcluster, "Read data"=w1446:refnum<k15>)  [unwired: 9 in]
        n645 = call "Digitizer2_FGV.vi"("Operation (Read)"=w1444) -> ("error out"=w1442:errorcluster, "Read data"=w1443:refnum<k15>)  [unwired: 9 in]
        n646 = property on="Property Node" class="niScope"(reference=w1443, error in=w1442) -> ("Device Temperature"=w1440:dbl)  [unwired: 2 out]
        "Dig2 Temp" <- w1440
        n647 = property on="Property Node" class="niScope"(reference=w1446, error in=w1445) -> ("Device Temperature"=w1441:dbl)  [unwired: 2 out]
        "Dig1 Temp" <- w1441
        n648 = Greater?(x=w1441, y=w1439) -> (0:w1438:bool)
        n649 = Greater?(x=w1440, y=w1439) -> (0:w1437:bool)
        n650 = case shown="True" w1438 {
          frame False {
          }
          frame True {
            n651 = One Button Dialog(message="Digitizer 1 over heating!", button name ("OK")="OK") -> ()  [unwired: 1 out]
          }
        }
        n652 = case shown="True" w1437 {
          frame False {
          }
          frame True {
            n653 = One Button Dialog(message="Digitizer 2 over heating!", button name ("OK")="OK") -> ()  [unwired: 1 out]
          }
        }
        n654 = call <vilib>:"Add State(s) to Queue__JKI_lib_State_Machine.vi"("State(s) in (\"\")"=w1451) -> ("States Out"=w1450:string)  [unwired: 14 in]
      }
      frame "Digitizer: Close" {
        # "Close Digitizer"
        n655 = call "Digitizer1_FGV.vi"("error in (no error)"=w1461, "Operation (Read)"=enum16{"Write", "Read"}."Read" ("Operation")) -> ("error out"=w1463:errorcluster, "Read data"=w1467:refnum<k15>)  [unwired: 8 in]
        n656 = call "Digitizer2_FGV.vi"("error in (no error)"=w1461, "Operation (Read)"=enum16{"Write", "Read"}."Read" ("Operation")) -> ("error out"=w1462:errorcluster, "Read data"=w1465:refnum<k15>)  [unwired: 8 in]
        n657 = call <instrlib>:"niScope Close.vi"("instrument handle"=w1467, "error in"=w1463) -> ("error out"=w1460:errorcluster)  [unwired: 13 in]
        n658 = call <instrlib>:"niScope Close.vi"("instrument handle"=w1465, "error in"=w1462) -> ("error out"=w1459:errorcluster)  [unwired: 13 in]
        n659 = Merge Errors(w1460, w1459) -> (w1458:errorcluster)
        n660 = Unbundle By Name(w1458) -> ("status"=w1457:bool)
        n661 = Bundle By Name(cluster=w1468, "System Status.Digitizer"=w1457) -> (w1469:T25)
        n662 = call <vilib>:"Add State(s) to Queue__JKI_lib_State_Machine.vi"("State(s) in (\"\")"=w1471) -> ("States Out"=w1470:string)  [unwired: 14 in]
      }
      frame "---------- LabJack ----------" {
        # "Template Separator\n(You can make a copy of, or modify, this frame)"
        n663 = call <vilib>:"Add State(s) to Queue__JKI_lib_State_Machine.vi"("State(s) in (\"\")"=w1476) -> ("States Out"=w1475:string)  [unwired: 14 in]
      }
      frame "LabJack: checkPedal" {
        # "Template Separator\n(You can make a copy of, or modify, this frame)"
        n664 = Unbundle By Name(w1477) -> ("LJ Pinout.Foot Pedal"=w1481:string)
        n665 = call "LabJack_FGV.vi"("Operation(Read)"=enum16{"Write", "Read"}."Read" ("Operation"), "error in (no error)"=w1479) -> ("error out"=w1483:errorcluster, "Read data"=w1484:i32)  [unwired: 8 in]
        n666 = call "LJM_eReadName.vi"("Handle In"=w1484, "Name"=w1481, "error in"=w1483) -> ("Value"=w1482:dbl, "error out"=w1480:errorcluster)  [unwired: 10 in, 1 out]
        n667 = case shown="1" w1482 {
          tunnel: w1477 -> [w1489 w1492]
          tunnel: [w1489 w1490] -> w1478
          frame 0, Default {
          }
          frame 1 {
            # "If Pedal pressed"
            n668 = Tick Count (ms)() -> (millisecond timer value=w1496:u32)
            n669 = Unbundle By Name(w1492) -> ("Last Trigger"=w1491:u32)
            n670 = Subtract(x=w1496, y=w1491) -> (x-y=w1495:u32)
            n671 = Greater Or Equal?(x=w1495, y=u32 2000) -> (x >= y?=w1493:bool)
            n672 = case shown="True" w1493 {
              tunnel: w1492 -> [w1497 w1498]
              tunnel: w1491 -> [_ _]
              tunnel: [w1497 w1499] -> w1490
              frame False {
              }
              frame True {
                n673 = Tick Count (ms)() -> (millisecond timer value=w1500:u32)
                n674 = Unbundle By Name(w1498) -> ("SysRunning?"=w1501:bool)
                n675 = case shown="False" w1501 {
                  frame False {
                    n676 = property on="StartButton" class="Bool (strict)"("Val(Sgnl)"=TRUE ("Value (Signaling)")) -> ()  [unwired: 2 in, 2 out]
                  }
                  frame True {
                    n677 = property on="StopButton" class="Bool (strict)"("Val(Sgnl)"=TRUE ("Value (Signaling)")) -> ()  [unwired: 2 in, 2 out]
                  }
                }
                n678 = Bundle By Name(cluster=w1498, "Last Trigger"=w1500) -> (w1499:T25)
              }
            }
          }
        }
        n679 = call <vilib>:"Add State(s) to Queue__JKI_lib_State_Machine.vi"("State(s) in (\"\")"=w1488) -> ("States Out"=w1487:string)  [unwired: 14 in]
      }
      frame "LabJack: ZeroV" {
        # "Just Zero V\nDO not update FGV and front panel\nWIll resume from last V"
        # "set bias to 0"
        # "Zero APD bias\n(You can make a copy of, or modify, this frame)"
        n680 = Unbundle By Name(w1506) -> ("LJ Pinout.Ch1 Bias"=w1511:string, "LJ Pinout.Ch2 Bias"=w1510:string, "LJ Pinout.Ch3 Bias"=w1509:string)
        n681 = Build Array(w1511, w1510, w1509) -> (w1508:string[])
        n682 = call "LabJack_FGV.vi"("Operation(Read)"=enum16{"Write", "Read"}."Read" ("Operation"), "error in (no error)"=w1505) -> ("error out"=w1512:errorcluster, "Read data"=w1513:i32)  [unwired: 8 in]
        n683 = call "LJM_eWriteNames.vi"("Handle In"=w1513, "aNames"=w1508, "aValuesIn"=dbl[] [0.0, 0.0, 0.0], "error in"=w1512) -> ("error out"=w1504:errorcluster)  [unwired: 9 in, 2 out]
        n684 = call <vilib>:"Add State(s) to Queue__JKI_lib_State_Machine.vi"("State(s) in (\"\")"=w1517) -> ("States Out"=w1516:string)  [unwired: 14 in]
      }
      frame "LabJack: SetV" {
        # "set bias to user specifid"
        # "Zero APD bias\n(You can make a copy of, or modify, this frame)"
        n685 = Unbundle By Name(w1531) -> ("LJ Pinout.Ch1 Bias"=w1535:string, "LJ Pinout.Ch2 Bias"=w1534:string, "LJ Pinout.Ch3 Bias"=w1533:string)
        n686 = call "V1FGV.vi"("Error In"=w1530, "action (write)"=enum16{"write", "read"}."read") -> ("Error Out"=w1529:errorcluster, "V1 out"=w1523:dbl)  [unwired: 8 in]
        n687 = local write "V 1"(w1523) -> ()
        n688 = call "V2FGV.vi"("Error In"=w1529, "action(write)"=enum16{"write", "read"}."read") -> ("Error Out"=w1528:errorcluster, "V2 out"=w1522:dbl)  [unwired: 8 in]
        n689 = local write "V 2"(w1522) -> ()
        n690 = Build Array(w1535, w1534, w1533) -> (w1532:string[])
        n691 = call "V3FGV.vi"("Error In"=w1528, "action(write)"=enum16{"write", "read"}."read" ("action(read)")) -> ("Error Out"=w1525:errorcluster, "V3 out"=w1521:dbl)  [unwired: 8 in]
        n692 = local write "V 3"(w1521) -> ()
        n693 = Build Array(w1523, w1522, w1521) -> (w1524:dbl[])
        n694 = call "LabJack_FGV.vi"("Operation(Read)"=enum16{"Write", "Read"}."Read" ("Operation"), "error in (no error)"=w1530) -> ("error out"=w1536:errorcluster, "Read data"=w1537:i32)  [unwired: 8 in]
        n695 = call "LJM_eWriteNames.vi"("Handle In"=w1537, "aNames"=w1532, "aValuesIn"=w1524, "error in"=w1536) -> ("error out"=w1526:errorcluster)  [unwired: 9 in, 2 out]
        n696 = Merge Errors(w1525, w1526) -> (w1527:errorcluster)
        n697 = call <vilib>:"Add State(s) to Queue__JKI_lib_State_Machine.vi"("State(s) in (\"\")"=w1541) -> ("States Out"=w1540:string)  [unwired: 14 in]
      }
      frame "LabJack: Open" {
        # "Initialize LabJack T7\nEstablish connection and initialize pins"
        n698 = call "LJ_Open.vi"("error in"=w1551, "DeviceType"="LJM_dtT7") -> ("error out"=w1548:errorcluster, "Success?"=w1549:bool, "Handle Out"=w1543:i32)  [unwired: 7 in]
        n699 = call "LabJack_FGV.vi"("Operation(Read)"=enum16{"Write", "Read"}."Write" ("Operation"), "error in (no error)"=w1548, "Write data"=w1543) -> ("error out"=w1545:errorcluster)  [unwired: 7 in, 1 out]
        n700 = Bundle By Name(cluster=w1546, "System Status.Labjack"=w1549) -> (w1550:T25)
        n701 = call <vilib>:"Add State(s) to Queue__JKI_lib_State_Machine.vi"("State(s) in (\"\")"=w1553) -> ("States Out"=w1552:string)  [unwired: 14 in]
      }
      frame "LabJack: SetDefaultSub" {
        w1573 = "_EF_ENABLE" ("string")
        # "1. Disable PWM\n2. Set all V to 0\n3. Set 355 relay to open\n4. Set LED to off"
        # "read once to set DIO to input"
        # "set all initila V to 0. Set footpedal to input. Set PWM to low. Set laser relay to open. Set LEDs to yellow."
        # "Set Labjack to correct input and output state and initial values"
        n702 = Unbundle By Name(w1570) -> ("LJ Pinout.355 PWM"=w1575:string, "LJ Pinout.AimingBeam PWM"=w1574:string, "LJ Pinout.Ch1 Bias"=w1582:string, "LJ Pinout.Ch2 Bias"=w1588:string, "LJ Pinout.Ch3 Bias"=w1587:string, "LJ Pinout.Laser Start/Stop"=w1586:string, "LJ Pinout.Red LED"=w1585:string, "LJ Pinout.Green LED"=w1584:string)
        n703 = call "V1FGV.vi"("Error In"=w1563, "action (write)"=enum16{"write", "read"}."write" ("action"), "V1 in"=0.0) -> ("Error Out"=w1564:errorcluster, "V1 out"=w1556:dbl)  [unwired: 7 in]
        n704 = call "LabJack_FGV.vi"("Operation(Read)"=enum16{"Write", "Read"}."Read" ("Operation"), "error in (no error)"=w1563) -> ("error out"=w1578:errorcluster, "Read data"=w1579:i32)  [unwired: 8 in]
        n705 = local write "V 1"(w1556) -> ()
        n706 = call "V2FGV.vi"("Error In"=w1564, "action(write)"=enum16{"write", "read"}."write" ("action"), "V2 in"=0.0) -> ("Error Out"=w1560:errorcluster, "V2 out"=w1555:dbl)  [unwired: 7 in]
        n707 = Concatenate Strings(w1575, w1573) -> (w1572:string)
        n708 = Concatenate Strings(w1574, w1573) -> (w1571:string)
        n709 = local write "V 2"(w1555) -> ()
        n710 = call "V3FGV.vi"("Error In"=w1560, "action(write)"=enum16{"write", "read"}."write" ("action"), "V3 in"=0.0) -> ("Error Out"=w1557:errorcluster, "V3 out"=w1554:dbl)  [unwired: 7 in]
        n711 = Build Array(w1572, w1571, w1582, w1588, w1587, w1586, w1585, w1584) -> (w1583:string[])
        n712 = local write "V 3"(w1554) -> ()
        n713 = Unbundle By Name(w1570) -> ("LJ Pinout.Foot Pedal"=w1569:string)
        n714 = call "LJM_eWriteNames.vi"("Handle In"=w1579, "aNames"=w1583, "aValuesIn"=dbl[] [0.0, 0.0, 0.0, 0.0, 0.0, 0.0, 0.0, 0.0], "error in"=w1578) -> ("Handle Out"=w1577:i32, "error out"=w1576:errorcluster)  [unwired: 9 in, 1 out]
        n715 = call "LJM_eReadName.vi"("Handle In"=w1577, "Name"=w1569, "error in"=w1576) -> ("error out"=w1559:errorcluster)  [unwired: 10 in, 2 out]
        n716 = Merge Errors(w1559, w1557) -> (w1558:errorcluster)
        n717 = call <vilib>:"Add State(s) to Queue__JKI_lib_State_Machine.vi"("State(s) in (\"\")"=w1591) -> ("States Out"=w1590:string)  [unwired: 14 in]
      }
      frame "LabJack: FootPedalConfig" {
        # "Setup footPedal\n(You can make a copy of, or modify, this frame)"
        n718 = call "LabJack_FGV.vi"("Operation(Read)"=enum16{"Write", "Read"}."Read" ("Operation"), "error in (no error)"=w1593) -> ("error out"=w1597:errorcluster, "Read data"=w1598:i32)  [unwired: 8 in]
        n719 = call "LJM_eWriteName.vi"("Handle In"=w1598, "Name"="DIO15", "Value"=1.0, "error in"=w1597) -> ("error out"=w1594:errorcluster)  [unwired: 10 in, 1 out]
        n720 = call <vilib>:"Add State(s) to Queue__JKI_lib_State_Machine.vi"("State(s) in (\"\")"=w1602) -> ("States Out"=w1601:string)  [unwired: 14 in]
      }
      frame "LabJack: SetDefaultAndClose" {
        # "Template Separator\n(You can make a copy of, or modify, this frame)"
        n721 = call <vilib>:"Add State(s) to Queue__JKI_lib_State_Machine.vi"("State(s) in Front (\"\")"="LabJack: SetDefaultSub\nLabJack: Close" ("State(s) in Front (\"\")"), "State(s) in (\"\")"=w1608) -> ("States Out"=w1607:string)  [unwired: 13 in]
      }
      frame "LabJack: Close" {
        # "Close LabJack Refnum"
        n722 = call "LabJack_FGV.vi"("Operation(Read)"=enum16{"Write", "Read"}."Read" ("Operation"), "error in (no error)"=w1614) -> ("error out"=w1609:errorcluster, "Read data"=w1610:i32)  [unwired: 8 in]
        n723 = Bundle By Name(cluster=w1612, "System Status.Labjack"=FALSE ("System Status.Gain Control")) -> (w1615:T25)
        n724 = call "LJM_Close.vi"("error in"=w1609, "Handle"=w1610) -> ("error out"=w1617:errorcluster)  [unwired: 9 in]
        n725 = call <vilib>:"Add State(s) to Queue__JKI_lib_State_Machine.vi"("State(s) in (\"\")"=w1619) -> ("States Out"=w1618:string)  [unwired: 14 in]
      }
      frame "LabJack: Interlock enable/disable" {
        w1628 = i8 0  # int8
        # "[Covers: REQ8]"
        # "Interlock enable/disable\n(Usage: \"LabJack: Interlock enable/disable >> 1|0\")"
        n726 = Fract/Exp String To Number(string=w1629, default (0 dbl)=w1628) -> (number=w1625:i8)  [unwired: 2 in, 1 out]
        n727 = Unbundle By Name(w1627) -> ("LJ Pinout.Interlock"=w1626:string)
        n728 = call "LabJack_FGV.vi"("Operation(Read)"=enum16{"Write", "Read"}."Read" ("Operation")) -> ("Read data"=w1623:i32)  [unwired: 9 in, 1 out]
        n729 = call "LJM_eWriteName.vi"("Handle In"=w1623, "Name"=w1626, "Value"=w1625, "error in"=w1624) -> ("error out"=w1621:errorcluster)  [unwired: 10 in, 1 out]
        n730 = call <vilib>:"Add State(s) to Queue__JKI_lib_State_Machine.vi"("State(s) in (\"\")"=w1631) -> ("States Out"=w1630:string)  [unwired: 14 in]
      }
      frame "LabJack: 355_PWM_Config" {
        w1633 = 0.0 ("element")
        w1653 = "DIO_EF_CLOCK1_ENABLE"
        # "Config PWM frequency"
        n731 = Unbundle By Name(w1645) -> ("LJ Pinout.355 PWM"=w1652:string)
        n732 = Unbundle By Name(w1645) -> ("355 PWM setting.DIO_EF_CLOCK1_DIVISOR"=w1644:i16, "355 PWM setting.DIO_EF_CLOCK1_ROLL_VALUE"=w1643:i32, "355 PWM setting.DIO#_EF_INDEX"=w1640:i16, "355 PWM setting.DIO#_EF_OPTIONS"=w1639:i16, "355 PWM setting.DIO#_EF_CONFIG_A"=w1638:i32)
        n733 = Concatenate Strings(w1652, "_EF_ENABLE" ("string")) -> (w1648:string)
        n734 = Concatenate Strings(w1652, "_EF_INDEX") -> (w1651:string)
        n735 = Concatenate Strings(w1652, "_EF_OPTIONS") -> (w1650:string)
        n736 = Concatenate Strings(w1652, "_EF_CONFIG_A") -> (w1649:string)
        n737 = call "LabJack_FGV.vi"("Operation(Read)"=enum16{"Write", "Read"}."Read" ("Operation")) -> ("Read data"=w1646:i32)  [unwired: 9 in, 1 out]
        n738 = Build Array(w1633, w1633, w1644, w1643, 1.0 ("element"), 0.0 ("element"), w1640, w1639, w1638) -> (w1637:dbl[])
        n739 = Build Array("DIO_EF_CLOCK0_ENABLE", w1653, "DIO_EF_CLOCK1_DIVISOR", "DIO_EF_CLOCK1_ROLL_VALUE", w1653, w1648, w1651, w1650, w1649) -> (w1647:string[])
        n740 = call "LJM_eWriteNames.vi"("Handle In"=w1646, "aNames"=w1647, "aValuesIn"=w1637, "error in"=w1635) -> ("error out"=w1636:errorcluster)  [unwired: 9 in, 2 out]
        n741 = call <vilib>:"Add State(s) to Queue__JKI_lib_State_Machine.vi"("State(s) in (\"\")"=w1662) -> ("States Out"=w1661:string)  [unwired: 14 in]
      }
      frame "LabJack: 355_PWM_Start" {
        # "Template Separator\n(You can make a copy of, or modify, this frame)"
        n742 = Unbundle By Name(w1670) -> ("LJ Pinout.355 PWM"=w1669:string)
        n743 = call "LabJack_FGV.vi"("Operation(Read)"=enum16{"Write", "Read"}."Read" ("Operation"), "error in (no error)"=w1664) -> ("error out"=w1671:errorcluster, "Read data"=w1672:i32)  [unwired: 8 in]
        n744 = Concatenate Strings(w1669, "_EF_ENABLE" ("string")) -> (w1667:string)
        n745 = call "LJM_eWriteName.vi"("Handle In"=w1672, "Name"=w1667, "Value"=1.0, "error in"=w1671) -> ("error out"=w1665:errorcluster)  [unwired: 10 in, 1 out]
        n746 = call <vilib>:"Add State(s) to Queue__JKI_lib_State_Machine.vi"("State(s) in (\"\")"=w1675) -> ("States Out"=w1674:string)  [unwired: 14 in]
      }
      frame "LabJack: 355_PWM_Stop" {
        # "Template Separator\n(You can make a copy of, or modify, this frame)"
        n747 = Unbundle By Name(w1681) -> ("LJ Pinout.355 PWM"=w1685:string)
        n748 = call "LabJack_FGV.vi"("Operation(Read)"=enum16{"Write", "Read"}."Read" ("Operation"), "error in (no error)"=w1680) -> ("error out"=w1686:errorcluster, "Read data"=w1678:i32)  [unwired: 8 in]
        n749 = Concatenate Strings(w1685, "_EF_ENABLE" ("string")) -> (w1683:string)
        n750 = call "LJM_eWriteName.vi"("Handle In"=w1678, "Name"=w1683, "Value"=0.0, "error in"=w1686) -> ("error out"=w1677:errorcluster)  [unwired: 10 in, 1 out]
        n751 = local write "355nm Laser toggle"(FALSE ("355nm Laser toggle")) -> ()
        n752 = call <vilib>:"Add State(s) to Queue__JKI_lib_State_Machine.vi"("State(s) in (\"\")"=w1689) -> ("States Out"=w1688:string)  [unwired: 14 in]
      }
      frame "LabJack: AB_Start" {
        # "Aiming Beam Start\n(Based on aimging beam frequency, set LabJack pin)"
        n753 = Unbundle By Name(w1699) -> ("AB Cluster.Freq"=w1691:i32, "LJ Pinout.AimingBeam PWM"=w1698:string)
        n754 = Greater Than 0?(x=w1691) -> (x > 0?=w1690:bool)
        n755 = case shown="False" w1690 {
          tunnel: w1698 -> [w1705 w1708]
          tunnel: [w1705 w1706] -> w1697
          frame False {
            # "if 0 freq, set PWM pin"
          }
          frame True {
            # "if non zero freq, set PWM enable"
            n756 = Concatenate Strings(w1708, "_EF_ENABLE" ("string")) -> (w1706:string)
          }
        }
        n757 = call "LabJack_FGV.vi"("Operation(Read)"=enum16{"Write", "Read"}."Read" ("Operation"), "error in (no error)"=w1694) -> ("error out"=w1700:errorcluster, "Read data"=w1701:i32)  [unwired: 8 in]
        n758 = call "LJM_eWriteName.vi"("Handle In"=w1701, "Name"=w1697, "Value"=1.0, "error in"=w1700) -> ("error out"=w1695:errorcluster)  [unwired: 10 in, 1 out]
        n759 = local write "Aiming beam toggle"(TRUE ("Aiming beam toggle")) -> ()
        n760 = call <vilib>:"Add State(s) to Queue__JKI_lib_State_Machine.vi"("State(s) in (\"\")"=w1704) -> ("States Out"=w1703:string)  [unwired: 14 in]
      }
      frame "LabJack: AB_Stop" {
        # "Aiming Beam Stop\n(Based on aiming beam frequency, set LabJack pin low)"
        n761 = Unbundle By Name(w1716) -> ("AB Cluster.Freq"=w1711:i32, "LJ Pinout.AimingBeam PWM"=w1718:string)
        n762 = Greater Than 0?(x=w1711) -> (x > 0?=w1710:bool)
        n763 = case shown="False" w1710 {
          tunnel: w1718 -> [w1724 w1727]
          tunnel: [w1724 w1725] -> w1709
          frame False {
          }
          frame True {
            n764 = Concatenate Strings(w1727, "_EF_ENABLE" ("string")) -> (w1725:string)
          }
        }
        n765 = call "LabJack_FGV.vi"("Operation(Read)"=enum16{"Write", "Read"}."Read" ("Operation"), "error in (no error)"=w1714) -> ("error out"=w1719:errorcluster, "Read data"=w1720:i32)  [unwired: 8 in]
        n766 = call "LJM_eWriteName.vi"("Handle In"=w1720, "Name"=w1709, "Value"=0.0, "error in"=w1719) -> ("error out"=w1715:errorcluster)  [unwired: 10 in, 1 out]
        n767 = local write "Aiming beam toggle"(FALSE ("Aiming beam toggle")) -> ()
        n768 = call <vilib>:"Add State(s) to Queue__JKI_lib_State_Machine.vi"("State(s) in (\"\")"=w1723) -> ("States Out"=w1722:string)  [unwired: 14 in]
      }
      frame "LabJack: AB_PWM_Config" {
        w1729 = 0.0 ("element")
        w1749 = "DIO_EF_CLOCK2_ENABLE"
        # "Config PWM frequency"
        n769 = Unbundle By Name(w1741) -> ("LJ Pinout.AimingBeam PWM"=w1748:string)
        n770 = Unbundle By Name(w1741) -> ("AB PWM setting.DIO_EF_CLOCK1_DIVISOR"=w1740:i16, "AB PWM setting.DIO_EF_CLOCK1_ROLL_VALUE"=w1739:i32, "AB PWM setting.DIO#_EF_INDEX"=w1736:i16, "AB PWM setting.DIO#_EF_OPTIONS"=w1735:i16, "AB PWM setting.DIO#_EF_CONFIG_A"=w1734:i32)
        n771 = Concatenate Strings(w1748, "_EF_ENABLE" ("string")) -> (w1744:string)
        n772 = Concatenate Strings(w1748, "_EF_INDEX") -> (w1747:string)
        n773 = Concatenate Strings(w1748, "_EF_OPTIONS") -> (w1746:string)
        n774 = Concatenate Strings(w1748, "_EF_CONFIG_A") -> (w1745:string)
        n775 = call "LabJack_FGV.vi"("Operation(Read)"=enum16{"Write", "Read"}."Read" ("Operation")) -> ("Read data"=w1742:i32)  [unwired: 9 in, 1 out]
        n776 = Build Array(w1729, w1729, w1740, w1739, 1.0 ("element"), 0.0 ("element"), w1736, w1735, w1734) -> (w1733:dbl[])
        n777 = Build Array("DIO_EF_CLOCK0_ENABLE", w1749, "DIO_EF_CLOCK2_DIVISOR", "DIO_EF_CLOCK2_ROLL_VALUE", w1749, w1744, w1747, w1746, w1745) -> (w1743:string[])
        n778 = call "LJM_eWriteNames.vi"("Handle In"=w1742, "aNames"=w1743, "aValuesIn"=w1733, "error in"=w1731) -> ("error out"=w1732:errorcluster)  [unwired: 9 in, 2 out]
        n779 = call <vilib>:"Add State(s) to Queue__JKI_lib_State_Machine.vi"("State(s) in (\"\")"=w1758) -> ("States Out"=w1757:string)  [unwired: 14 in]
      }
      frame "---------- LED ----------" {
        # "Template Separator\n(You can make a copy of, or modify, this frame)"
        n780 = call <vilib>:"Add State(s) to Queue__JKI_lib_State_Machine.vi"("State(s) in (\"\")"=w1763) -> ("States Out"=w1762:string)  [unwired: 14 in]
      }
      frame "LED: OpenVIRef" {
        # "Template Separator\n(You can make a copy of, or modify, this frame)"
        n781 = call <vilib>:"Application Directory.vi"() -> ("Application Directory"=w1770:path)
        n782 = Build Path(base path=w1770, name or relative path="SubVI") -> (appended path=w1768:path)
        n783 = Build Path(base path=w1768, name or relative path="LEDBreath.vi") -> (appended path=w1766:path)
        n784 = Open VI Reference(vi path=w1766, error in (no error)=w1771) -> (vi reference=w1772:refnum<vi>, error out=w1765:errorcluster)  [unwired: 4 in]
        n785 = case shown="Error .." w1765 {
          tunnel: [TRUE FALSE] -> w1764
          frame No Error {
          }
          frame Error {
          }
        }
        n786 = Bundle By Name(cluster=w1773, "LED vi reference"=w1772, "LED vi ref open?"=w1764) -> (w1774:T25)
        n787 = call <vilib>:"Add State(s) to Queue__JKI_lib_State_Machine.vi"("State(s) in (\"\")"=w1777) -> ("States Out"=w1776:string)  [unwired: 14 in]
      }
      frame "LED: CloseVIRef" {
        # "Template Separator\n(You can make a copy of, or modify, this frame)"
        n788 = Unbundle By Name(w1781) -> ("LED vi reference"=w1782:refnum<vi>, "LED vi ref open?"=w1780:bool)
        n789 = case shown="True" w1780 {
          tunnel: w1784 -> [w1788 w1791]
          tunnel: [w1788 w1790] -> w1783
          tunnel: w1782 -> [_ w1789]
          frame False {
          }
          frame True {
            n790 = Close Reference(reference=w1789, error in (no error)=w1791) -> (error out=w1790:errorcluster)
          }
        }
        n791 = call <vilib>:"Add State(s) to Queue__JKI_lib_State_Machine.vi"("State(s) in (\"\")"=w1787) -> ("States Out"=w1786:string)  [unwired: 14 in]
      }
      frame "LED: BreathGreen" {
        w1792 = FALSE ("Wait Until Done")
        # "Breath system LED\n(LED: Breath >> True/False)"
        n792 = Unbundle By Name(w1800) -> ("LED vi reference"=w1799:refnum<vi>)
        n793 = invoke class="VI" method="Ctrl Val.Set"(reference=w1799, error in=w1797, "Control Name"="Color", "Value"=0) -> (reference out=w1796:refnum<vi>, error out=w1795:errorcluster)  [unwired: 1 in, 3 out]
        n794 = invoke on="Invoke Node" class="VI" method="Run VI"(reference=w1796, error in=w1795, "Wait until done"=w1792, "Auto Dispose Ref"=w1792) -> (error out=w1798:errorcluster)  [unwired: 1 in, 4 out]
        n795 = call <vilib>:"Add State(s) to Queue__JKI_lib_State_Machine.vi"("State(s) in (\"\")"=w1803) -> ("States Out"=w1802:string)  [unwired: 14 in]
      }
      frame "LED: BreathOrange" {
        w1804 = FALSE ("Wait Until Done")
        # "Breath system LED\n(LED: Breath >> True/False)"
        n796 = Unbundle By Name(w1812) -> ("LED vi reference"=w1811:refnum<vi>)
        n797 = invoke class="VI" method="Ctrl Val.Set"(reference=w1811, error in=w1809, "Control Name"="Color", "Value"=1) -> (reference out=w1808:refnum<vi>, error out=w1807:errorcluster)  [unwired: 1 in, 3 out]
        n798 = invoke on="Invoke Node" class="VI" method="Run VI"(reference=w1808, error in=w1807, "Wait until done"=w1804, "Auto Dispose Ref"=w1804) -> (error out=w1810:errorcluster)  [unwired: 1 in, 4 out]
        n799 = call <vilib>:"Add State(s) to Queue__JKI_lib_State_Machine.vi"("State(s) in (\"\")"=w1815) -> ("States Out"=w1814:string)  [unwired: 14 in]
      }
      frame "LED: BreathOff" {
        # "System LED Breath Off\n(Breath off, check VI status to make sure it is off)"
        n800 = Unbundle By Name(w1824) -> ("LED vi reference"=w1823:refnum<vi>)
        n801 = invoke on="Invoke Node" class="VI" method="Ctrl Val.Set"(reference=w1823, error in=w1821, "Control Name"="Stop", "Value"=TRUE) -> (reference out=w1816:refnum<vi>, error out=w1817:errorcluster)  [unwired: 1 in, 3 out]
        n802 = case shown="No Error" w1817 {
          selector: w1817 -> [w1829 _]
          tunnel: [w1828 errorcluster {"status"=FALSE, "code"=0, "source"=""} ("error IO")] -> w1822
          tunnel: ["" ("State(s) in Front (\"\")") "LED: BreathOff" ("State(s) in Front (\"\")")] -> w1820
          tunnel: w1816 -> [w1830 _]
          frame No Error {
            # "No error, wait for VI to stop"
            n803 = while {
              tunnel: w1830 -> [w1838]
              shift-right: [w1832] -> w1828
              shift-left: w1829 -> [w1837]
              stop <- w1834 stop-if-true
              # "continue check whether vi is running"
              n804 = property class="VI"(reference=w1838, error in=w1837) -> (error out=w1832:errorcluster, "Exec.State"=w1836:T22)  [unwired: 1 out]
              n805 = Wait (ms)(milliseconds to wait=u32 50) -> ()  [unwired: 1 out]
              n806 = Equal?(x=w1836, y=T22."Idle") -> (x = y?=w1834:bool)
            }
          }
          frame Error {
            # "try again when error"
          }
        }
        n807 = call <vilib>:"Add State(s) to Queue__JKI_lib_State_Machine.vi"("State(s) in Front (\"\")"=w1820, "State(s) in (\"\")"=w1827) -> ("States Out"=w1826:string)  [unwired: 13 in]
      }
      frame "LED: Off" {
        # "set LED to red"
        # "Template Separator\n(You can make a copy of, or modify, this frame)"
        n808 = Unbundle By Name(w1843) -> ("LJ Pinout.Red LED"=w1842:string, "LJ Pinout.Green LED"=w1841:string)
        n809 = call "LabJack_FGV.vi"("Operation(Read)"=enum16{"Write", "Read"}."Read" ("Operation"), "error in (no error)"=w1844) -> ("error out"=w1851:errorcluster, "Read data"=w1850:i32)  [unwired: 8 in]
        n810 = call "LJM_eWriteName.vi"("Handle In"=w1850, "Name"=w1842, "Value"=0.0, "error in"=w1851) -> ("Handle Out"=w1848:i32, "error out"=w1847:errorcluster)  [unwired: 10 in]
        n811 = call "LJM_eWriteName.vi"("Handle In"=w1848, "Name"=w1841, "Value"=0.0, "error in"=w1847) -> ("error out"=w1845:errorcluster)  [unwired: 10 in, 1 out]
        n812 = call <vilib>:"Add State(s) to Queue__JKI_lib_State_Machine.vi"("State(s) in (\"\")"=w1855) -> ("States Out"=w1854:string)  [unwired: 14 in]
      }
      frame "LED: Green" {
        # "set LED to green"
        # "Template Separator\n(You can make a copy of, or modify, this frame)"
        n813 = Unbundle By Name(w1859) -> ("LJ Pinout.Red LED"=w1857:string, "LJ Pinout.Green LED"=w1858:string)
        n814 = call "LabJack_FGV.vi"("Operation(Read)"=enum16{"Write", "Read"}."Read" ("Operation"), "error in (no error)"=w1861) -> ("error out"=w1867:errorcluster, "Read data"=w1866:i32)  [unwired: 8 in]
        n815 = call "LJM_eWriteName.vi"("Handle In"=w1866, "Name"=w1857, "Value"=0.0, "error in"=w1867) -> ("Handle Out"=w1864:i32, "error out"=w1863:errorcluster)  [unwired: 10 in]
        n816 = call "LJM_eWriteName.vi"("Handle In"=w1864, "Name"=w1858, "Value"=9.0, "error in"=w1863) -> ("error out"=w1860:errorcluster)  [unwired: 10 in, 1 out]
        n817 = call <vilib>:"Add State(s) to Queue__JKI_lib_State_Machine.vi"("State(s) in (\"\")"=w1870) -> ("States Out"=w1869:string)  [unwired: 14 in]
      }
      frame "---------- Queue ----------" {
        # "Template Separator\n(You can make a copy of, or modify, this frame)"
        n818 = call <vilib>:"Add State(s) to Queue__JKI_lib_State_Machine.vi"("State(s) in (\"\")"=w1875) -> ("States Out"=w1874:string)  [unwired: 14 in]
      }
      frame "Queue: Flash" {
        # "Clear queue contnet\n(clear queue content by flash it)"
        n819 = Flush Queue(queue=w1881, error in (no error)=w1880) -> (error out=w1879:errorcluster)  [unwired: 2 out]
        n820 = Flush Queue(queue=w1882, error in (no error)=w1879) -> (error out=w1877:errorcluster)  [unwired: 2 out]
        n821 = Flush Queue(queue=w1878, error in (no error)=w1877) -> (error out=w1876:errorcluster)  [unwired: 2 out]
        n822 = call <vilib>:"Add State(s) to Queue__JKI_lib_State_Machine.vi"("State(s) in (\"\")"=w1886) -> ("States Out"=w1885:string)  [unwired: 14 in]
      }
      frame "Queue: Destory" {
        # "Destory Data Queue\nDistory data queue ref so the aquisition loop stop"
        n823 = Release Queue(queue=w1892, error in (no error)=w1888) -> (error out=w1895:errorcluster)  [unwired: 1 in, 2 out]
        n824 = Release Queue(queue=w1891, error in (no error)=w1888) -> (error out=w1894:errorcluster)  [unwired: 1 in, 2 out]
        n825 = Release Queue(queue=w1889, error in (no error)=w1888) -> (error out=w1887:errorcluster)  [unwired: 1 in, 2 out]
        n826 = Merge Errors(w1895, w1894, w1887) -> (w1893:errorcluster)
        n827 = call <vilib>:"Simple Error Handler.vi"("error in (no error)"=w1893) -> ()  [unwired: 4 in, 5 out]
        n828 = call <vilib>:"Add State(s) to Queue__JKI_lib_State_Machine.vi"("State(s) in (\"\")"=w1898) -> ("States Out"=w1897:string)  [unwired: 14 in]
      }
      frame "---------- Run ----------" {
        # "Template Separator\n(You can make a copy of, or modify, this frame)"
        n829 = call <vilib>:"Add State(s) to Queue__JKI_lib_State_Machine.vi"("State(s) in (\"\")"=w1903) -> ("States Out"=w1902:string)  [unwired: 14 in]
      }
      frame "Run: CaliIncrement" {
        # "Increment Calibration #\n(You can make a copy of, or modify, this frame)"
        n830 = Unbundle By Name(w1905) -> ("IDs.Cali ID"=w1907:i8)
        n831 = Increment(x=w1907) -> (x+1=w1904:i8)
        n832 = Bundle By Name(cluster=w1905, "IDs.Cali ID"=w1904) -> (w1906:T25)
        n833 = call <vilib>:"Add State(s) to Queue__JKI_lib_State_Machine.vi"("State(s) in (\"\")"=w1911) -> ("States Out"=w1910:string)  [unwired: 14 in]
      }
      frame "Run: BGIncrement" {
        # "Increment BG #\n(You can make a copy of, or modify, this frame)"
        n834 = Unbundle By Name(w1912) -> ("IDs.BG ID"=w1915:i8)
        n835 = Increment(x=w1915) -> (x+1=w1914:i8)
        n836 = Bundle By Name(cluster=w1912, "IDs.BG ID"=w1914) -> (w1913:T25)
        n837 = call <vilib>:"Add State(s) to Queue__JKI_lib_State_Machine.vi"("State(s) in (\"\")"=w1919) -> ("States Out"=w1918:string)  [unwired: 14 in]
      }
      frame "Run: Increment" {
        # "Increase Run# by 1"
        n838 = Unbundle By Name(w1924) -> ("IDs.RunID"=w1926:i8)
        n839 = Increment(x=w1926) -> (x+1=w1922:i8)
        n840 = Bundle By Name(cluster=w1924, "IDs.RunID"=w1922) -> (w1925:T25)
        n841 = call "RunIDFGV.vi"("Error In"=w1920, "RunID in"=w1922) -> ("Error Out"=w1921:errorcluster)  [unwired: 8 in, 1 out]
        n842 = call <vilib>:"Add State(s) to Queue__JKI_lib_State_Machine.vi"("State(s) in (\"\")"=w1928) -> ("States Out"=w1927:string)  [unwired: 14 in]
      }
      frame "Run: Decrement" {
        # "Increase Run# by 1"
        n843 = Unbundle By Name(w1933) -> ("IDs.RunID"=w1935:i8)
        n844 = Decrement(x=w1935) -> (x-1=w1931:i8)
        n845 = Bundle By Name(cluster=w1933, "IDs.RunID"=w1931) -> (w1934:T25)
        n846 = call "RunIDFGV.vi"("Error In"=w1929, "RunID in"=w1931) -> ("Error Out"=w1930:errorcluster)  [unwired: 8 in, 1 out]
        n847 = call <vilib>:"Add State(s) to Queue__JKI_lib_State_Machine.vi"("State(s) in (\"\")"=w1937) -> ("States Out"=w1936:string)  [unwired: 14 in]
      }
      frame "---------- SysConfig ----------" {
        # "Template Separator\n(You can make a copy of, or modify, this frame)"
        n848 = call <vilib>:"Add State(s) to Queue__JKI_lib_State_Machine.vi"("State(s) in (\"\")"=w1942) -> ("States Out"=w1941:string)  [unwired: 14 in]
      }
      frame "SysConfig: LoadAPDSerialNumber" {
        # "Template Separator\n(You can make a copy of, or modify, this frame)"
        n849 = call "readAPDSerial.vi"("Error In"=w1944) -> ("Error Out"=w1943:errorcluster, "output cluster"=w1945:T41)  [unwired: 9 in]
        n850 = Bundle By Name(cluster=w1946, "APDSerialNum"=w1945) -> (w1947:T25)
        n851 = call <vilib>:"Add State(s) to Queue__JKI_lib_State_Machine.vi"("State(s) in (\"\")"=w1950) -> ("States Out"=w1949:string)  [unwired: 14 in]
      }
      frame "SysConfig: Load Sys Config" {
        # "[Covers: REQ5]"
        # "Load System config"
        # "Load system configuration\n(Load both hardware and DAQ config)"
        n852 = call "LoadSysConfig.vi"("Error In"=w1953, "Enum"=enum16{"LastUse", "Default"}."LastUse") -> ("Error Out"=w1952:errorcluster, "SysConfigCluster"=w1955:T4)  [unwired: 8 in]
        "SysConfigCluster" <- w1955
        n853 = Bundle By Name(cluster=w1956, "SysConfigCluster"=w1955) -> (w1957:T25)
        n854 = call <vilib>:"Add State(s) to Queue__JKI_lib_State_Machine.vi"("State(s) in (\"\")"=w1959) -> ("States Out"=w1958:string)  [unwired: 14 in]
      }
      frame "SysConfig: Load Digitizer Setting" {
        w1960 = enum16{"Write", "Read"}."Write" ("Operation")
        # "Load DAQ config\nSave to FGV"
        # "Template Separator\n(You can make a copy of, or modify, this frame)"
        n855 = call <userlib>:"Current VIs Parent Directory__ogtk.vi"() -> ("Parent Directory (+ Relative)"=w1974:path)  [unwired: 5 in]
        n856 = Build Path(base path=w1974, name or relative path="SubVI\\DigitizerConfiguration\\V6_Scope_last_use.config") -> (appended path=w1975:path)
        n857 = call "ReadDigitizerConfig(SubVI).vi"("error in (no error)"=w1972, "appended path"=w1975) -> ("error out"=w1968:errorcluster, "FLImDAQ"=w1966:T6)  [unwired: 8 in]
        n858 = call "FLImDAQ_FGV.vi"("error in (no error)"=w1968, "Operation (Read)"=w1960, "Write data"=w1966) -> ("error out"=w1970:errorcluster)  [unwired: 7 in, 1 out]
        n859 = Unbundle By Name(w1966) -> ("min record length"=→"data length":i32, "Digitizer 1"=w1962:refnum<k15>, "Digitizer 2"=w1969:refnum<k15>)
        n860 = Bundle By Name(cluster=w1964, "FLImDAQ"=w1966) -> (w1965:T25)
        n861 = call "Digitizer1_FGV.vi"("error in (no error)"=w1970, "Operation (Read)"=w1960, "Write data"=w1962) -> ("error out"=w1971:errorcluster)  [unwired: 7 in, 1 out]
        n862 = call "Digitizer2_FGV.vi"("error in (no error)"=w1971, "Operation (Read)"=w1960, "Write data"=w1969) -> ("error out"=w1967:errorcluster)  [unwired: 7 in, 1 out]
        n863 = call <vilib>:"Add State(s) to Queue__JKI_lib_State_Machine.vi"("State(s) in (\"\")"=w1977) -> ("States Out"=w1976:string)  [unwired: 14 in]
      }
      frame "SysConfig: Load LJ Pinout" {
        # "Template Separator\n(You can make a copy of, or modify, this frame)"
        n864 = call <userlib>:"Current VIs Parent Directory__ogtk.vi"() -> ("Parent Directory (+ Relative)"=w1991:path)  [unwired: 5 in]
        n865 = Build Path(base path=w1991, name or relative path="SubVI\\LabJack\\LJ_pin_setting.config") -> (appended path=w1989:path)
        n866 = call "ReadLabjackConfig(SubVI).vi"("error in (no error)"=w1987, "appended path"=w1989) -> ("error out"=w1988:errorcluster, "Utility"=w1985:T5)  [unwired: 8 in]
        n867 = Unbundle By Name(w1985) -> ("Ch1 Bias"=w1984:string, "Ch2 Bias"=w1983:string, "Ch3 Bias"=w1982:string, "Red LED"=w1979:string, "Green LED"=w1978:string)
        n868 = global write "GlobalVariables.vi" "LED Green pin"(w1978) -> ()
        n869 = global write "GlobalVariables.vi" "LED Red pin"(w1979) -> ()
        n870 = global write "GlobalVariables.vi" "Ch1 LJ pin"(w1984) -> ()
        n871 = global write "GlobalVariables.vi" "Ch2 LJ pin"(w1983) -> ()
        n872 = global write "GlobalVariables.vi" "Ch3 LJ pin"(w1982) -> ()
        n873 = Bundle By Name(cluster=w1980, "LJ Pinout"=w1985) -> (w1986:T25)
        n874 = call <vilib>:"Add State(s) to Queue__JKI_lib_State_Machine.vi"("State(s) in (\"\")"=w1993) -> ("States Out"=w1992:string)  [unwired: 14 in]
      }
      frame "SysConfig: Load 355 PWM" {
        # "Template Separator\n(You can make a copy of, or modify, this frame)"
        n875 = call <userlib>:"Current VIs Parent Directory__ogtk.vi"() -> ("Parent Directory (+ Relative)"=w2011:path)  [unwired: 5 in]
        n876 = Build Path(base path=w2011, name or relative path="SubVI\\LabJack\\PWM_setting_355.config") -> (appended path=w2009:path)
        n877 = call "ReadPWMConfig(SubVI).vi"("error in (no error)"=w2006, "appended path"=w2009) -> ("error out"=w2007:errorcluster, "PWM Setting"=w2005:T42)  [unwired: 8 in]
        n878 = Unbundle By Name(w2005) -> ("DIO_EF_CLOCK1_DIVISOR"=w2002:i16, "DIO_EF_CLOCK1_ROLL_VALUE"=w2001:i32)
        n879 = Multiply(x=w2002, y=w2001) -> (x*y=w2003:i32)
        n880 = Bundle By Name(cluster=w2008, "355 PWM setting"=w2005) -> (w1995:T25)
        n881 = Divide(x=80000000.0, y=w2003) -> (x/y=w2000:dbl)
        "Laser Rep Rate" <- w2000
        n882 = Number To Decimal String(number=w2000) -> (decimal integer string=w1999:string)  [unwired: 1 in]
        n883 = Concatenate Strings("355nm " ("string"), w1999, "Hz" ("string")) -> (w1997:string)
        n884 = property on="355nm Laser toggle" class="Bool (strict)"("Caption.Text"=w1997) -> ()  [unwired: 2 in, 2 out]
        n885 = call <vilib>:"Add State(s) to Queue__JKI_lib_State_Machine.vi"("State(s) in (\"\")"=w2013) -> ("States Out"=w2012:string)  [unwired: 14 in]
      }
      frame "SysConfig: Load AB PWM" {
        # "Template Separator\n(You can make a copy of, or modify, this frame)"
        n886 = call <userlib>:"Current VIs Parent Directory__ogtk.vi"() -> ("Parent Directory (+ Relative)"=w2022:path)  [unwired: 5 in]
        n887 = Build Path(base path=w2022, name or relative path="SubVI\\LabJack\\PWM_setting_AB.config") -> (appended path=w2020:path)
        n888 = call "ReadPWMConfig(SubVI).vi"("error in (no error)"=w2017, "appended path"=w2020) -> ("error out"=w2018:errorcluster, "PWM Setting"=w2016:T42)  [unwired: 8 in]
        n889 = Bundle By Name(cluster=w2014, "AB PWM setting"=w2016) -> (w2019:T25)
        n890 = call <vilib>:"Add State(s) to Queue__JKI_lib_State_Machine.vi"("State(s) in (\"\")"=w2024) -> ("States Out"=w2023:string)  [unwired: 14 in]
      }
      frame "SysConfig: Load AB setting" {
        # "load aming beam setting\n(check frequency, if 0 do nothing, if not zero, config PWM)"
        n891 = call "readAimingBeamSetting.vi"("error in (no error)"=w2042) -> ("error out"=w2037:errorcluster, "Aiming Beam Setting"=w2029:T43)  [unwired: 9 in]
        n892 = Unbundle By Name(w2029) -> ("Default Current"=w2028:dbl)
        n893 = Unbundle By Name(w2029) -> ("Frequency(Hz)"=w2025:u32)
        n894 = Equal To 0?(x=w2025) -> (x = 0?=w2035:bool)
        n895 = Select(t="", s=w2035, f="SysConfig: Load AB PWM" ("State(s) in Front (\"\")")) -> (s? t:f=w2038:string)
        n896 = Number To Decimal String(number=w2025) -> (decimal integer string=w2034:string)  [unwired: 1 in]
        n897 = Number To Decimal String(number=w2028, width (-)=i16 2) -> (decimal integer string=w2027:string)
        n898 = Concatenate Strings("445nm " ("string"), w2034, "Hz " ("string"), w2027, "mA" ("string")) -> (w2033:string)
        n899 = property on="Aiming beam toggle" class="Bool (strict)"("Caption.Text"=w2033) -> ()  [unwired: 2 in, 2 out]
        n900 = case shown="False" w2035 {
          tunnel: w2037 -> [w2050 w2053]
          tunnel: [w2049 w2053] -> w2036
          tunnel: w2025 -> [w2048 _]
          frame False {
            n901 = call "LJ_calculate_PWM_parameters.vi"("Duty Cycle (%)"=u32 10, "Error In"=w2050, "Show Confirmation"=FALSE, "Laser Rep Rate (Hz)"=w2048, "Laser"=enum16{"355nm", "AimingBeam"}."AimingBeam") -> ("Error Out"=w2049:errorcluster)  [unwired: 5 in, 1 out]
          }
          frame True {
          }
        }
        n902 = Bundle By Name(cluster=w2043, "AB Cluster"=w2029) -> (w2044:T25)
        n903 = call <vilib>:"Add State(s) to Queue__JKI_lib_State_Machine.vi"("State(s) in Front (\"\")"=w2038, "State(s) in (\"\")"=w2046) -> ("States Out"=w2045:string)  [unwired: 13 in]
      }
      frame "SysConfig: LoadABVideoSetting" {
        # "Load AB video setting form ini file\n()"
        n904 = call "readVideoConfig.vi"("error in (no error)"=w2057) -> ("error out"=w2058:errorcluster, "Aiming Beam Config"=w2056:T24)  [unwired: 8 in, 1 out]
        n905 = Bundle By Name(cluster=w2054, "VideoConfig"=w2056) -> (w2055:T25)
        n906 = call <vilib>:"Add State(s) to Queue__JKI_lib_State_Machine.vi"("State(s) in (\"\")"=w2061) -> ("States Out"=w2060:string)  [unwired: 14 in]
      }
      frame "SysConfig: LoadCursorLocation" {
        # "Load cursor location from ini file\n(load cursor from system setting ini file)"
        n907 = call "readCursorConfigMain.vi"("error in (no error)"=w2073) -> ("error out"=w2074:errorcluster, "Cursor Locations"=w2072:T44)  [unwired: 9 in]
        n908 = Unbundle By Name(w2072) -> ("DC1"=w2071:i32, "DC2"=w2070:i32, "BG1"=w2065:i32, "BG2"=w2064:i32)
        n909 = Build Array(w2071, w2070) -> (w2069:i32[])
        n910 = Build Array(w2065, w2064) -> (w2066:i32[])
        n911 = Array Max & Min(array=w2069) -> (max value=w2068:i32, min value=w2067:i32)  [unwired: 2 out]
        n912 = Array Max & Min(array=w2066) -> (max value=w2063:i32, min value=w2062:i32)  [unwired: 2 out]
        n913 = global write "GlobalVariables.vi" "DC Idx2"(w2068) -> ()
        n914 = global write "GlobalVariables.vi" "DC Idx1"(w2067) -> ()
        n915 = global write "GlobalVariables.vi" "BG Idx2"(w2063) -> ()
        n916 = global write "GlobalVariables.vi" "BG Idx1"(w2062) -> ()
        n917 = call <vilib>:"Add State(s) to Queue__JKI_lib_State_Machine.vi"("State(s) in (\"\")"=w2078) -> ("States Out"=w2077:string)  [unwired: 14 in]
      }
      frame "---------- SystemStatus ----------" {
        # "Template Separator\n(You can make a copy of, or modify, this frame)"
        n918 = call <vilib>:"Add State(s) to Queue__JKI_lib_State_Machine.vi"("State(s) in (\"\")"=w2083) -> ("States Out"=w2082:string)  [unwired: 14 in]
      }
      frame "SystemStatus: SlowSysStatusMacro" {
        # "store system check time"
        # "Template Separator\n(You can make a copy of, or modify, this frame)"
        n919 = Tick Count (ms)() -> (millisecond timer value=w2086:u32)
        n920 = Bundle By Name(cluster=w2084, "SlowTimer"=w2086) -> (w2085:T25)
        n921 = call <vilib>:"Add State(s) to Queue__JKI_lib_State_Machine.vi"("State(s) in Front (\"\")"="Digitizer: checkTemp\nTCP: CheckConnection" ("State(s) in Front (\"\")"), "State(s) in (\"\")"=w2091) -> ("States Out"=w2090:string)  [unwired: 13 in]
      }
      frame "SystemStatus: FastSysStatusMacro" {
        # "store system check time"
        # "Template Separator\n(You can make a copy of, or modify, this frame)"
        n922 = Tick Count (ms)() -> (millisecond timer value=w2094:u32)
        n923 = Bundle By Name(cluster=w2092, "FastTimer"=w2094) -> (w2093:T25)
        n924 = call <vilib>:"Add State(s) to Queue__JKI_lib_State_Machine.vi"("State(s) in Front (\"\")"="355 Laser: CheckPWMStatus\nAimingBeam: GetPWMStatus\n/*355 Laser: CheckControllerStatus" ("State(s) in Front (\"\")"), "State(s) in (\"\")"=w2099) -> ("States Out"=w2098:string)  [unwired: 13 in]
      }
      frame "---------- UI ----------" {
        # "Do not put any code in this frame.\n(It is a separator no-op. You can make a copy of this frame to create a new UI frame)"
        n925 = call <vilib>:"Add State(s) to Queue__JKI_lib_State_Machine.vi"("State(s) in (\"\")"=w2104) -> ("States Out"=w2103:string)  [unwired: 14 in]
      }
      frame "UI: Initialize" {
        w2106 = T45 {"Minimum"=0.0, "Maximum"=4.6, "Increment"=0.1} ("Data Entry Limits")
        w2105 = T10."Disabled and Grayed Out" ("Disabled")
        # "Disable all button on startup"
        # "Initialize the User Interface, here.\n(this is called automatically, by the Macro: Init)"
        n926 = property on="V 1" class="DigNum (strict)"("DisabledEnum"=w2105) -> ()  [unwired: 2 in, 2 out]
        n927 = property on="V 2" class="DigNum (strict)"("DisabledEnum"=w2105) -> ()  [unwired: 2 in, 2 out]
        n928 = property on="StopButton" class="Bool (strict)"("DisabledEnum"=w2105) -> ()  [unwired: 2 in, 2 out]
        n929 = property on="Sys Reconfig" class="Bool"("DisabledEnum"=w2105) -> ()  [unwired: 2 in, 2 out]
        n930 = property on="StartButton" class="Bool (strict)"("DisabledEnum"=w2105) -> ()  [unwired: 2 in, 2 out]
        n931 = property on="355nm Laser toggle" class="Bool (strict)"("DisabledEnum"=w2105) -> ()  [unwired: 2 in, 2 out]
        n932 = property on="Aiming beam toggle" class="Bool (strict)"("DisabledEnum"=w2105) -> ()  [unwired: 2 in, 2 out]
        n933 = property on="Background" class="Bool (strict)"("DisabledEnum"=w2105) -> ()  [unwired: 2 in, 2 out]
        n934 = property on="Cali&iRF alignment" class="Bool (strict)"("DisabledEnum"=w2105) -> ()  [unwired: 2 in, 2 out]
        n935 = property on="V 3" class="DigNum (strict)"("DisabledEnum"=w2105) -> ()  [unwired: 2 in, 2 out]
        n936 = property on="Video Source" class="RadioBtnsControl (strict)"("DisabledEnum"=w2105) -> ()  [unwired: 2 in, 2 out]
        n937 = property on="V 1" class="DigNum (strict)"("Data Range"=w2106) -> ()  [unwired: 2 in, 2 out]
        n938 = property on="V 2" class="DigNum (strict)"("Data Range"=w2106) -> ()  [unwired: 2 in, 2 out]
        n939 = property on="V 3" class="DigNum (strict)"("Data Range"=w2106) -> ()  [unwired: 2 in, 2 out]
        n940 = call <vilib>:"Add State(s) to Queue__JKI_lib_State_Machine.vi"("State(s) in Front (\"\")"="UI: CaliAndiRFNotReady" ("State(s) in Front (\"\")"), "State(s) in (\"\")"=w2112) -> ("States Out"=w2111:string)  [unwired: 13 in]
      }
      frame "UI: BGLoaded" {
        # "[Covers: REQ24]"
        # "Do not put any code in this frame.\n(It is a separator no-op. You can make a copy of this frame to create a new UI frame)"
        n941 = property on="Background" class="Bool (strict)"("BoolText.Text"="Loaded!" ("Boolean Text.Text"), "Colors [4]"=cluster{u32, u32}[] [{15764023, 15764023}, {16711680, 16711680}]) -> ()  [unwired: 2 in, 2 out]
        n942 = call <vilib>:"Add State(s) to Queue__JKI_lib_State_Machine.vi"("State(s) in (\"\")"=w2119) -> ("States Out"=w2118:string)  [unwired: 14 in]
      }
      frame "UI: BGSizeError" {
        # "[Covers: REQ24]"
        # "Do not put any code in this frame.\n(It is a separator no-op. You can make a copy of this frame to create a new UI frame)"
        n943 = property on="Background" class="Bool (strict)"("BoolText.Text"="Loaded!" ("Boolean Text.Text"), "Colors [4]"=cluster{u32, u32}[] [{7171459, 7171459}, {16711680, 16711680}]) -> ()  [unwired: 2 in, 2 out]
        n944 = One Button Dialog(message="Background waveform length and current digitizer setting mismatch! Please take a new background before any aquisition!") -> ()  [unwired: 1 in, 1 out]
        n945 = call <vilib>:"Add State(s) to Queue__JKI_lib_State_Machine.vi"("State(s) in (\"\")"=w2127) -> ("States Out"=w2126:string)  [unwired: 14 in]
      }
      frame "UI: CaliAndiRFLoaded" {
        # "[Covers: REQ24]"
        # "Do not put any code in this frame.\n(It is a separator no-op. You can make a copy of this frame to create a new UI frame)"
        n946 = property on="Cali&iRF alignment" class="Bool (strict)"("BoolText.Text"="Loaded!" ("Boolean Text.Text"), "Colors [4]"=cluster{u32, u32}[] [{15764023, 15764023}, {16711680, 16711680}]) -> ()  [unwired: 2 in, 2 out]
        n947 = call <vilib>:"Add State(s) to Queue__JKI_lib_State_Machine.vi"("State(s) in (\"\")"=w2134) -> ("States Out"=w2133:string)  [unwired: 14 in]
      }
      frame "UI: WFAutoScale" {
        # "Set graph auto scale.\n(UI: WFAutoScale >> T/F)"
        n948 = Equal?(x=w2135, y="F") -> (x = y?=w2136:bool)
        n949 = Equal?(x=w2135, y="T") -> (x = y?=w2138:bool)
        n950 = case shown="True" w2138 {
          frame False {
          }
          frame True {
            w2154 = u8 2 ("Y Scale.Scale Fit")
            n951 = property on="Channel 1" class="WFGraph (strict)"("YScale.ScaleFit"=w2154) -> ()  [unwired: 2 in, 2 out]
            n952 = property on="Channel 2" class="WFGraph (strict)"("YScale.ScaleFit"=w2154) -> ()  [unwired: 2 in, 2 out]
            n953 = property on="Channel 3" class="WFGraph (strict)"("YScale.ScaleFit"=w2154) -> ()  [unwired: 2 in, 2 out]
          }
        }
        n954 = case shown="True" w2136 {
          frame False {
          }
          frame True {
            w2151 = 0.0 ("Y Scale.Range:Maximum")
            w2152 = 2.0 ("Y Scale.Range:Maximum")
            w2153 = u8 0 ("Y Scale.Scale Fit")
            n955 = property on="Channel 1" class="WFGraph (strict)"("YScale.ScaleFit"=w2153) -> (error out=w2150:errorcluster)  [unwired: 2 in, 1 out]
            n956 = property on="Channel 2" class="WFGraph (strict)"("YScale.ScaleFit"=w2153) -> (error out=w2149:errorcluster)  [unwired: 2 in, 1 out]
            n957 = property on="Channel 3" class="WFGraph (strict)"("YScale.ScaleFit"=w2153) -> (error out=w2148:errorcluster)  [unwired: 2 in, 1 out]
            n958 = property on="Channel 1" class="WFGraph (strict)"(error in=w2150, "YScale.Maximum"=w2152) -> (error out=w2147:errorcluster)  [unwired: 1 in, 1 out]
            n959 = property on="Channel 2" class="WFGraph (strict)"(error in=w2149, "YScale.Maximum"=w2152) -> (error out=w2146:errorcluster)  [unwired: 1 in, 1 out]
            n960 = property on="Channel 3" class="WFGraph (strict)"(error in=w2148, "YScale.Maximum"=w2152) -> (error out=w2145:errorcluster)  [unwired: 1 in, 1 out]
            n961 = property on="Channel 1" class="WFGraph (strict)"(error in=w2147, "YScale.Minimum"=w2151) -> ()  [unwired: 1 in, 2 out]
            n962 = property on="Channel 2" class="WFGraph (strict)"(error in=w2146, "YScale.Minimum"=w2151) -> ()  [unwired: 1 in, 2 out]
            n963 = property on="Channel 3" class="WFGraph (strict)"(error in=w2145, "YScale.Minimum"=w2151) -> ()  [unwired: 1 in, 2 out]
          }
        }
        n964 = call <vilib>:"Add State(s) to Queue__JKI_lib_State_Machine.vi"("State(s) in (\"\")"=w2144) -> ("States Out"=w2143:string)  [unwired: 14 in]
      }
      frame "UI: showDisclaimer" {
        # "Show disclamer window.\n(It is a separator no-op. You can make a copy of this frame to create a new UI frame)"
        n965 = call <vilib>:"Application Directory.vi"() -> ("Application Directory"=w2167:path)
        n966 = Build Path(base path=w2167, name or relative path="Disclamer.png") -> (appended path=w2165:path)
        n967 = property on="Disclamer" class="Pict"() -> ("Draw Area Size"=w2163:T46)  [unwired: 2 in, 2 out]
        n968 = disable-structure "Diagram Disable Structure" shown="Disabled" {
          frame Disabled {
            n969 = flat-sequence {
              frame #0 {
                n970 = call "disclaimer.vi"() -> ()  [unwired: 12 in]
              }
              frame #1 {
                n971 = Wait (ms)(milliseconds to wait=u32 250) -> ()  [unwired: 1 out]
              }
              frame #2 {
                n972 = call "SoftwareNote.vi"() -> ()  [unwired: 12 in]
              }
            }
          }
          frame Enabled {
          }
        }
        n973 = call <vilib>:"Read PNG File.vi"("path to PNG file"=w2165) -> ("image data"=w2162:T47)  [unwired: 8 in, 2 out]
        n974 = Unbundle By Name(w2162) -> ("Rectangle.right"=w2160:i16, "Rectangle.bottom"=w2158:i16)
        n975 = Unbundle By Name(w2163) -> ("Width"=w2161:u32, "Height"=w2159:u32)
        n976 = call <vilib>:"Draw Flattened Pixmap.vi"("image data"=w2162) -> ("new picture"=→"Disclamer":picture)  [unwired: 8 in]
        n977 = Divide(x=w2161, y=w2160) -> (x/y=w2157:dbl)
        n978 = Divide(x=w2159, y=w2158) -> (x/y=w2156:dbl)
        n979 = Max & Min(x=w2157, y=w2156) -> (min(x,y)=w2155:dbl)  [unwired: 1 out]
        n980 = property on="Disclamer" class="Pict"("ZoomFactor"=w2155) -> ()  [unwired: 2 in, 2 out]
        n981 = call <vilib>:"Add State(s) to Queue__JKI_lib_State_Machine.vi"("State(s) in (\"\")"=w2172) -> ("States Out"=w2171:string)  [unwired: 14 in]
      }
      frame "UI: CaliAndiRFNotReady" {
        # "Do not put any code in this frame.\n(It is a separator no-op. You can make a copy of this frame to create a new UI frame)"
        n982 = property on="Cali&iRF alignment" class="Bool (strict)"("BoolText.Text"="No Info" ("Boolean Text.Text"), "Colors [4]"=cluster{u32, u32}[] [{13816530, 13816530}, {16711680, 16711680}]) -> ()  [unwired: 2 in, 2 out]
        n983 = call <vilib>:"Add State(s) to Queue__JKI_lib_State_Machine.vi"("State(s) in (\"\")"=w2180) -> ("States Out"=w2179:string)  [unwired: 14 in]
      }
      frame "UI: BGnotReady" {
        # "Do not put any code in this frame.\n(It is a separator no-op. You can make a copy of this frame to create a new UI frame)"
        n984 = property on="Background" class="Bool (strict)"("BoolText.Text"="No Info" ("Boolean Text.Text"), "Colors [4]"=cluster{u32, u32}[] [{13816530, 13816530}, {16711680, 16711680}]) -> ()  [unwired: 2 in, 2 out]
        n985 = call <vilib>:"Add State(s) to Queue__JKI_lib_State_Machine.vi"("State(s) in (\"\")"=w2187) -> ("States Out"=w2186:string)  [unwired: 14 in]
      }
      frame "UI: Reset" {
        w2189 = cluster{u32, u32}[] [{13816530, 13816530}, {13816530, 13816530}] ("Colors [4]")
        # "Do not put any code in this frame.\n(It is a separator no-op. You can make a copy of this frame to create a new UI frame)"
        n986 = property on="Cali&iRF alignment" class="Bool (strict)"("BoolText.Text"="No Info" ("Boolean Text.Text"), "Colors [4]"=w2189) -> ()  [unwired: 2 in, 2 out]
        n987 = property on="Background" class="Bool (strict)"("BoolText.Text"="No Info" ("Boolean Text.Text"), "Colors [4]"=w2189) -> ()  [unwired: 2 in, 2 out]
        n988 = call <vilib>:"Add State(s) to Queue__JKI_lib_State_Machine.vi"("State(s) in (\"\")"=w2195) -> ("States Out"=w2194:string)  [unwired: 14 in]
      }
      frame "UI: SetButtonText" {
        # "Set button text of 355nm laser and aiming beam."
        n989 = call <vilib>:"Add State(s) to Queue__JKI_lib_State_Machine.vi"("State(s) in (\"\")"=w2200) -> ("States Out"=w2199:string)  [unwired: 14 in]
      }
      frame "UI: DuringAquisition" {
        w2203 = T10."Disabled and Grayed Out" ("Disabled")
        # "Do not put any code in this frame.\n(It is a separator no-op. You can make a copy of this frame to create a new UI frame)"
        n990 = Unbundle By Name(w2202) -> ("bothVidSourceAvail"=w2201:bool)
        n991 = case shown="True" w2201 {
          tunnel: w2203 -> [_ w2209]
          frame False {
          }
          frame True {
            n992 = property on="Video Source" class="RadioBtnsControl (strict)"("DisabledEnum"=w2209) -> ()  [unwired: 2 in, 2 out]
          }
        }
        n993 = property on="StartButton" class="Bool (strict)"("DisabledEnum"=w2203) -> ()  [unwired: 2 in, 2 out]
        n994 = property on="Sys Reconfig" class="Bool"("DisabledEnum"=w2203) -> ()  [unwired: 2 in, 2 out]
        n995 = property on="355nm Laser toggle" class="Bool (strict)"("DisabledEnum"=w2203) -> ()  [unwired: 2 in, 2 out]
        n996 = property on="Aiming beam toggle" class="Bool (strict)"("DisabledEnum"=w2203) -> ()  [unwired: 2 in, 2 out]
        n997 = property on="Background" class="Bool (strict)"("DisabledEnum"=w2203) -> ()  [unwired: 2 in, 2 out]
        n998 = property on="Radio Buttons" class="RadioBtnsControl (strict)"("DisabledEnum"=w2203) -> ()  [unwired: 2 in, 2 out]
        n999 = property on="Cali&iRF alignment" class="Bool (strict)"("DisabledEnum"=w2203) -> ()  [unwired: 2 in, 2 out]
        n1000 = property on="Quit" class="Bool"("DisabledEnum"=w2203) -> ()  [unwired: 2 in, 2 out]
        n1001 = property on="Skip Data Save?" class="Bool (strict)"("DisabledEnum"=w2203) -> ()  [unwired: 2 in, 2 out]
        n1002 = property on="Video Display" class="Bool (strict)"("DisabledEnum"=w2203) -> ()  [unwired: 2 in, 2 out]
        n1003 = property on="StopButton" class="Bool (strict)"("DisabledEnum"=T10."Enabled" ("Disabled")) -> ()  [unwired: 2 in, 2 out]
        n1004 = call <vilib>:"Add State(s) to Queue__JKI_lib_State_Machine.vi"("State(s) in (\"\")"=w2208) -> ("States Out"=w2207:string)  [unwired: 14 in]
      }
      frame "UI: duringIRFAlign" {
        w2210 = T10."Disabled and Grayed Out" ("Disabled")
        # "Set UI to during iRF alignment\n(It is a separator no-op. You can make a copy of this frame to create a new UI frame)"
        n1005 = property on="StartButton" class="Bool (strict)"("DisabledEnum"=w2210) -> ()  [unwired: 2 in, 2 out]
        n1006 = property on="Sys Reconfig" class="Bool"("DisabledEnum"=w2210) -> ()  [unwired: 2 in, 2 out]
        n1007 = property on="355nm Laser toggle" class="Bool (strict)"("DisabledEnum"=w2210) -> ()  [unwired: 2 in, 2 out]
        n1008 = property on="Aiming beam toggle" class="Bool (strict)"("DisabledEnum"=w2210) -> ()  [unwired: 2 in, 2 out]
        n1009 = property on="Background" class="Bool (strict)"("DisabledEnum"=w2210) -> ()  [unwired: 2 in, 2 out]
        n1010 = property on="StopButton" class="Bool (strict)"("DisabledEnum"=w2210) -> ()  [unwired: 2 in, 2 out]
        n1011 = call <vilib>:"Add State(s) to Queue__JKI_lib_State_Machine.vi"("State(s) in (\"\")"=w2215) -> ("States Out"=w2214:string)  [unwired: 14 in]
      }
      frame "UI: duringBGAcquire" {
        w2216 = T10."Disabled and Grayed Out" ("Disabled")
        # "Do not put any code in this frame.\n(It is a separator no-op. You can make a copy of this frame to create a new UI frame)"
        n1012 = property on="StartButton" class="Bool (strict)"("DisabledEnum"=w2216) -> ()  [unwired: 2 in, 2 out]
        n1013 = property on="StopButton" class="Bool (strict)"("DisabledEnum"=w2216) -> ()  [unwired: 2 in, 2 out]
        n1014 = property on="Sys Reconfig" class="Bool"("DisabledEnum"=w2216) -> ()  [unwired: 2 in, 2 out]
        n1015 = property on="355nm Laser toggle" class="Bool (strict)"("DisabledEnum"=w2216) -> ()  [unwired: 2 in, 2 out]
        n1016 = property on="Aiming beam toggle" class="Bool (strict)"("DisabledEnum"=w2216) -> ()  [unwired: 2 in, 2 out]
        n1017 = property on="Cali&iRF alignment" class="Bool (strict)"("DisabledEnum"=w2216) -> ()  [unwired: 2 in, 2 out]
        n1018 = call <vilib>:"Add State(s) to Queue__JKI_lib_State_Machine.vi"("State(s) in (\"\")"=w2221) -> ("States Out"=w2220:string)  [unwired: 14 in]
      }
      frame "UI: ReadyForAquisition" {
        w2225 = T10."Enabled" ("Disabled")
        # "Do not put any code in this frame.\n(It is a separator no-op. You can make a copy of this frame to create a new UI frame)"
        n1019 = Unbundle By Name(w2224) -> ("System Status.TCP/IP"=w2223:bool, "bothVidSourceAvail"=w2222:bool)
        n1020 = property on="StartButton" class="Bool (strict)"("DisabledEnum"=w2225) -> ()  [unwired: 2 in, 2 out]
        n1021 = property on="Sys Reconfig" class="Bool"("DisabledEnum"=w2225) -> ()  [unwired: 2 in, 2 out]
        n1022 = property on="355nm Laser toggle" class="Bool (strict)"("DisabledEnum"=w2225) -> ()  [unwired: 2 in, 2 out]
        n1023 = property on="Aiming beam toggle" class="Bool (strict)"("DisabledEnum"=w2225) -> ()  [unwired: 2 in, 2 out]
        n1024 = property on="Cali&iRF alignment" class="Bool (strict)"("DisabledEnum"=w2225) -> ()  [unwired: 2 in, 2 out]
        n1025 = property on="Background" class="Bool (strict)"("DisabledEnum"=w2225) -> ()  [unwired: 2 in, 2 out]
        n1026 = property on="Quit" class="Bool"("DisabledEnum"=w2225) -> ()  [unwired: 2 in, 2 out]
        n1027 = property on="Radio Buttons" class="RadioBtnsControl (strict)"("DisabledEnum"=w2225) -> ()  [unwired: 2 in, 2 out]
        n1028 = case shown="True" w2222 {
          tunnel: w2225 -> [_ w2231]
          frame False {
          }
          frame True {
            n1029 = property on="Video Source" class="RadioBtnsControl (strict)"("DisabledEnum"=w2231) -> ()  [unwired: 2 in, 2 out]
          }
        }
        n1030 = property on="Skip Data Save?" class="Bool (strict)"("DisabledEnum"=w2225) -> ()  [unwired: 2 in, 2 out]
        n1031 = case shown="True" w2223 {
          tunnel: w2225 -> [_ w2232]
          frame False {
          }
          frame True {
            n1032 = property on="Video Display" class="Bool (strict)"("DisabledEnum"=w2232) -> ()  [unwired: 2 in, 2 out]
          }
        }
        n1033 = property on="StopButton" class="Bool (strict)"("DisabledEnum"=T10."Disabled and Grayed Out" ("Disabled")) -> ()  [unwired: 2 in, 2 out]
        n1034 = call <vilib>:"Add State(s) to Queue__JKI_lib_State_Machine.vi"("State(s) in (\"\")"=w2230) -> ("States Out"=w2229:string)  [unwired: 14 in]
      }
      frame "UI: Update" {
        # "Do not put any code in this frame.\n(It is a separator no-op. You can make a copy of this frame to create a new UI frame)"
        n1035 = Unbundle By Name(w2243) -> ("System Status"=→"System Hardware Connection Status":T2, "IDs.RunID"=→"Run #":i8, "CaseID"=→"Case #":string, "FLImDAQ"=→"FLImDAQ":T32, "SysRunning?"=→"Aquisition Status:":bool, "LJ Pinout"=→"LJ Pinout":T5, "IDs.BG ID"=→"BG #":i8, "IDs.Cali ID"=→"Calibration #":i8, "video source"=→"Visualization PC video source":T1)
        n1036 = call <vilib>:"Add State(s) to Queue__JKI_lib_State_Machine.vi"("State(s) in (\"\")"=w2246) -> ("States Out"=w2245:string)  [unwired: 14 in]
      }
      frame "UI: updateVideoToggle" {
        # "Set video toggle based on visualization PC video source.\n(take )"
        n1037 = call <vilib>:"Add State(s) to Queue__JKI_lib_State_Machine.vi"("State(s) in (\"\")"=w2251) -> ("States Out"=w2250:string)  [unwired: 14 in]
      }
      frame "UI: Cursor Set" {
        # "Argument"
        # "Set and Unset Cursor Busy.\n(Usage: \"UI: Cursor Set >> Busy|Idle\")"
        n1038 = case shown="\"Idle\", Default" w2253 {
          tunnel: w2255 -> [w2260 w2262]
          tunnel: [w2259 w2261] -> w2254
          frame "Idle", Default {
            n1039 = call <vilib>:"Unset Busy.vi"("error in (no error)"=w2260) -> ("error out"=w2259:errorcluster)  [unwired: 10 in]
          }
          frame "Busy" {
            n1040 = call <vilib>:"Set Busy.vi"("error in (no error)"=w2262) -> ("error out"=w2261:errorcluster)  [unwired: 9 in, 1 out]
          }
        }
        n1041 = call <vilib>:"Add State(s) to Queue__JKI_lib_State_Machine.vi"("State(s) in (\"\")"=w2258) -> ("States Out"=w2257:string)  [unwired: 14 in]
      }
      frame "UI: Front Panel State" {
        # "Argument"
        # "Set Front Panel Open or Closed\n(Usage: \"UI: Front Panel State >> Open|Close\")"
        n1042 = Unbundle By Name(w2266) -> ("Core.Current VI Reference"=w2265:refnum<vi>)
        n1043 = case shown="\"Open\", \"Standard\", Default" w2264 {
          tunnel: w2268 -> [w2276 w2291 w2302 w2315 w2328]
          tunnel: [w2278 w2292 w2304 w2317 w2330] -> w2267
          tunnel: w2265 -> [w2277 w2289 w2303 w2316 w2329]
          frame "Open", "Standard", Default {
            w2271 = T20."Standard" ("State")
            n1044 = property on="Property Node" class="VI"(reference=w2277, error in=w2276) -> (reference out=w2274:refnum<vi>, error out=w2275:errorcluster, "FP.State"=w2273:T20)
            n1045 = Not Equal?(x=w2273, y=w2271) -> (x != y?=w2272:bool)
            n1046 = case shown="True" w2272 {
              tunnel: [w2282 w2284] -> w2278
              tunnel: w2275 -> [w2281 w2284]
              tunnel: w2274 -> [w2280 _]
              tunnel: w2271 -> [w2279 _]
              frame True {
                n1047 = invoke on="Invoke Node" class="VI" method="FP.Open"(reference=w2280, error in=w2281, "Activate"=TRUE, "State"=w2279) -> (error out=w2282:errorcluster)  [unwired: 1 in, 4 out]
              }
              frame False {
              }
            }
          }
          frame "Close", "Closed" {
            n1048 = property on="Property Node" class="VI"(reference=w2289, error in=w2291) -> (reference out=w2288:refnum<vi>, error out=w2290:errorcluster, "FP.State"=w2286:T20)
            n1049 = Not Equal?(x=w2286, y=T20."Closed" ("Front Panel Window:State")) -> (x != y?=w2285:bool)
            n1050 = case shown="True" w2285 {
              tunnel: [w2293 w2296] -> w2292
              tunnel: w2290 -> [w2293 w2295]
              tunnel: w2288 -> [_ w2294]
              frame False {
              }
              frame True {
                n1051 = invoke on="Invoke Node" class="VI" method="FP.Close"(reference=w2294, error in=w2295) -> (error out=w2296:errorcluster)  [unwired: 1 in, 2 out]
              }
            }
          }
          frame "Hidden", "Hide" {
            w2297 = T20."Hidden" ("State")
            n1052 = property on="Property Node" class="VI"(reference=w2303, error in=w2302) -> (reference out=w2300:refnum<vi>, error out=w2301:errorcluster, "FP.State"=w2299:T20)
            n1053 = Not Equal?(x=w2299, y=w2297) -> (x != y?=w2298:bool)
            n1054 = case shown="True" w2298 {
              tunnel: [w2308 w2309] -> w2304
              tunnel: w2301 -> [w2307 w2309]
              tunnel: w2300 -> [w2306 _]
              tunnel: w2297 -> [w2305 _]
              frame True {
                n1055 = invoke on="Invoke Node" class="VI" method="FP.Open"(reference=w2306, error in=w2307, "State"=w2305) -> (error out=w2308:errorcluster)  [unwired: 2 in, 4 out]
              }
              frame False {
              }
            }
          }
          frame "Minimize", "Minimized" {
            w2310 = T20."Minimized" ("State")
            n1056 = property on="Property Node" class="VI"(reference=w2316, error in=w2315) -> (reference out=w2313:refnum<vi>, error out=w2314:errorcluster, "FP.State"=w2312:T20)
            n1057 = Not Equal?(x=w2312, y=w2310) -> (x != y?=w2311:bool)
            n1058 = case shown="True" w2311 {
              tunnel: [w2321 w2322] -> w2317
              tunnel: w2314 -> [w2320 w2322]
              tunnel: w2313 -> [w2319 _]
              tunnel: w2310 -> [w2318 _]
              frame True {
                n1059 = invoke on="Invoke Node" class="VI" method="FP.Open"(reference=w2319, error in=w2320, "State"=w2318) -> (error out=w2321:errorcluster)  [unwired: 2 in, 4 out]
              }
              frame False {
              }
            }
          }
          frame "Maximize", "Maximized" {
            w2323 = T20."Maximized" ("State")
            n1060 = property on="Property Node" class="VI"(reference=w2329, error in=w2328) -> (reference out=w2326:refnum<vi>, error out=w2327:errorcluster, "FP.State"=w2325:T20)
            n1061 = Not Equal?(x=w2325, y=w2323) -> (x != y?=w2324:bool)
            n1062 = case shown="True" w2324 {
              tunnel: [w2334 w2335] -> w2330
              tunnel: w2327 -> [w2333 w2335]
              tunnel: w2326 -> [w2332 _]
              tunnel: w2323 -> [w2331 _]
              frame True {
                n1063 = invoke on="Invoke Node" class="VI" method="FP.Open"(reference=w2332, error in=w2333, "State"=w2331) -> (error out=w2334:errorcluster)  [unwired: 2 in, 4 out]
              }
              frame False {
              }
            }
          }
        }
        n1064 = call <vilib>:"Add State(s) to Queue__JKI_lib_State_Machine.vi"("State(s) in (\"\")"=w2270) -> ("States Out"=w2269:string)  [unwired: 14 in]
      }
      frame "---------- AimingBeam ----------" {
        # "Template Separator\n(You can make a copy of, or modify, this frame)"
        n1065 = call <vilib>:"Add State(s) to Queue__JKI_lib_State_Machine.vi"("State(s) in (\"\")"=w2340) -> ("States Out"=w2339:string)  [unwired: 14 in]
      }
      frame "AimingBeam: Initialize" {
        # "set aiming beam button color"
        # "Open COM port for Aiming Beam\n(Require USB connection)"
        n1066 = Unbundle By Name(w2342) -> ("AB Cluster.Aiming Beam COM Port"=w2350:refnum<visa-resource-name>)
        n1067 = call-poly "VISA Configure Serial Port"("VISA resource name"=w2350, "Enable Termination\nChar (T)"=TRUE ("Enable Termination\nChar (T)"), "baud rate (9600)"=u32 9600, "error in (no error)"=w2347) -> ("error out"=w2346:errorcluster)  [unwired: 10 in, 1 out]
        n1068 = Unbundle By Name(w2346) -> ("status"=w2345:bool)
        n1069 = Not(x=w2345) -> (.not. x?=w2344:bool)
        n1070 = Bundle By Name(cluster=w2342, "System Status.Aiming Beam"=w2344) -> (w2343:T25)
        n1071 = call <vilib>:"Add State(s) to Queue__JKI_lib_State_Machine.vi"("State(s) in (\"\")"=w2352) -> ("States Out"=w2351:string)  [unwired: 14 in]
      }
      frame "AimingBeam: Close" {
        # "Close Aiming Beam COM port\n(Require USB connection to Aiming Beam Laser)"
        n1072 = Unbundle By Name(w2355) -> ("AB Cluster.Aiming Beam COM Port"=w2359:refnum<visa-resource-name>)
        n1073 = VISA Close(VISA resource name=w2359, error in (no error)=w2357) -> (error out=w2358:errorcluster)
        n1074 = Bundle By Name(cluster=w2355, "System Status.Aiming Beam"=FALSE) -> (w2356:T25)
        n1075 = call <vilib>:"Add State(s) to Queue__JKI_lib_State_Machine.vi"("State(s) in (\"\")"=w2361) -> ("States Out"=w2360:string)  [unwired: 14 in]
      }
      frame "AimingBeam: Set Current" {
        # "Set Aiming Beam Current\n(You can make a copy of, or modify, this frame)"
        n1076 = Unbundle By Name(w2376) -> ("AB Cluster.Aiming Beam COM Port"=w2369:refnum<visa-resource-name>, "AB Cluster.Max Current"=w2365:dbl, "AB Cluster.Default Current"=w2367:dbl, "AB Cluster.Min Current"=w2366:dbl)
        n1077 = In Range and Coerce(upper limit=w2365, x=w2367, lower limit=w2366) -> (coerced(x)=w2362:dbl)  [unwired: 1 out]
        n1078 = Number To Fractional String(number=w2362, precision (6)=i16 2) -> (F-format string=w2370:string)  [unwired: 2 in]
        n1079 = Concatenate Strings("slc:", w2370, "\r" ("Carriage Return Constant"), "\n" ("Line Feed Constant")) -> (w2373:string)
        n1080 = VISA Write(VISA resource name=w2369, write buffer=w2373, error in (no error)=w2364) -> (error out=w2368:errorcluster)  [unwired: 2 out]
        n1081 = call <vilib>:"Add State(s) to Queue__JKI_lib_State_Machine.vi"("State(s) in (\"\")"=w2378) -> ("States Out"=w2377:string)  [unwired: 14 in]
      }
      frame "AimingBeam: Set Status" {
        # "Enable Aiming Beam\n(Usage: \"AimingBeam: Set >> Enable|Disable\")"
        n1082 = Unbundle By Name(w2385) -> ("AB Cluster.Aiming Beam COM Port"=w2382:refnum<visa-resource-name>)
        n1083 = case shown="\"Enable\"" w2384 {
          tunnel: [w2388 w2392] -> w2383
          frame "Disable", Default {
            n1084 = Concatenate Strings("cof", "\r" ("Carriage Return Constant"), "\n" ("Line Feed Constant")) -> (w2388:string)
          }
          frame "Enable" {
            n1085 = Concatenate Strings("con", "\r" ("Carriage Return Constant"), "\n" ("Line Feed Constant")) -> (w2392:string)
          }
        }
        n1086 = VISA Write(VISA resource name=w2382, write buffer=w2383, error in (no error)=w2380) -> (error out=w2381:errorcluster)  [unwired: 2 out]
        n1087 = call <vilib>:"Add State(s) to Queue__JKI_lib_State_Machine.vi"("State(s) in (\"\")"=w2387) -> ("States Out"=w2386:string)  [unwired: 14 in]
      }
      frame "AimingBeam: GetPWMStatus" {
        # "Get aiming beam PWM status\n()"
        n1088 = Unbundle By Name(w2400) -> ("AB Cluster.Freq"=w2399:i32, "LJ Pinout.AimingBeam PWM"=w2406:string)
        n1089 = Equal To 0?(x=w2399) -> (x = 0?=w2398:bool)
        n1090 = call "LabJack_FGV.vi"("Operation(Read)"=enum16{"Write", "Read"}."Read" ("Operation"), "error in (no error)"=w2402) -> ("error out"=w2404:errorcluster, "Read data"=w2405:i32)  [unwired: 8 in]
        n1091 = case shown="True" w2398 {
          tunnel: w2406 -> [w2419 _]
          tunnel: [w2417 "DIO_STATE"] -> w2403
          frame False {
            n1092 = Concatenate Strings(w2419, "_EF_ENABLE" ("string")) -> (w2417:string)
          }
          frame True {
          }
        }
        n1093 = call "LJM_eReadName.vi"("Handle In"=w2405, "Name"=w2403, "error in"=w2404) -> ("Value"=w2397:dbl, "error out"=w2401:errorcluster)  [unwired: 10 in, 1 out]
        n1094 = case shown="True" w2398 {
          tunnel: w2397 -> [w2412 w2416]
          tunnel: [w2411 w2413] -> w2396
          frame False {
            n1095 = Greater Than 0?(x=w2412) -> (x > 0?=w2411:bool)
          }
          frame True {
            n1096 = Number To Boolean Array(number=w2416) -> (Boolean array=w2415:bool[])
            n1097 = Index Array(array=w2415, index=3) -> (element=w2413:bool)
          }
        }
        n1098 = case shown="False" w2396 {
          frame False {
            # "PWM is off\nset color to dark green"
            n1099 = local write "Aiming beam toggle"(FALSE ("Aimging beam")) -> ()
          }
          frame True {
            # "PWM is on\nset color to light green"
            n1100 = local write "Aiming beam toggle"(TRUE ("Aimging beam")) -> ()
          }
        }
        n1101 = call <vilib>:"Add State(s) to Queue__JKI_lib_State_Machine.vi"("State(s) in (\"\")"=w2410) -> ("States Out"=w2409:string)  [unwired: 14 in]
      }
      frame "---------- 355 Laser ----------" {
        # "Template Separator\n(You can make a copy of, or modify, this frame)"
        n1102 = call <vilib>:"Add State(s) to Queue__JKI_lib_State_Machine.vi"("State(s) in (\"\")"=w2427) -> ("States Out"=w2426:string)  [unwired: 14 in]
      }
      frame "355 Laser: Check Dewelling" {
        # "if time laser start time is less than 7.5s before, wait 250ms then check again."
        # "Template Separator\n(You can make a copy of, or modify, this frame)"
        n1103 = Unbundle By Name(w2435) -> ("Laser start tic"=w2432:u32)
        n1104 = Tick Count (ms)() -> (millisecond timer value=w2433:u32)
        n1105 = Subtract(x=w2433, y=w2432) -> (x-y=w2431:u32)
        n1106 = Greater?(x=w2431, y=u32 5000) -> (0:w2429:bool)
        n1107 = case shown="False" w2429 {
          tunnel: ["355 Laser: Check Dewelling" ""] -> w2428
          frame False {
            n1108 = Wait (ms)(milliseconds to wait=u32 250) -> ()  [unwired: 1 out]
          }
          frame True {
          }
        }
        n1109 = call <vilib>:"Add State(s) to Queue__JKI_lib_State_Machine.vi"("State(s) in Front (\"\")"=w2428, "State(s) in (\"\")"=w2438) -> ("States Out"=w2437:string)  [unwired: 13 in]
      }
      frame "355 Laser: Laser enable" {
        # "Laser enable/disable\n(Usage: \"LabJack: Laser enable/disable >> 1|0\")"
        n1110 = Unbundle By Name(w2445) -> ("LJ Pinout.Laser Start/Stop"=w2449:string, "System Status.355 Laser"=w2443:bool)
        n1111 = case shown="False" w2443 {
          tunnel: w2442 -> [w2464 w2465]
          tunnel: w2449 -> [w2458 _]
          tunnel: [w2453 w2465] -> w2447
          tunnel: [w2452 u32 0 ("millisecond timer value")] -> w2444
          frame False {
            n1112 = call "LabJack_FGV.vi"("Operation(Read)"=enum16{"Write", "Read"}."Read" ("Operation")) -> ("Read data"=w2460:i32)  [unwired: 9 in, 1 out]
            n1113 = call "LJM_eWriteName.vi"("Handle In"=w2460, "Name"=w2458, "Value"=1.0, "error in"=w2464) -> ("Handle Out"=w2459:i32, "error out"=w2457:errorcluster)  [unwired: 10 in]
            n1114 = call <userlib>:"Wait (ms)__ogtk.vi"("error in (no error)"=w2457, "milliseconds to wait"=u32 250) -> ("error out"=w2456:errorcluster)  [unwired: 8 in, 1 out]
            n1115 = call "LJM_eWriteName.vi"("Handle In"=w2459, "Name"=w2458, "Value"=0.0, "error in"=w2456) -> ("error out"=w2454:errorcluster)  [unwired: 10 in, 1 out]
            n1116 = call <userlib>:"Tick Count (ms)__ogtk.vi"("error in (no error)"=w2454) -> ("error out"=w2453:errorcluster, "millisecond timer value"=w2452:u32)  [unwired: 9 in]
          }
          frame True {
          }
        }
        n1117 = Bundle By Name(cluster=w2445, "Laser start tic"=w2444) -> (w2446:T25)
        n1118 = call <vilib>:"Add State(s) to Queue__JKI_lib_State_Machine.vi"("State(s) in (\"\")"=w2451) -> ("States Out"=w2450:string)  [unwired: 14 in]
      }
      frame "355 Laser: Laser disable" {
        # "Laser enable/disable\n(Usage: \"LabJack: Laser enable/disable >> 1|0\")"
        n1119 = Unbundle By Name(w2469) -> ("LJ Pinout.Laser Start/Stop"=w2473:string, "System Status.355 Laser"=w2467:bool)
        n1120 = case shown="True" w2467 {
          tunnel: w2474 -> [w2477 w2491]
          tunnel: w2473 -> [_ w2485]
          tunnel: [w2477 w2480] -> w2471
          tunnel: [u32 0 ("millisecond timer value") w2479] -> w2468
          frame False {
          }
          frame True {
            n1121 = call "LabJack_FGV.vi"("Operation(Read)"=enum16{"Write", "Read"}."Read" ("Operation")) -> ("Read data"=w2487:i32)  [unwired: 9 in, 1 out]
            n1122 = call "LJM_eWriteName.vi"("Handle In"=w2487, "Name"=w2485, "Value"=1.0, "error in"=w2491) -> ("Handle Out"=w2486:i32, "error out"=w2484:errorcluster)  [unwired: 10 in]
            n1123 = call <userlib>:"Wait (ms)__ogtk.vi"("error in (no error)"=w2484, "milliseconds to wait"=u32 250) -> ("error out"=w2483:errorcluster)  [unwired: 8 in, 1 out]
            n1124 = call "LJM_eWriteName.vi"("Handle In"=w2486, "Name"=w2485, "Value"=0.0, "error in"=w2483) -> ("error out"=w2481:errorcluster)  [unwired: 10 in, 1 out]
            n1125 = call <userlib>:"Tick Count (ms)__ogtk.vi"("error in (no error)"=w2481) -> ("error out"=w2480:errorcluster, "millisecond timer value"=w2479:u32)  [unwired: 9 in]
          }
        }
        n1126 = Bundle By Name(cluster=w2469, "Laser start tic"=w2468) -> (w2470:T25)
        n1127 = call <vilib>:"Add State(s) to Queue__JKI_lib_State_Machine.vi"("State(s) in (\"\")"=w2476) -> ("States Out"=w2475:string)  [unwired: 14 in]
      }
      frame "355 Laser: Dewelling" {
        # "Wait some time (ms)\n(355 Laser: Dewelling >> #)"
        n1128 = Fract/Exp String To Number(string=w2495, default (0 dbl)=0) -> (number=w2493:i32)  [unwired: 2 in, 1 out]
        n1129 = Wait (ms)(milliseconds to wait=w2493) -> ()  [unwired: 1 out]
        n1130 = call <vilib>:"Add State(s) to Queue__JKI_lib_State_Machine.vi"("State(s) in (\"\")"=w2499) -> ("States Out"=w2498:string)  [unwired: 14 in]
      }
      frame "355 Laser: Close" {
        # "Template Separator\n(You can make a copy of, or modify, this frame)"
        n1131 = call <vilib>:"Add State(s) to Queue__JKI_lib_State_Machine.vi"("State(s) in Front (\"\")"="355 Laser: CheckControllerStatus\n355 Laser: Laser disable\n355 Laser: Dewelling >>1000", "State(s) in (\"\")"=w2505) -> ("States Out"=w2504:string)  [unwired: 13 in]
      }
      frame "355 Laser: CheckControllerStatus" {
        # "if average < 2, laser no power\nif average 2 < average < 9.3, laser on\nif 9.3<average<10, interlock open, blink indicator\nif average > 10, laser off\n[Covers: REQ30]"
        # "take 10 measuremt and look at average"
        # "Check 355 laser controller status\nBy probing Emisison Lamp negative terminal voltage"
        n1132 = Unbundle By Name(w2514) -> ("LJ Pinout.Laser Ready"=w2517:string)
        n1133 = call "LabJack_FGV.vi"("Operation(Read)"=enum16{"Write", "Read"}."Read" ("Operation")) -> ("Read data"=w2518:i32)  [unwired: 9 in, 1 out]
        n1134 = for {
          N: 20 -> [_]
          tunnel: w2518 -> [w2529]
          tunnel: w2517 -> [w2528]
          shift-right: [w2527] -> w2510
          shift-left: w2516 -> [w2526]
          tunnel: [w2524] -> w2509 mode=indexing
          n1135 = call "LJM_eReadName.vi"("Handle In"=w2529, "Name"=w2528, "error in"=w2526) -> ("Value"=w2524:dbl, "error out"=w2527:errorcluster)  [unwired: 10 in, 1 out]
          n1136 = Wait (ms)(milliseconds to wait=u32 25) -> ()  [unwired: 1 out]
        }
        n1137 = call "checkLaserStatus.vi"("error in (no error)"=w2510, "Laser LED voltage"=w2509) -> ("error out"=w2511:errorcluster, "Interlock open?"=w2506:bool, "Laser on?"=w2508:bool, "Mean voltage"=→"laser EM lamp V":dbl)  [unwired: 6 in]
        n1138 = Bundle By Name(cluster=w2514, "System Status.355 Laser"=w2508) -> (w2515:T25)
        n1139 = case shown="True" w2506 {
          frame False {
            n1140 = property on="355 Laser" class="Bool (strict)"("Blinking"=FALSE) -> ()  [unwired: 2 in, 2 out]
          }
          frame True {
            n1141 = property on="355 Laser" class="Bool (strict)"("Blinking"=TRUE) -> ()  [unwired: 2 in, 2 out]
          }
        }
        n1142 = call <vilib>:"Add State(s) to Queue__JKI_lib_State_Machine.vi"("State(s) in (\"\")"=w2521) -> ("States Out"=w2520:string)  [unwired: 14 in]
      }
      frame "355 Laser: CheckPWMStatus" {
        # "Check 355 laser PWM status\n(Read LJ DIO#EF_ENABLE register to determine PWM status)"
        n1143 = Unbundle By Name(w2539) -> ("LJ Pinout.355 PWM"=w2538:string)
        n1144 = call "LabJack_FGV.vi"("Operation(Read)"=enum16{"Write", "Read"}."Read" ("Operation"), "error in (no error)"=w2532) -> ("error out"=w2535:errorcluster, "Read data"=w2536:i32)  [unwired: 8 in]
        n1145 = Concatenate Strings(w2538, "_EF_ENABLE" ("string")) -> (w2534:string)
        n1146 = call "LJM_eReadName.vi"("Handle In"=w2536, "Name"=w2534, "error in"=w2535) -> ("Value"=w2531:dbl, "error out"=w2533:errorcluster)  [unwired: 10 in, 1 out]
        n1147 = Greater Than 0?(x=w2531) -> (x > 0?=w2530:bool)
        n1148 = case shown="False" w2530 {
          frame False {
            # "PWM is off\nset color to gray"
            n1149 = local write "355nm Laser toggle"(FALSE ("355nm Laser")) -> ()
          }
          frame True {
            # "PWM is on\nset color to light green"
            n1150 = local write "355nm Laser toggle"(TRUE ("355nm Laser")) -> ()
          }
        }
        n1151 = call <vilib>:"Add State(s) to Queue__JKI_lib_State_Machine.vi"("State(s) in (\"\")"=w2543) -> ("States Out"=w2542:string)  [unwired: 14 in]
      }
      frame "355 Laser: Start" {
        # "Template Separator\n(You can make a copy of, or modify, this frame)"
        n1152 = call <vilib>:"Add State(s) to Queue__JKI_lib_State_Machine.vi"("State(s) in Front (\"\")"="LabJack: 355_PWM_Start", "State(s) in (\"\")"=w2551) -> ("States Out"=w2550:string)  [unwired: 13 in]
      }
      frame "355 Laser: Stop" {
        # "Template Separator\n(You can make a copy of, or modify, this frame)"
        n1153 = call <vilib>:"Add State(s) to Queue__JKI_lib_State_Machine.vi"("State(s) in Front (\"\")"="LabJack: 355_PWM_Stop", "State(s) in (\"\")"=w2557) -> ("States Out"=w2556:string)  [unwired: 13 in]
      }
      frame "---------- Utility ----------" {
        # "Template Separator\n(You can make a copy of, or modify, this frame)"
        n1154 = call <vilib>:"Add State(s) to Queue__JKI_lib_State_Machine.vi"("State(s) in (\"\")"=w2562) -> ("States Out"=w2561:string)  [unwired: 14 in]
      }
      frame "Utility: SetDataClass" {
        # "Set Data Class in Queues\n(Set data class to either Data, Bg or Cali)"
        n1155 = case shown="\"Cali\"" w2564 {
          tunnel: [enum16{"Data", "BG", "Cali"}."Data" ("Data Class") enum16{"Data", "BG", "Cali"}."BG" ("Data Class") enum16{"Data", "BG", "Cali"}."Cali" ("Data Class")] -> w2563
          frame "Data", Default {
          }
          frame "Bg" {
          }
          frame "Cali" {
          }
        }
        n1156 = local write "Data Class"(w2563) -> ()
        n1157 = call <vilib>:"Add State(s) to Queue__JKI_lib_State_Machine.vi"("State(s) in (\"\")"=w2569) -> ("States Out"=w2568:string)  [unwired: 14 in]
      }
      frame "Utility: AquiTimerReset" {
        # "Set Aquisition Timer\n(You can make a copy of, or modify, this frame)"
        n1158 = Tick Count (ms)() -> (millisecond timer value=w2575:u32)
        n1159 = Bundle By Name(cluster=w2573, "Aquisition Timer"=w2575) -> (w2574:T25)
        n1160 = call <vilib>:"Add State(s) to Queue__JKI_lib_State_Machine.vi"("State(s) in (\"\")"=w2579) -> ("States Out"=w2578:string)  [unwired: 14 in]
      }
      frame "Utility: AquiTimerCheck" {
        # "5min to ms"
        # "Set Aquisition Timer\n([Covers: REQ35])"
        n1161 = Unbundle By Name(w2587) -> ("Aquisition Timer"=w2585:u32)
        n1162 = Tick Count (ms)() -> (millisecond timer value=w2586:u32)
        n1163 = Subtract(x=w2586, y=w2585) -> (x-y=w2584:u32)
        n1164 = Multiply(x=1000, y=300) -> (x*y=w2581:i32)
        n1165 = Greater Or Equal?(x=w2584, y=w2581) -> (x >= y?=w2580:bool)
        n1166 = case shown="True" w2580 {
          frame False {
            # "do nothing"
          }
          frame True {
            # "if timed out, stop aquisition"
            n1167 = property on="StopButton" class="Bool (strict)"("Val(Sgnl)"=TRUE ("Value (Signaling)")) -> ()  [unwired: 2 in, 2 out]
          }
        }
        n1168 = call <vilib>:"Add State(s) to Queue__JKI_lib_State_Machine.vi"("State(s) in (\"\")"=w2591) -> ("States Out"=w2590:string)  [unwired: 14 in]
      }
      frame "Utility: StartBeep" {
        # "Beep\n([Covers: REQ18])"
        n1169 = call <vilib>:"Beep.vi"("use system alert? (T)"=FALSE, "duration (msec)"=u32 1000, "frequency (Hz)"=u32 2000) -> ()  [unwired: 9 in]
        n1170 = call <vilib>:"Add State(s) to Queue__JKI_lib_State_Machine.vi"("State(s) in (\"\")"=w2600) -> ("States Out"=w2599:string)  [unwired: 14 in]
      }
      frame "Utility: EndBeep" {
        # "Beep\n([Covers: REQ18])"
        n1171 = flat-sequence {
          frame #0 {
            n1172 = call <vilib>:"Beep.vi"("use system alert? (T)"=FALSE, "duration (msec)"=u32 500, "frequency (Hz)"=u32 2000) -> ()  [unwired: 9 in]
          }
          frame #1 {
            n1173 = call <vilib>:"Beep.vi"("use system alert? (T)"=FALSE, "duration (msec)"=u32 500, "frequency (Hz)"=u32 2000) -> ()  [unwired: 9 in]
          }
        }
        n1174 = call <vilib>:"Add State(s) to Queue__JKI_lib_State_Machine.vi"("State(s) in (\"\")"=w2605) -> ("States Out"=w2604:string)  [unwired: 14 in]
      }
      frame "Utility: RestoreDeConChan" {
        # "Template Separator\n(You can make a copy of, or modify, this frame)"
        n1175 = global read "GlobalVariables.vi" "DeconChan Temp"() -> (w2612:T48)
        n1176 = local write "Radio Buttons"(w2612) -> ()
        n1177 = call <vilib>:"Add State(s) to Queue__JKI_lib_State_Machine.vi"("State(s) in (\"\")"=w2617) -> ("States Out"=w2616:string)  [unwired: 14 in]
      }
      frame "Utility: SaveDeconChan" {
        # "Save Decon Channel to global temp\n(You can make a copy of, or modify, this frame)"
        n1178 = flat-sequence {
          frame #0 {
            n1179 = local read "Radio Buttons"() -> (w2623:enum32{"No Selection", "Ch1", "Ch2", "Ch3"})
            n1180 = global write "GlobalVariables.vi" "DeconChan Temp"(w2623) -> ()
          }
          frame #1 {
            n1181 = local write "Radio Buttons"(enum32{"No Selection", "Ch1", "Ch2", "Ch3"}."No Selection" ("Radio Buttons")) -> ()
          }
        }
        n1182 = flat-sequence {
          frame #0 {
          }
          frame #1 {
            (unwired) enum32{"No Selection", "Ch1", "Ch2", "Ch3"}."No Selection" ("Radio Buttons")
          }
        }
        n1183 = call <vilib>:"Add State(s) to Queue__JKI_lib_State_Machine.vi"("State(s) in (\"\")"=w2622) -> ("States Out"=w2621:string)  [unwired: 14 in]
      }
      frame "Utility: Dewelling" {
        # "Main loop dewell\n(Dewelling >> #)"
        n1184 = Fract/Exp String To Number(string=w2628, default (0 dbl)=0) -> (number=w2626:i32)  [unwired: 2 in, 1 out]
        n1185 = Wait (ms)(milliseconds to wait=w2626) -> ()  [unwired: 1 out]
        n1186 = call <vilib>:"Add State(s) to Queue__JKI_lib_State_Machine.vi"("State(s) in (\"\")"=w2632) -> ("States Out"=w2631:string)  [unwired: 14 in]
      }
      frame "Utility: SetAllChanManualGain" {
        # "Template Separator\n(You can make a copy of, or modify, this frame)"
        n1187 = property on="Auto gain ch1" class="Bool (strict)"("Val(Sgnl)"=FALSE ("Value (Signaling)")) -> ()  [unwired: 2 in, 2 out]
        n1188 = property on="Auto gain ch2" class="Bool (strict)"("Val(Sgnl)"=FALSE ("Value (Signaling)")) -> ()  [unwired: 2 in, 2 out]
        n1189 = property on="Auto gain ch3" class="Bool (strict)"("Val(Sgnl)"=FALSE ("Value (Signaling)")) -> ()  [unwired: 2 in, 2 out]
        n1190 = call <vilib>:"Add State(s) to Queue__JKI_lib_State_Machine.vi"("State(s) in (\"\")"=w2640) -> ("States Out"=w2639:string)  [unwired: 14 in]
      }
      frame "Utility: SetAllChanAutoGain" {
        # "Template Separator\n(You can make a copy of, or modify, this frame)"
        n1191 = property on="Auto gain ch1" class="Bool (strict)"("Val(Sgnl)"=TRUE ("Value (Signaling)")) -> ()  [unwired: 2 in, 2 out]
        n1192 = property on="Auto gain ch2" class="Bool (strict)"("Val(Sgnl)"=TRUE ("Value (Signaling)")) -> ()  [unwired: 2 in, 2 out]
        n1193 = property on="Auto gain ch3" class="Bool (strict)"("Val(Sgnl)"=TRUE ("Value (Signaling)")) -> ()  [unwired: 2 in, 2 out]
        n1194 = call <vilib>:"Add State(s) to Queue__JKI_lib_State_Machine.vi"("State(s) in (\"\")"=w2648) -> ("States Out"=w2647:string)  [unwired: 14 in]
      }
      frame "---------- SysLog ----------" {
        # "Template Separator\n(You can make a copy of, or modify, this frame)"
        n1195 = call <vilib>:"Add State(s) to Queue__JKI_lib_State_Machine.vi"("State(s) in (\"\")"=w2653) -> ("States Out"=w2652:string)  [unwired: 14 in]
      }
      frame "SysLog: OpenLogFile" {
        # "Template Separator\n(You can make a copy of, or modify, this frame)"
        n1196 = call <vilib>:"Add State(s) to Queue__JKI_lib_State_Machine.vi"("State(s) in (\"\")"=w2658) -> ("States Out"=w2657:string)  [unwired: 14 in]
      }
      frame "---------- Graph ----------" {
        # "Template Separator\n(You can make a copy of, or modify, this frame)"
        n1197 = call <vilib>:"Add State(s) to Queue__JKI_lib_State_Machine.vi"("State(s) in (\"\")"=w2663) -> ("States Out"=w2662:string)  [unwired: 14 in]
      }
      frame "Graph: SetXMultiplier" {
        # "Set X multiplier of WF graphs\n(You can make a copy of, or modify, this frame)"
        n1198 = call "Digitizer1_FGV.vi"() -> ("error out"=w2667:errorcluster, "Read data"=w2668:refnum<k15>)  [unwired: 10 in]
        n1199 = property class="niScope"(reference=w2668, error in=w2667) -> ("Min Sample Rate"=w2666:dbl)  [unwired: 2 out]
        n1200 = Divide(x=1.0, y=w2666) -> (x/y=w2664:dbl)
        n1201 = property on="Channel 1" class="WFGraph (strict)"("XScale.Multiplier"=w2664) -> ()  [unwired: 2 in, 2 out]
        n1202 = property on="Channel 2" class="WFGraph (strict)"("XScale.Multiplier"=w2664) -> ()  [unwired: 2 in, 2 out]
        n1203 = property on="Channel 3" class="WFGraph (strict)"("XScale.Multiplier"=w2664) -> ()  [unwired: 2 in, 2 out]
        n1204 = call <vilib>:"Add State(s) to Queue__JKI_lib_State_Machine.vi"("State(s) in (\"\")"=w2673) -> ("States Out"=w2672:string)  [unwired: 14 in]
      }
      frame "Graph: AddCursors" {
        # "Add BG and DC cursor to all graphs\n(You can make a copy of, or modify, this frame)"
        n1205 = property on="Channel 1" class="WFGraph (strict)"() -> ("XScale.Multiplier"=w2680:dbl)  [unwired: 2 in, 2 out]
        n1206 = global read "GlobalVariables.vi" "DC Idx1"() -> (w2679:i32)
        n1207 = global read "GlobalVariables.vi" "DC Idx2"() -> (w2678:i32)
        n1208 = global read "GlobalVariables.vi" "BG Idx1"() -> (w2677:i32)
        n1209 = global read "GlobalVariables.vi" "BG Idx2"() -> (w2676:i32)
        n1210 = property on="Channel 2" class="WFGraph (strict)"() -> ("CrsrList"=w2688:T26)  [unwired: 2 in, 2 out]
        n1211 = property on="Channel 3" class="WFGraph (strict)"() -> ("CrsrList"=w2687:T26)  [unwired: 2 in, 2 out]
        n1212 = property on="Channel 1" class="WFGraph (strict)"(error in=w2682) -> ("CrsrList"=w2691:T26)  [unwired: 1 in, 2 out]
        n1213 = Build Array(w2679, w2678, w2677, w2676) -> (w2675:i32[])
        n1214 = Multiply(x=w2675, y=w2680) -> (x*y=w2674:dbl[])
        n1215 = for {
          tunnel: w2691 -> [w2703] mode=indexing
          tunnel: w2674 -> [w2699] mode=indexing
          tunnel: [w2702] -> w2690 mode=indexing
          tunnel: u32[] [6618880, 6618880, 16711680, 16711680] -> [w2698] mode=indexing
          tunnel: w2688 -> [w2701] mode=indexing
          tunnel: w2687 -> [w2700] mode=indexing
          tunnel: [w2697] -> w2686 mode=indexing
          tunnel: [w2696] -> w2685 mode=indexing
          n1216 = Bundle By Name(cluster=w2703, "Position.X"=w2699, "Color"=w2698) -> (w2702:T27)
          n1217 = Bundle By Name(cluster=w2701, "Position.X"=w2699, "Color"=w2698) -> (w2697:T27)
          n1218 = Bundle By Name(cluster=w2700, "Position.X"=w2699, "Color"=w2698) -> (w2696:T27)
        }
        n1219 = control-ref of="Channel 1"() -> (w2684:refnum<vi>)
        n1220 = property on="Channel 1" class="WFGraph (strict)"("CrsrList"=w2690) -> (error out=w2681:errorcluster)  [unwired: 2 in, 1 out]
        n1221 = property on="Channel 2" class="WFGraph (strict)"("CrsrList"=w2686) -> ()  [unwired: 2 in, 2 out]
        n1222 = property on="Channel 3" class="WFGraph (strict)"("CrsrList"=w2685) -> ()  [unwired: 2 in, 2 out]
        n1223 = call "UpdateCurserIdx(SubVI).vi"("error in (no error)"=w2681, "WaveformGraph in"=w2684) -> ("error out"=w2683:errorcluster)  [unwired: 9 in]
        n1224 = call <vilib>:"Add State(s) to Queue__JKI_lib_State_Machine.vi"("State(s) in (\"\")"=w2695) -> ("States Out"=w2694:string)  [unwired: 14 in]
      }
      frame "Graph: SaveCursorLoc" {
        # "Save cursor location to ini file\n(Save cursor location to system setting ini file)"
        n1225 = global read "GlobalVariables.vi" "DC Idx1"() -> (w2710:i32)
        n1226 = global read "GlobalVariables.vi" "DC Idx2"() -> (w2709:i32)
        n1227 = global read "GlobalVariables.vi" "BG Idx1"() -> (w2708:i32)
        n1228 = global read "GlobalVariables.vi" "BG Idx2"() -> (w2707:i32)
        n1229 = Bundle("DC Idx1"=w2710, "DC Idx2"=w2709, "BG Idx1"=w2708, "BG Idx2"=w2707) -> (w2706:T49)  [unwired: 1 in]
        n1230 = call "writeCursorConfigMain.vi"("error in (no error)"=w2704, "Cursor Locations"=w2706) -> ("error out"=w2705:errorcluster)  [unwired: 9 in]
        n1231 = call <vilib>:"Add State(s) to Queue__JKI_lib_State_Machine.vi"("State(s) in (\"\")"=w2714) -> ("States Out"=w2713:string)  [unwired: 14 in]
      }
      frame "---------- APD ----------" {
        # "Template Separator\n(You can make a copy of, or modify, this frame)"
        n1232 = call <vilib>:"Add State(s) to Queue__JKI_lib_State_Machine.vi"("State(s) in (\"\")"=w2719) -> ("States Out"=w2718:string)  [unwired: 14 in]
      }
      frame "APD: Initialize" {
        w2726 = enum16{"Read", "Write"}."Write" ("Operation (Read)")
        w2725 = refnum<class "APDClass.lvclass"> refnum  # APDClass.lvclass
        # "Initialize APD FGV\n(Initialized APD FGV for holding data)"
        n1233 = call "APD1FGV.vi"("Error In"=w2720, "Operation (Read)"=w2726, "APDClass in"=w2725) -> ("Error Out"=w2724:errorcluster)  [unwired: 7 in, 1 out]
        n1234 = call "APD2FGV.vi"("Error In"=w2720, "Operation (Read)"=w2726, "APDClass in"=w2725) -> ("Error Out"=w2723:errorcluster)  [unwired: 7 in, 1 out]
        n1235 = call "APD3FGV.vi"("Error In"=w2720, "Operation (Read)"=w2726, "APDClass in"=w2725) -> ("Error Out"=w2722:errorcluster)  [unwired: 7 in, 1 out]
        n1236 = Merge Errors(w2724, w2723, w2722) -> (w2721:errorcluster)
        n1237 = call <vilib>:"Add State(s) to Queue__JKI_lib_State_Machine.vi"("State(s) in (\"\")"=w2730) -> ("States Out"=w2729:string)  [unwired: 14 in]
      }
      frame "APD: LoadFromSerial" {
        w2739 = enum16{"Read", "Write"}."Write" ("Operation (Read)")
        # "Load APD data from tdms file\n(load and update FGV)"
        n1238 = call "readAPDSerial.vi"("Error In"=w2734) -> ("Error Out"=w2733:errorcluster, "output cluster"=w2732:T41)  [unwired: 9 in]
        n1239 = Unbundle By Name(w2732) -> ("Ch1APDSerial#"=w2747:string, "Ch2APDSerial#"=w2731:string, "Ch3APDSerial#"=w2746:string)
        n1240 = call "CreatFromSerialNumNoRaw.vi"("error in (no error)"=w2733, "APD Serial #"=w2731) -> ("error out"=w2742:errorcluster, "APDClass out"=w2743:refnum<class "APDClass.lvclass">)  [unwired: 8 in]
        n1241 = call "CreatFromSerialNumNoRaw.vi"("error in (no error)"=w2733, "APD Serial #"=w2746) -> ("error out"=w2740:errorcluster, "APDClass out"=w2741:refnum<class "APDClass.lvclass">)  [unwired: 8 in]
        n1242 = call "CreatFromSerialNumNoRaw.vi"("error in (no error)"=w2733, "APD Serial #"=w2747) -> ("error out"=w2744:errorcluster, "APDClass out"=w2745:refnum<class "APDClass.lvclass">)  [unwired: 8 in]
        n1243 = call "APD1FGV.vi"("Error In"=w2744, "Operation (Read)"=w2739, "APDClass in"=w2745) -> ("Error Out"=w2738:errorcluster)  [unwired: 7 in, 1 out]
        n1244 = call "APD2FGV.vi"("Error In"=w2742, "Operation (Read)"=w2739, "APDClass in"=w2743) -> ("Error Out"=w2736:errorcluster)  [unwired: 7 in, 1 out]
        n1245 = call "APD3FGV.vi"("Error In"=w2740, "Operation (Read)"=w2739, "APDClass in"=w2741) -> ("Error Out"=w2737:errorcluster)  [unwired: 7 in, 1 out]
        n1246 = Merge Errors(w2738, w2736, w2737) -> (w2735:errorcluster)
        n1247 = call <vilib>:"Add State(s) to Queue__JKI_lib_State_Machine.vi"("State(s) in (\"\")"=w2751) -> ("States Out"=w2750:string)  [unwired: 14 in]
      }
      frame "APD: UpdateCtrlVLimit" {
        w2769 = enum16{"Read", "Write"}."Read" ("Operation (Read)")
        # "Template Separator\n(You can make a copy of, or modify, this frame)"
        n1248 = call "APD1FGV.vi"("Error In"=w2766, "Operation (Read)"=w2769) -> ("Error Out"=w2767:errorcluster, "APDClass out"=w2768:refnum<class "APDClass.lvclass">)  [unwired: 8 in]
        n1249 = call "APD2FGV.vi"("Error In"=w2766, "Operation (Read)"=w2769) -> ("Error Out"=w2764:errorcluster, "APDClass out"=w2765:refnum<class "APDClass.lvclass">)  [unwired: 8 in]
        n1250 = call "APD3FGV.vi"("Error In"=w2766, "Operation (Read)"=w2769) -> ("Error Out"=w2762:errorcluster, "APDClass out"=w2763:refnum<class "APDClass.lvclass">)  [unwired: 8 in]
        n1251 = call-dynamic "ReadMaxCtrlV.vi"("error in (no error)"=w2767, "APDClass in"=w2768) -> ("error out"=w2757:errorcluster, "Numeric"=w2760:dbl)  [unwired: 7 in, 1 out]
        n1252 = call-dynamic "ReadMaxCtrlV.vi"("error in (no error)"=w2764, "APDClass in"=w2765) -> ("error out"=w2755:errorcluster, "Numeric"=w2759:dbl)  [unwired: 7 in, 1 out]
        n1253 = call-dynamic "ReadMaxCtrlV.vi"("error in (no error)"=w2762, "APDClass in"=w2763) -> ("error out"=w2753:errorcluster, "Numeric"=w2758:dbl)  [unwired: 7 in, 1 out]
        n1254 = property on="V 1" class="DigNum (strict)"(error in=w2757, "Maximum"=w2760) -> (error out=w2756:errorcluster)  [unwired: 1 in, 1 out]
        n1255 = property on="V 2" class="DigNum (strict)"(error in=w2755, "Maximum"=w2759) -> (error out=w2754:errorcluster)  [unwired: 1 in, 1 out]
        n1256 = property on="V 3" class="DigNum (strict)"(error in=w2753, "Maximum"=w2758) -> (error out=w2752:errorcluster)  [unwired: 1 in, 1 out]
        n1257 = Merge Errors(w2756, w2754, w2752) -> (w2761:errorcluster)
        n1258 = call <vilib>:"Add State(s) to Queue__JKI_lib_State_Machine.vi"("State(s) in (\"\")"=w2773) -> ("States Out"=w2772:string)  [unwired: 14 in]
      }
      frame "APD: GetGainLimits" {
        w2788 = enum16{"Read", "Write"}."Read" ("Operation (Read)")
        # "Template Separator\n(You can make a copy of, or modify, this frame)"
        n1259 = call "APD1FGV.vi"("Error In"=w2787, "Operation (Read)"=w2788) -> ("Error Out"=w2778:errorcluster, "APDClass out"=w2779:refnum<class "APDClass.lvclass">)  [unwired: 8 in]
        n1260 = call "APD2FGV.vi"("Error In"=w2787, "Operation (Read)"=w2788) -> ("Error Out"=w2785:errorcluster, "APDClass out"=w2786:refnum<class "APDClass.lvclass">)  [unwired: 8 in]
        n1261 = call "APD3FGV.vi"("Error In"=w2787, "Operation (Read)"=w2788) -> ("Error Out"=w2783:errorcluster, "APDClass out"=w2784:refnum<class "APDClass.lvclass">)  [unwired: 8 in]
        n1262 = call-dynamic "Read Gain Limits(Log).vi"("error in (no error)"=w2778, "APDClass in"=w2779) -> ("error out"=w2777:errorcluster, "GainLimits(Log)"=w2774:cluster{"GainMax":dbl, "GainMin":dbl})  [unwired: 7 in, 1 out]
        n1263 = call-dynamic "Read Gain Limits(Log).vi"("error in (no error)"=w2785, "APDClass in"=w2786) -> ("error out"=w2781:errorcluster, "GainLimits(Log)"=w2776:cluster{"GainMax":dbl, "GainMin":dbl})  [unwired: 7 in, 1 out]
        n1264 = call-dynamic "Read Gain Limits(Log).vi"("error in (no error)"=w2783, "APDClass in"=w2784) -> ("error out"=w2780:errorcluster, "GainLimits(Log)"=w2775:cluster{"GainMax":dbl, "GainMin":dbl})  [unwired: 7 in, 1 out]
        n1265 = global write "GlobalVariables.vi" "Ch1GainLim(Log)"(w2774) -> ()
        n1266 = global write "GlobalVariables.vi" "Ch2GainLim(Log)"(w2776) -> ()
        n1267 = global write "GlobalVariables.vi" "Ch3GainLim(Log)"(w2775) -> ()
        n1268 = Merge Errors(w2777, w2781, w2780) -> (w2782:errorcluster)
        n1269 = call <vilib>:"Add State(s) to Queue__JKI_lib_State_Machine.vi"("State(s) in (\"\")"=w2792) -> ("States Out"=w2791:string)  [unwired: 14 in]
      }
      frame "---------- TCP ----------" {
        # "Template Separator\n(You can make a copy of, or modify, this frame)"
        n1270 = call <vilib>:"Add State(s) to Queue__JKI_lib_State_Machine.vi"("State(s) in (\"\")"=w2797) -> ("States Out"=w2796:string)  [unwired: 14 in]
      }
      frame "TCP: InitializeNew" {
        # "if unsuccessful and count <10, increament count \nand try again"
        # "Initialize TCP connection to aimging beam computer\n(You can make a copy of, or modify, this frame)"
        n1271 = TCP Create Listener(10:u16 2100 ("port"), 11:"RTLT" ("service name")) -> (0:w2806:errorcluster, 3:w2798:refnum<k5>)  [unwired: 3 in, 1 out]
        n1272 = while {
          tunnel: w2798 -> [w2826]
          tunnel: w2806 -> [w2825]
          tunnel: [w2816] -> w2804
          tunnel: [w2813] -> w2800
          i -> [w2822]
          stop <- w2813 stop-if-true
          n1273 = TCP Wait On Listener(8:w2825, 9:100 ("timeout ms (wait forever: -1)"), 11:w2826) -> (0:w2823:errorcluster, 4:w2820:refnum<k5>)  [unwired: 1 in, 3 out]
          n1274 = Less Or Equal?(x=100, y=w2822) -> (x <= y?=w2819:bool)
          n1275 = case shown="No Error" w2823 {
            selector: w2823 -> [w2836 w2846]
            tunnel: w2820 -> [w2837 _]
            tunnel: [errorcluster {"status"=TRUE, "code"=0, "source"=""} ("No error") w2847] -> w2815
            tunnel: [w2828 FALSE ("TCP connected?")] -> w2816
            frame No Error {
              # "connection is ready, read data"
              n1276 = TCP Read(connection ID=w2837, bytes to read=512, error in (no error)=w2836, 7:T23."CRLF" ("mode (standard)"), 9:5000 ("timeout ms (25000)")) -> (connection ID out=w2830:refnum<k5>, data out=w2832:string, error out=w2829:errorcluster)
              n1277 = Concatenate Strings("alive" ("string"), "\r\n" ("End of Line Constant")) -> (w2833:string)
              n1278 = Equal?(x=w2833, y=w2832) -> (x = y?=w2831:bool)
              n1279 = case shown="False" w2831 {
                tunnel: w2830 -> [_ w2842]
                tunnel: w2829 -> [_ _]
                tunnel: [FALSE ("TCP connected?") TRUE ("TCP connected?")] -> w2828
                frame False {
                }
                frame True {
                  n1280 = call "TcpIDFGV.vi"("action"=enum16{"write", "read"}."write", "connection ID in"=w2842) -> ()  [unwired: 8 in, 2 out]
                }
              }
            }
            frame Error {
              # "connection not ready, keep waiting"
              n1281 = Unbundle By Name(w2846) -> ("code"=w2848:i32)
              n1282 = case shown="56" w2848 {
                tunnel: w2846 -> [w2849 _]
                tunnel: [w2849 w2850] -> w2847
                frame Default {
                }
                frame 56 {
                  w2850 = errorcluster {"status"=FALSE, "code"=0, "source"=""}  # No error
                }
              }
            }
          }
          n1283 = Select(t=errorcluster {"status"=TRUE, "code"=5001, "source"=""} ("error in (no error)"), s=w2819, f=errorcluster {"status"=FALSE, "code"=0, "source"=""} ("error in (no error)")) -> (s? t:f=w2814:errorcluster)
          n1284 = Merge Errors(w2815, w2814) -> (w2813:errorcluster)
        }
        n1285 = Unbundle By Name(w2800) -> ("code"=w2803:i32)
        n1286 = Bundle By Name(cluster=w2805, "System Status.TCP/IP"=w2804, "listener ID"=w2798) -> (w2810:T25)
        n1287 = global write "GlobalVariables.vi" "TCP connected?"(w2804) -> ()
        n1288 = Equal To 0?(x=w2803) -> (x = 0?=w2802:bool)
        n1289 = Select(t=errorcluster {"status"=FALSE, "code"=0, "source"=""} ("error in (no error)"), s=w2802, f=w2800) -> (s? t:f=w2799:errorcluster)
        n1290 = call <vilib>:"Add State(s) to Queue__JKI_lib_State_Machine.vi"("State(s) in (\"\")"=w2812) -> ("States Out"=w2811:string)  [unwired: 14 in]
      }
      frame "TCP: checkSource" {
        # "Check visualization PC video source\n(send !video_source message, listen for response, then parse it to binary mask)"
        n1291 = Unbundle By Name(w2857) -> ("System Status.TCP/IP"=w2860:bool)
        n1292 = case shown="True" w2860 {
          tunnel: w2859 -> [w2865 w2888]
          tunnel: [w2865 w2872] -> w2858
          tunnel: [w2864 w2877] -> w2855
          tunnel: [w2864 w2875] -> w2854
          tunnel: [w2864 w2876] -> w2853
          tunnel: [w2864 w2874] -> w2852
          tunnel: [w2864 w2866] -> w2851
          frame False {
            w2864 = FALSE
          }
          frame True {
            n1293 = call "TcpIDFGV.vi"("Error In"=w2888, "action"=enum16{"write", "read"}."read") -> ("Error Out"=w2885:errorcluster, "connection ID out"=w2887:refnum<k5>)  [unwired: 8 in]
            n1294 = call "TCP_WriteRead.vi"("error in (no error)"=w2885, "data in"="!video_source", "connectin ID in"=w2887) -> ("error out"=w2882:errorcluster, "data out"=w2884:string)  [unwired: 4 in, 1 out]
            n1295 = Scan From String(format string="!video_source:%d", input string=w2884, error in=w2882) -> (error out=w2873:errorcluster, output 1=w2871:i32)  [unwired: 2 in, 2 out]
            n1296 = case shown="5..7, 9..11, 13..15" w2871 {
              tunnel: w2873 -> [_ _ _ _]
              tunnel: [errorcluster {"status"=TRUE, "code"=5007, "source"="Visualization PC"} ("error out") errorcluster {"status"=FALSE, "code"=0, "source"=""} ("error out") errorcluster {"status"=FALSE, "code"=0, "source"=""} ("error out") errorcluster {"status"=FALSE, "code"=0, "source"=""} ("error out")] -> w2872
              tunnel: [FALSE FALSE FALSE TRUE] -> w2866
              frame 0, Default {
                # "No video source available or default"
                n1297 = property on="Video Source" class="RadioBtnsControl (strict)"("DisabledEnum"=T10."Disabled and Grayed Out" ("Disabled")) -> ()  [unwired: 2 in, 2 out]
              }
              frame 1..3 {
                # "one or both camera available"
                n1298 = local write "Video Source"(enum32{"Camera", "FrameGrabber"}."Camera" ("Video Source")) -> ()
                n1299 = property on="Video Source" class="RadioBtnsControl (strict)"("DisabledEnum"=T10."Disabled and Grayed Out" ("Disabled")) -> ()  [unwired: 2 in, 2 out]
              }
              frame 4, 8, 12 {
                # "one or both frame grabber available"
                n1300 = local write "Video Source"(enum32{"Camera", "FrameGrabber"}."FrameGrabber" ("Video Source")) -> ()
                n1301 = property on="Video Source" class="RadioBtnsControl (strict)"("DisabledEnum"=T10."Disabled and Grayed Out" ("Disabled")) -> ()  [unwired: 2 in, 2 out]
              }
              frame 5..7, 9..11, 13..15 {
                n1302 = property on="Video Source" class="RadioBtnsControl (strict)"("DisabledEnum"=T10."Enabled" ("Disabled")) -> ()  [unwired: 2 in, 2 out]
              }
            }
            n1303 = Integer to Fixed-Point Cast(fixed-point type=fxp<+,4,4> 0.0, integer=w2871) -> (fixed-point=w2870:fxp<+,4,4>)
            n1304 = Number To Boolean Array(number=w2870) -> (Boolean array=w2868:bool[])
            n1305 = Reverse 1D Array(array=w2868) -> (reversed array=w2867:bool[])
            n1306 = Index Array(array=w2867, index=0) -> (element=w2877:bool)
            n1307 = Index Array(array=w2867, index=1) -> (element=w2875:bool)
            n1308 = Index Array(array=w2867, index=2) -> (element=w2876:bool)
            n1309 = Index Array(array=w2867, index=3) -> (element=w2874:bool)
          }
        }
        n1310 = Bundle By Name(cluster=w2857, "video source.Main Frame Grabber"=w2855, "video source.Side Frame Grabber"=w2854, "video source.Main Camera"=w2853, "video source.Side Camera"=w2852, "bothVidSourceAvail"=w2851) -> (w2856:T25)
        n1311 = call <vilib>:"Add State(s) to Queue__JKI_lib_State_Machine.vi"("State(s) in (\"\")"=w2863) -> ("States Out"=w2862:string)  [unwired: 14 in]
      }
      frame "TCP: SyncTime" {
        # "Template Separator\n(You can make a copy of, or modify, this frame)"
        n1312 = Unbundle By Name(w2905) -> ("System Status.TCP/IP"=w2904:bool)
        n1313 = case shown="True" w2904 {
          tunnel: w2906 -> [_ w2914]
          frame False {
          }
          frame True {
            n1314 = call "TcpIDFGV.vi"("Error In"=w2914, "action"=enum16{"write", "read"}."read") -> ("Error Out"=w2913:errorcluster, "connection ID out"=w2910:refnum<k5>)  [unwired: 8 in]
            n1315 = call <userlib>:"Tick Count (ms)__ogtk.vi"("error in (no error)"=w2913) -> ("error out"=w2912:errorcluster, "millisecond timer value"=w2911:u32)  [unwired: 9 in]
            n1316 = while {
              tunnel: w2912 -> [w2934]
              tunnel: w2910 -> [w2933]
              tunnel: w2911 -> [w2922]
              stop <- w2917 stop-if-true
              n1317 = Concatenate Strings("latencycheck" ("string"), "\r\n" ("End of Line Constant")) -> (w2929:string)
              n1318 = TCP Read(connection ID=w2933, bytes to read=512, error in (no error)=w2934, 7:T23."CRLF" ("mode (standard)"), 9:2000 ("timeout ms (25000)")) -> (connection ID out=w2926:refnum<k5>, data out=w2924:string, error out=w2916:errorcluster)
              n1319 = Tick Count (ms)() -> (millisecond timer value=w2923:u32)
              n1320 = Subtract(x=w2923, y=w2922) -> (x-y=w2921:u32)
              n1321 = Equal?(x=w2924, y=w2929) -> (x = y?=w2925:bool)
              n1322 = case shown="True" w2925 {
                tunnel: w2926 -> [_ w2947]
                tunnel: w2924 -> [w2939 _]
                tunnel: [w2935 FALSE] -> w2919
                tunnel: w2916 -> [_ w2941]
                frame False {
                  n1323 = Concatenate Strings("synctimer" ("string"), "\r\n" ("End of Line Constant")) -> (w2936:string)
                  n1324 = Equal?(x=w2939, y=w2936) -> (x = y?=w2935:bool)
                  "Sync Success?" <- w2935
                }
                frame True {
                  n1325 = Concatenate Strings("latencycheck:" ("string"), "\r\n" ("End of Line Constant")) -> (w2946:string)
                  n1326 = TCP Write(connection ID=w2947, data in=w2946, error in (no error)=w2941, 9:1000 ("timeout ms (25000)")) -> (error out=w2940:errorcluster)  [unwired: 2 out]
                  n1327 = call <vilib>:"Clear Errors.vi"("error in (no error)"=w2940) -> ()  [unwired: 5 in, 2 out]
                }
              }
              n1328 = Greater?(x=w2921, y=u32 10000 ("x-y")) -> (0:w2918:bool)
              n1329 = Or(x=w2919, y=w2918) -> (x .or. y?=w2917:bool)
            }
          }
        }
        n1330 = call <vilib>:"Add State(s) to Queue__JKI_lib_State_Machine.vi"("State(s) in (\"\")"=w2909) -> ("States Out"=w2908:string)  [unwired: 14 in]
      }
      frame "TCP: SendSettingMacro" {
        # "Template Separator\n(You can make a copy of, or modify, this frame)"
        n1331 = Unbundle By Name(w2951) -> ("System Status.TCP/IP"=w2950:bool)
        n1332 = case shown="True" w2950 {
          tunnel: ["" ("Empty String Constant") "TCP: sendSubjectID\nTCP: sendScaleBarSetting\nTCP: sendScaleMaxMin\nTCP: sendDeconChannel\nTCP: sendANSI\nTCP: sendRadius\nTCP: send3Dsetting\nTCP: sendFirefly\nTCP: sendPentero"] -> w2949
          frame False {
          }
          frame True {
          }
        }
        n1333 = call <vilib>:"Add State(s) to Queue__JKI_lib_State_Machine.vi"("State(s) in Front (\"\")"=w2949, "State(s) in (\"\")"=w2954) -> ("States Out"=w2953:string)  [unwired: 13 in]
      }
      frame "TCP: sendRunNum" {
        # "Send run number to AB PC\n(You can make a copy of, or modify, this frame)"
        n1334 = Unbundle By Name(w2961) -> ("System Status.TCP/IP"=w2958:bool, "IDs.RunID"=w2962:i8)
        n1335 = Increment(x=w2962) -> (x+1=w2957:i8)
        n1336 = case shown="True" w2958 {
          tunnel: w2957 -> [_ w2976]
          tunnel: [w2966 w2968] -> w2960
          tunnel: w2959 -> [w2966 w2967]
          frame False {
          }
          frame True {
            n1337 = Number To Decimal String(number=w2976, width (-)=i16 3) -> (decimal integer string=w2971:string)
            n1338 = call "TcpIDFGV.vi"("Error In"=w2967, "action"=enum16{"write", "read"}."read") -> ("Error Out"=w2969:errorcluster, "connection ID out"=w2973:refnum<k5>)  [unwired: 8 in]
            n1339 = Concatenate Strings("!run:", w2971) -> (w2970:string)
            n1340 = call "TCP_WriteRead.vi"("error in (no error)"=w2969, "data in"=w2970, "connectin ID in"=w2973) -> ("error out"=w2968:errorcluster)  [unwired: 4 in, 2 out]
          }
        }
        n1341 = call <vilib>:"Add State(s) to Queue__JKI_lib_State_Machine.vi"("State(s) in (\"\")"=w2965) -> ("States Out"=w2964:string)  [unwired: 14 in]
      }
      frame "TCP: sendVideoSource" {
        # "Send video source \n(You can make a copy of, or modify, this frame)"
        n1342 = Unbundle By Name(w2978) -> ("System Status.TCP/IP"=w2977:bool)
        n1343 = case shown="True" w2977 {
          tunnel: [w2984 w2986] -> w2980
          tunnel: w2979 -> [w2984 w2985]
          frame False {
          }
          frame True {
            n1344 = case shown="\"Camera\", Default" "Video Source" {
              tunnel: [0 1] -> w2991
              frame "Camera", Default {
              }
              frame "FrameGrabber" {
              }
            }
            n1345 = call "TcpIDFGV.vi"("Error In"=w2985, "action"=enum16{"write", "read"}."read") -> ("Error Out"=w2987:errorcluster, "connection ID out"=w2993:refnum<k5>)  [unwired: 8 in]
            n1346 = Number To Decimal String(number=w2991) -> (decimal integer string=w2989:string)  [unwired: 1 in]
            n1347 = Concatenate Strings("!invivo:" ("data in"), w2989) -> (w2988:string)
            n1348 = call "TCP_WriteRead.vi"("error in (no error)"=w2987, "data in"=w2988, "connectin ID in"=w2993) -> ("error out"=w2986:errorcluster)  [unwired: 4 in, 2 out]
          }
        }
        n1349 = call <vilib>:"Add State(s) to Queue__JKI_lib_State_Machine.vi"("State(s) in (\"\")"=w2983) -> ("States Out"=w2982:string)  [unwired: 14 in]
      }
      frame "TCP: startRun" {
        # "Template Separator\n(You can make a copy of, or modify, this frame)"
        n1350 = Unbundle By Name(w2998) -> ("System Status.TCP/IP"=w2997:bool)
        n1351 = case shown="True" w2997 {
          tunnel: [w3004 w3006] -> w3000
          tunnel: w2999 -> [w3004 w3005]
          frame False {
          }
          frame True {
            n1352 = call "TcpIDFGV.vi"("Error In"=w3005, "action"=enum16{"write", "read"}."read") -> ("Error Out"=w3007:errorcluster, "connection ID out"=w3008:refnum<k5>)  [unwired: 8 in]
            n1353 = call "TCP_WriteRead.vi"("error in (no error)"=w3007, "data in"="!acquire:1", "connectin ID in"=w3008) -> ("error out"=w3006:errorcluster)  [unwired: 4 in, 2 out]
          }
        }
        n1354 = call <vilib>:"Add State(s) to Queue__JKI_lib_State_Machine.vi"("State(s) in (\"\")"=w3003) -> ("States Out"=w3002:string)  [unwired: 14 in]
      }
      frame "TCP: stopRun" {
        # "Send stop run to AB PC\n(You can make a copy of, or modify, this frame)"
        n1355 = Unbundle By Name(w3012) -> ("System Status.TCP/IP"=w3011:bool)
        n1356 = case shown="True" w3011 {
          tunnel: [w3018 w3020] -> w3014
          tunnel: w3013 -> [w3018 w3019]
          frame False {
            # "if not connected, do nothing"
          }
          frame True {
            # "If TCP connected, send stop run"
            n1357 = call "TcpIDFGV.vi"("Error In"=w3019, "action"=enum16{"write", "read"}."read") -> ("Error Out"=w3021:errorcluster, "connection ID out"=w3023:refnum<k5>)  [unwired: 8 in]
            n1358 = call "TCP_WriteRead.vi"("error in (no error)"=w3021, "data in"="!acquire:0", "connectin ID in"=w3023) -> ("error out"=w3020:errorcluster)  [unwired: 4 in, 2 out]
          }
        }
        n1359 = call <vilib>:"Add State(s) to Queue__JKI_lib_State_Machine.vi"("State(s) in (\"\")"=w3017) -> ("States Out"=w3016:string)  [unwired: 14 in]
      }
      frame "TCP: CheckConnection" {
        # "Check TCP/IP connection statuse\n(If connection is lost, throw error)"
        n1360 = Unbundle By Name(w3026) -> ("System Status.TCP/IP"=w3025:bool)
        n1361 = case shown="False" w3025 {
          frame False {
          }
          frame True {
            # "If TCP/IP is true check, otherwise skip"
          }
        }
        n1362 = call <vilib>:"Add State(s) to Queue__JKI_lib_State_Machine.vi"("State(s) in (\"\")"=w3030) -> ("States Out"=w3029:string)  [unwired: 14 in]
      }
      frame "TCP: sendSubjectID" {
        # "Send subject ID"
        n1363 = Unbundle By Name(w3032) -> ("System Status.TCP/IP"=w3031:bool, "CaseID"=w3035:string)
        n1364 = case shown="True" w3031 {
          tunnel: w3035 -> [_ w3046]
          tunnel: [w3039 w3041] -> w3034
          tunnel: w3033 -> [w3039 w3040]
          frame False {
          }
          frame True {
            n1365 = call "TcpIDFGV.vi"("Error In"=w3040, "action"=enum16{"write", "read"}."read") -> ("Error Out"=w3042:errorcluster, "connection ID out"=w3044:refnum<k5>)  [unwired: 8 in]
            n1366 = Concatenate Strings("!subject:", w3046) -> (w3043:string)
            n1367 = call "TCP_WriteRead.vi"("error in (no error)"=w3042, "data in"=w3043, "connectin ID in"=w3044) -> ("error out"=w3041:errorcluster)  [unwired: 4 in, 2 out]
          }
        }
        n1368 = call <vilib>:"Add State(s) to Queue__JKI_lib_State_Machine.vi"("State(s) in (\"\")"=w3038) -> ("States Out"=w3037:string)  [unwired: 14 in]
      }
      frame "TCP: sendScaleBarSetting" {
        # "Template Separator\n(You can make a copy of, or modify, this frame)"
        n1369 = Unbundle By Name(w3050) -> ("System Status.TCP/IP"=w3048:bool, "VideoConfig.Scale Bar"=w3049:bool)
        n1370 = case shown="True" w3048 {
          tunnel: [w3056 w3065] -> w3052
          tunnel: w3051 -> [w3056 w3064]
          tunnel: w3049 -> [_ w3063]
          frame False {
          }
          frame True {
            n1371 = Boolean To (0,1)(Boolean=w3063) -> (0, 1=w3062:i16)
            n1372 = call "TcpIDFGV.vi"("Error In"=w3064, "action"=enum16{"write", "read"}."read") -> ("Error Out"=w3066:errorcluster, "connection ID out"=w3067:refnum<k5>)  [unwired: 8 in]
            n1373 = Number To Fractional String(number=w3062, width (-)=i16 1, precision (6)=i16 0) -> (F-format string=w3060:string)  [unwired: 1 in]
            n1374 = Concatenate Strings("!autocolor:" ("data in"), w3060) -> (w3058:string)
            n1375 = call "TCP_WriteRead.vi"("error in (no error)"=w3066, "data in"=w3058, "connectin ID in"=w3067) -> ("error out"=w3065:errorcluster)  [unwired: 4 in, 2 out]
          }
        }
        n1376 = call <vilib>:"Add State(s) to Queue__JKI_lib_State_Machine.vi"("State(s) in (\"\")"=w3055) -> ("States Out"=w3054:string)  [unwired: 14 in]
      }
      frame "TCP: sendScaleMaxMin" {
        # "Send scale bar max and min to AB PC\n(You can make a copy of, or modify, this frame)"
        n1377 = Unbundle By Name(w3072) -> ("System Status.TCP/IP"=w3069:bool, "VideoConfig.Scale Low"=w3071:dbl, "VideoConfig.Scale High"=w3070:dbl)
        n1378 = case shown="True" w3069 {
          tunnel: [w3078 w3091] -> w3074
          tunnel: w3073 -> [w3078 w3090]
          tunnel: w3071 -> [_ w3089]
          tunnel: w3070 -> [_ w3080]
          frame False {
          }
          frame True {
            n1379 = call "TcpIDFGV.vi"("Error In"=w3090, "action"=enum16{"write", "read"}."read") -> ("Error Out"=w3092:errorcluster, "connection ID out"=w3093:refnum<k5>)  [unwired: 8 in]
            n1380 = Number To Fractional String(number=w3089, width (-)=i16 4, precision (6)=i16 2) -> (F-format string=w3085:string)  [unwired: 1 in]
            n1381 = Number To Fractional String(number=w3080, width (-)=i16 4, precision (6)=i16 2) -> (F-format string=w3081:string)  [unwired: 1 in]
            n1382 = Concatenate Strings("!color:" ("string"), w3085, ";" ("string"), w3081) -> (w3079:string)
            n1383 = call "TCP_WriteRead.vi"("error in (no error)"=w3092, "data in"=w3079, "connectin ID in"=w3093) -> ("error out"=w3091:errorcluster)  [unwired: 4 in, 2 out]
          }
        }
        n1384 = call <vilib>:"Add State(s) to Queue__JKI_lib_State_Machine.vi"("State(s) in (\"\")"=w3077) -> ("States Out"=w3076:string)  [unwired: 14 in]
      }
      frame "TCP: sendDeconChannel" {
        # "Send Decon channel\n(You can make a copy of, or modify, this frame)"
        n1385 = Unbundle By Name(w3096) -> ("System Status.TCP/IP"=w3095:bool)
        n1386 = case shown="True" w3095 {
          tunnel: [w3102 w3107] -> w3098
          tunnel: w3097 -> [w3102 w3106]
          frame False {
          }
          frame True {
            n1387 = local read "Radio Buttons"() -> (w3105:enum32{"No Selection", "Ch1", "Ch2", "Ch3"})
            n1388 = Increment(x=w3105) -> (x+1=w3104:enum32{"No Selection", "Ch1", "Ch2", "Ch3"})
            n1389 = Number To Decimal String(number=w3104) -> (decimal integer string=w3103:string)  [unwired: 1 in]
            n1390 = call "TcpIDFGV.vi"("Error In"=w3106, "action"=enum16{"write", "read"}."read") -> ("Error Out"=w3108:errorcluster, "connection ID out"=w3111:refnum<k5>)  [unwired: 8 in]
            n1391 = Concatenate Strings("!channel:", w3103) -> (w3109:string)
            n1392 = call "TCP_WriteRead.vi"("error in (no error)"=w3108, "data in"=w3109, "connectin ID in"=w3111) -> ("error out"=w3107:errorcluster)  [unwired: 4 in, 2 out]
          }
        }
        n1393 = call <vilib>:"Add State(s) to Queue__JKI_lib_State_Machine.vi"("State(s) in (\"\")"=w3101) -> ("States Out"=w3100:string)  [unwired: 14 in]
      }
      frame "TCP: sendANSI" {
        # "Template Separator\n(You can make a copy of, or modify, this frame)"
        n1394 = Unbundle By Name(w3115) -> ("System Status.TCP/IP"=w3113:bool, "VideoConfig.ANSI"=w3114:dbl)
        n1395 = case shown="True" w3113 {
          tunnel: [w3121 w3127] -> w3117
          tunnel: w3116 -> [w3121 w3126]
          tunnel: w3114 -> [_ w3125]
          frame False {
          }
          frame True {
            n1396 = Number To Fractional String(number=w3125) -> (F-format string=w3123:string)  [unwired: 3 in]
            n1397 = call "TcpIDFGV.vi"("Error In"=w3126, "action"=enum16{"write", "read"}."read") -> ("Error Out"=w3128:errorcluster, "connection ID out"=w3129:refnum<k5>)  [unwired: 8 in]
            n1398 = Concatenate Strings("!ansi:" ("data in"), w3123) -> (w3122:string)
            n1399 = call "TCP_WriteRead.vi"("error in (no error)"=w3128, "data in"=w3122, "connectin ID in"=w3129) -> ("error out"=w3127:errorcluster)  [unwired: 4 in, 2 out]
          }
        }
        n1400 = call <vilib>:"Add State(s) to Queue__JKI_lib_State_Machine.vi"("State(s) in (\"\")"=w3120) -> ("States Out"=w3119:string)  [unwired: 14 in]
      }
      frame "TCP: sendRadius" {
        # "Send drawing radius to AB PC\n(You can make a copy of, or modify, this frame)"
        n1401 = Unbundle By Name(w3133) -> ("System Status.TCP/IP"=w3131:bool, "VideoConfig.Radius"=w3132:dbl)
        n1402 = case shown="True" w3131 {
          tunnel: [w3139 w3145] -> w3135
          tunnel: w3134 -> [w3139 w3144]
          tunnel: w3132 -> [_ w3143]
          frame False {
          }
          frame True {
            n1403 = Number To Fractional String(number=w3143) -> (F-format string=w3142:string)  [unwired: 3 in]
            n1404 = Concatenate Strings("!radius:" ("data in"), w3142) -> (w3140:string)
            n1405 = call "TcpIDFGV.vi"("Error In"=w3144, "action"=enum16{"write", "read"}."read") -> ("Error Out"=w3146:errorcluster, "connection ID out"=w3147:refnum<k5>)  [unwired: 8 in]
            n1406 = call "TCP_WriteRead.vi"("error in (no error)"=w3146, "data in"=w3140, "connectin ID in"=w3147) -> ("error out"=w3145:errorcluster)  [unwired: 4 in, 2 out]
          }
        }
        n1407 = call <vilib>:"Add State(s) to Queue__JKI_lib_State_Machine.vi"("State(s) in (\"\")"=w3138) -> ("States Out"=w3137:string)  [unwired: 14 in]
      }
      frame "TCP: send3Dsetting" {
        # "Send 3D setting to AB computer\n(You can make a copy of, or modify, this frame)"
        n1408 = Unbundle By Name(w3151) -> ("System Status.TCP/IP"=w3149:bool, "VideoConfig.3D?"=w3150:bool)
        n1409 = case shown="True" w3149 {
          tunnel: [w3157 w3164] -> w3153
          tunnel: w3152 -> [w3157 w3163]
          tunnel: w3150 -> [_ w3162]
          frame False {
          }
          frame True {
            n1410 = Boolean To (0,1)(Boolean=w3162) -> (0, 1=w3161:i16)
            n1411 = Number To Fractional String(number=w3161) -> (F-format string=w3160:string)  [unwired: 3 in]
            n1412 = call "TcpIDFGV.vi"("Error In"=w3163, "action"=enum16{"write", "read"}."read") -> ("Error Out"=w3165:errorcluster, "connection ID out"=w3166:refnum<k5>)  [unwired: 8 in]
            n1413 = Concatenate Strings("!3dset:" ("data in"), w3160) -> (w3158:string)
            n1414 = call "TCP_WriteRead.vi"("error in (no error)"=w3165, "data in"=w3158, "connectin ID in"=w3166) -> ("error out"=w3164:errorcluster)  [unwired: 4 in, 2 out]
          }
        }
        n1415 = call <vilib>:"Add State(s) to Queue__JKI_lib_State_Machine.vi"("State(s) in (\"\")"=w3156) -> ("States Out"=w3155:string)  [unwired: 14 in]
      }
      frame "TCP: sendFirefly" {
        # "Template Separator\n(You can make a copy of, or modify, this frame)"
        n1416 = Unbundle By Name(w3169) -> ("System Status.TCP/IP"=w3168:bool)
        n1417 = case shown="False" w3168 {
          tunnel: [w3175 w3177] -> w3171
          tunnel: w3170 -> [w3175 w3176]
          frame False {
          }
          frame True {
            n1418 = call "TcpIDFGV.vi"("Error In"=w3176, "action"=enum16{"write", "read"}."read") -> ("Error Out"=w3178:errorcluster, "connection ID out"=w3180:refnum<k5>)  [unwired: 8 in]
            n1419 = call "TCP_WriteRead.vi"("error in (no error)"=w3178, "data in"="!firefly:0", "connectin ID in"=w3180) -> ("error out"=w3177:errorcluster)  [unwired: 4 in, 2 out]
          }
        }
        n1420 = call <vilib>:"Add State(s) to Queue__JKI_lib_State_Machine.vi"("State(s) in (\"\")"=w3174) -> ("States Out"=w3173:string)  [unwired: 14 in]
      }
      frame "TCP: sendPentero" {
        # "Send Pentero setting to AB computer\n(You can make a copy of, or modify, this frame)"
        n1421 = Unbundle By Name(w3183) -> ("System Status.TCP/IP"=w3182:bool)
        n1422 = case shown="True" w3182 {
          tunnel: [w3189 w3191] -> w3185
          tunnel: w3184 -> [w3189 w3190]
          frame False {
          }
          frame True {
            n1423 = call "TcpIDFGV.vi"("Error In"=w3190, "action"=enum16{"write", "read"}."read") -> ("Error Out"=w3192:errorcluster, "connection ID out"=w3194:refnum<k5>)  [unwired: 8 in]
            n1424 = call "TCP_WriteRead.vi"("error in (no error)"=w3192, "data in"="!pentero:0", "connectin ID in"=w3194) -> ("error out"=w3191:errorcluster)  [unwired: 4 in, 2 out]
          }
        }
        n1425 = call <vilib>:"Add State(s) to Queue__JKI_lib_State_Machine.vi"("State(s) in (\"\")"=w3188) -> ("States Out"=w3187:string)  [unwired: 14 in]
      }
      frame "TCP: sendChannel" {
        # "Send DeCon Channel to AB computer\n()"
        n1426 = Unbundle By Name(w3197) -> ("System Status.TCP/IP"=w3196:bool)
        n1427 = case shown="True" w3196 {
          tunnel: [w3203 w3207] -> w3199
          tunnel: w3198 -> [w3203 w3206]
          frame False {
          }
          frame True {
            n1428 = local read "Radio Buttons"() -> (w3205:enum32{"No Selection", "Ch1", "Ch2", "Ch3"})
            n1429 = case shown="\"No Selection\", Default" w3205 {
              tunnel: ["" ("data in") "!channel:1" ("data in") "!channel:2" ("data in") "!channel:3" ("data in")] -> w3204
              frame "No Selection", Default {
              }
              frame "Ch1" {
              }
              frame "Ch2" {
              }
              frame "Ch3" {
              }
            }
            n1430 = call "TcpIDFGV.vi"("Error In"=w3206, "action"=enum16{"write", "read"}."read") -> ("Error Out"=w3208:errorcluster, "connection ID out"=w3209:refnum<k5>)  [unwired: 8 in]
            n1431 = call "TCP_WriteRead.vi"("error in (no error)"=w3208, "data in"=w3204, "connectin ID in"=w3209) -> ("error out"=w3207:errorcluster)  [unwired: 4 in, 2 out]
          }
        }
        n1432 = call <vilib>:"Add State(s) to Queue__JKI_lib_State_Machine.vi"("State(s) in (\"\")"=w3202) -> ("States Out"=w3201:string)  [unwired: 14 in]
      }
      frame "TCP: startCam" {
        # "Send Pentero setting to AB computer\n(You can make a copy of, or modify, this frame)"
        n1433 = Unbundle By Name(w3216) -> ("System Status.TCP/IP"=w3215:bool)
        n1434 = case shown="True" w3215 {
          tunnel: [w3222 w3224] -> w3218
          tunnel: w3217 -> [w3222 w3223]
          frame False {
          }
          frame True {
            n1435 = call "TcpIDFGV.vi"("Error In"=w3223, "action"=enum16{"write", "read"}."read") -> ("Error Out"=w3225:errorcluster, "connection ID out"=w3227:refnum<k5>)  [unwired: 8 in]
            n1436 = call "TCP_WriteRead.vi"("error in (no error)"=w3225, "data in"="!focus:1", "connectin ID in"=w3227) -> ("error out"=w3224:errorcluster)  [unwired: 4 in, 2 out]
          }
        }
        n1437 = call <vilib>:"Add State(s) to Queue__JKI_lib_State_Machine.vi"("State(s) in (\"\")"=w3221) -> ("States Out"=w3220:string)  [unwired: 14 in]
      }
      frame "TCP: stopCam" {
        # "Send Pentero setting to AB computer\n(You can make a copy of, or modify, this frame)"
        n1438 = Unbundle By Name(w3230) -> ("System Status.TCP/IP"=w3229:bool)
        n1439 = case shown="True" w3229 {
          tunnel: [w3236 w3238] -> w3232
          tunnel: w3231 -> [w3236 w3237]
          frame False {
          }
          frame True {
            n1440 = call "TcpIDFGV.vi"("Error In"=w3237, "action"=enum16{"write", "read"}."read") -> ("Error Out"=w3239:errorcluster, "connection ID out"=w3241:refnum<k5>)  [unwired: 8 in]
            n1441 = call "TCP_WriteRead.vi"("error in (no error)"=w3239, "data in"="!focus:0", "connectin ID in"=w3241) -> ("error out"=w3238:errorcluster)  [unwired: 4 in, 2 out]
          }
        }
        n1442 = call <vilib>:"Add State(s) to Queue__JKI_lib_State_Machine.vi"("State(s) in (\"\")"=w3235) -> ("States Out"=w3234:string)  [unwired: 14 in]
      }
      frame "TCP: Close" {
        # "Close TCP connection\n()"
        n1443 = Unbundle By Name(w3245) -> ("System Status.TCP/IP"=w3243:bool)
        n1444 = case shown="True" w3243 {
          tunnel: [w3251 w3253] -> w3246
          tunnel: w3244 -> [w3251 w3252]
          frame False {
          }
          frame True {
            n1445 = call "TcpIDFGV.vi"("Error In"=w3252, "action"=enum16{"write", "read"}."read") -> ("Error Out"=w3255:errorcluster, "connection ID out"=w3256:refnum<k5>)  [unwired: 8 in]
            n1446 = TCP Close Connection(connection ID=w3256, error in (no error)=w3255) -> (error out=w3253:errorcluster)  [unwired: 1 in, 1 out]
          }
        }
        n1447 = case shown="Error .." w3246 {
          tunnel: [w3259 w3260] -> w3247
          tunnel: w3245 -> [w3258 w3260]
          frame No Error {
            w3257 = FALSE ("System Status.TCP/IP")
            n1448 = Bundle By Name(cluster=w3258, "System Status.TCP/IP"=w3257) -> (w3259:T25)
            n1449 = global write "GlobalVariables.vi" "TCP connected?"(w3257) -> ()
          }
          frame Error {
          }
        }
        n1450 = call <vilib>:"Add State(s) to Queue__JKI_lib_State_Machine.vi"("State(s) in (\"\")"=w3250) -> ("States Out"=w3249:string)  [unwired: 14 in]
      }
      frame "---------- PID ----------" {
        # "Template Separator\n(You can make a copy of, or modify, this frame)"
        n1451 = call <vilib>:"Add State(s) to Queue__JKI_lib_State_Machine.vi"("State(s) in (\"\")"=w3265) -> ("States Out"=w3264:string)  [unwired: 14 in]
      }
      frame "PID: loadPID" {
        # "Template Separator\n(You can make a copy of, or modify, this frame)"
        n1452 = call "readPIDSetting.vi"("Error In"=w3269) -> ("Error Out"=w3270:errorcluster, "Ch3 PID out"=w3266:T8, "Ch2 PID out"=w3267:T8, "Ch1 PID out"=w3268:T8)  [unwired: 7 in]
        n1453 = local write "Ch3 PID gains"(w3266) -> ()
        n1454 = local write "Ch1 PID gains"(w3268) -> ()
        n1455 = local write "Ch2 PID gains"(w3267) -> ()
        n1456 = call <vilib>:"Add State(s) to Queue__JKI_lib_State_Machine.vi"("State(s) in (\"\")"=w3274) -> ("States Out"=w3273:string)  [unwired: 14 in]
      }
      frame "---------- Temp ----------" {
        # "Template Separator\n(You can make a copy of, or modify, this frame)"
        n1457 = call <vilib>:"Add State(s) to Queue__JKI_lib_State_Machine.vi"("State(s) in (\"\")"=w3279) -> ("States Out"=w3278:string)  [unwired: 14 in]
      }
    }
    n1458 = Not(x=w190) -> (.not. x?=w189:bool)
    n1459 = local write "ML?"(w189) -> ()
    "ML?" <- TRUE ("main loop running?")
  }
  n1460 = while {
    tunnel: w18 -> [w3315]
    tunnel: w17 -> [w3310]
    tunnel: [w3309] -> w16
    tunnel: w12 -> [w3302]
    tunnel: [w3301] -> w15
    shift-right: [w3293] -> _
    shift-left: _ -> [w3294]
    i -> [w3308]
    stop <- w3289 stop-if-true
    # "Read data from notifier and deconvolve it and send to Aiming Beam computer"
    n1461 = Wait on Notification(notifier=w3315, ignore previous (F)=TRUE) -> (notification=w3314:T13, error out=w3305:errorcluster)  [unwired: 2 in, 2 out]
    n1462 = Wait Until Next ms Multiple(millisecond multiple=u32 20) -> ()  [unwired: 1 out]
    n1463 = Unbundle(w3314) -> ("CH1&2"=w3313:dbl[][], "CH3"=w3312:dbl[][], "V cluster"=w3297:cluster{"V1":dbl, "V2":dbl, "V3":dbl})  [unwired: 1 out]
    n1464 = call <vilib>:"High Resolution Relative Seconds.vi"() -> ("relative seconds"=w3293:dbl)
    n1465 = call "SeperateChanData.vi"("Input (Ch1&2)"=w3313) -> ("Ch1"=w3285:dbl[][], "Ch2"=w3283:dbl[][])
    n1466 = call "SeperateChanData.vi"("Input (Ch1&2)"=w3312) -> ("Ch1"=w3281:dbl[][])  [unwired: 1 out]
    n1467 = Subtract(x=w3293, y=w3294) -> (x-y=w3296:dbl)
    n1468 = call "AvgArrayTimeCritical.vi"("2D array"=w3285) -> ("1D Avg"=w3284:dbl[])  [unwired: 10 in]
    n1469 = call "AvgArrayTimeCritical.vi"("2D array"=w3283) -> ("1D Avg"=w3282:dbl[])  [unwired: 10 in]
    n1470 = call "AvgArrayTimeCritical.vi"("2D array"=w3281) -> ("1D Avg"=w3280:dbl[])  [unwired: 10 in]
    n1471 = Multiply(x=w3296, y=1000.0) -> (x*y=→"Decon Loop timing (ms)":dbl)
    n1472 = case shown="\"Ch1\"" "Radio Buttons" {
      selector: "Radio Buttons" -> [_ w3324 w3336 w3349]
      tunnel: w3284 -> [w3323 w3332 w3342 w3354]
      tunnel: w3282 -> [w3321 w3329 w3344 w3352]
      tunnel: w3280 -> [w3319 w3327 w3339 w3357]
      tunnel: FALSE -> [_ w3335 w3347 w3359]
      tunnel: w3305 -> [w3317 w3334 w3346 w3348]
      tunnel: [w3317 w3333 w3345 w3358] -> w3289
      tunnel: [w3322 w3330 w3340 w3353] -> w3300
      tunnel: [w3320 w3328 w3341 w3351] -> w3299
      tunnel: [w3318 w3326 w3338 w3355] -> w3298
      tunnel: [0.0 ("lifetime (ns)") w3325 w3337 w3350] -> w3304
      frame "No Selection", Default {
        n1473 = Build Array(w3323) -> (w3322:dbl[][])
        n1474 = Build Array(w3321) -> (w3320:dbl[][])
        n1475 = Build Array(w3319) -> (w3318:dbl[][])
      }
      frame "Ch1" {
        n1476 = call "Deconvolution.vi"("DeconChannel"=w3324, "iRF align"=w3335, "error in (no error)"=w3334, "Waveform"=w3332) -> ("error out"=w3333:errorcluster, "lifetime (ns)"=w3325:dbl, "Fitting"=w3331:dbl[])  [unwired: 5 in]
        "Lifetime 1" <- w3325
        n1477 = Build Array(w3332, w3331) -> (w3330:dbl[][])
        n1478 = Build Array(w3329) -> (w3328:dbl[][])
        n1479 = Build Array(w3327) -> (w3326:dbl[][])
      }
      frame "Ch2" {
        n1480 = call "Deconvolution.vi"("DeconChannel"=w3336, "iRF align"=w3347, "error in (no error)"=w3346, "Waveform"=w3344) -> ("error out"=w3345:errorcluster, "lifetime (ns)"=w3337:dbl, "Fitting"=w3343:dbl[])  [unwired: 5 in]
        "Lifetime 2" <- w3337
        n1481 = Build Array(w3342) -> (w3340:dbl[][])
        n1482 = Build Array(w3344, w3343) -> (w3341:dbl[][])
        n1483 = Build Array(w3339) -> (w3338:dbl[][])
      }
      frame "Ch3" {
        n1484 = call "Deconvolution.vi"("DeconChannel"=w3349, "iRF align"=w3359, "error in (no error)"=w3348, "Waveform"=w3357) -> ("error out"=w3358:errorcluster, "lifetime (ns)"=w3350:dbl, "Fitting"=w3356:dbl[])  [unwired: 5 in]
        "Lifetime 3" <- w3350
        n1485 = Build Array(w3354) -> (w3353:dbl[][])
        n1486 = Build Array(w3352) -> (w3351:dbl[][])
        n1487 = Build Array(w3357, w3356) -> (w3355:dbl[][])
      }
    }
    n1488 = Bundle(w3300, w3299, w3298, "V cluster"=w3297) -> (w3303:T50)  [unwired: 1 in]
    n1489 = Bundle(w3308, "lifetime (ns)"=w3304) -> (w3311:cluster{i32, "lifetime (ns)":dbl})  [unwired: 1 in]
    n1490 = Send Notification(notification=w3303, notifier=w3302, error in (no error)=w3289) -> (notifier out=w3301:refnum<notifier>, error out=w3288:errorcluster)
    n1491 = Send Notification(notification=w3311, notifier=w3310, error in (no error)=w3289) -> (notifier out=w3309:refnum<notifier>, error out=w3287:errorcluster)
    n1492 = Merge Errors(w3288, w3287) -> (→"decon error out":errorcluster)
  }
  n1493 = while {
    tunnel: w17 -> [w3370]
    shift-right: [w3363] -> _
    shift-left: u32 0 -> [w3364]
    stop <- w3361 stop-if-true
    # "Send data to AB computer here"
    # "if TCP ip is not open loop will run once and stop. To re-establish connection and start this loop. Reboot softwrae."
    # "Data communication loop"
    n1494 = Tick Count (ms)() -> (millisecond timer value=w3363:u32)
    n1495 = Wait on Notification(notifier=w3370, ignore previous (F)=TRUE) -> (notification=w3368:cluster{"idx":i32, "lifetime":dbl}, error out=w3362:errorcluster)  [unwired: 2 in, 2 out]
    n1496 = Unbundle(w3368) -> ("idx"=w3367:i32, "lifetime"=w3366:dbl)
    n1497 = global read "GlobalVariables.vi" "TCP connected?"() -> (w3360:bool)
    n1498 = Subtract(x=w3363, y=w3364) -> (x-y=→"Communication loop(ms)":u32)
    n1499 = case shown="True" w3360 {
      tunnel: w3367 -> [_ w3379]
      tunnel: w3366 -> [_ w3378]
      tunnel: w3362 -> [w3371 w3375]
      tunnel: [w3371 w3372] -> w3361
      frame False {
      }
      frame True {
        n1500 = Number To Decimal String(number=w3379) -> (decimal integer string=w3387:string)  [unwired: 1 in]
        n1501 = call "TcpIDFGV.vi"("Error In"=w3375, "action"=enum16{"write", "read"}."read") -> ("Error Out"=w3374:errorcluster, "connection ID out"=w3385:refnum<k5>)  [unwired: 8 in]
        n1502 = Concatenate Strings("!idx:", w3387) -> (w3388:string)
        n1503 = call "TCP_WriteRead.vi"("error in (no error)"=w3374, "data in"=w3388, "connectin ID in"=w3385) -> ("error out"=w3373:errorcluster, "connectin ID out"=w3386:refnum<k5>)  [unwired: 4 in, 1 out]
        n1504 = Number To Fractional String(number=w3378, precision (6)=i16 2) -> (F-format string=w3377:string)  [unwired: 2 in]
        n1505 = Concatenate Strings("!lifetime:", w3377) -> (w3384:string)
        n1506 = call "TCP_WriteRead.vi"("error in (no error)"=w3373, "data in"=w3384, "connectin ID in"=w3386) -> ("error out"=w3372:errorcluster, "data out"=→"data out(communcation loop)":string)  [unwired: 4 in, 1 out]
      }
    }
  }
  n1507 = while {
    tunnel: w12 -> [w3399]
    shift-right: [w3390] -> _
    shift-left: w14 -> [w3397]
    shift-right: [w3392] -> _
    shift-left: w14 -> [w3391]
    i -> [w3393]
    stop <- w3394 stop-if-true
    # "Data display loop(30Hz)"
    n1508 = Wait on Notification(notifier=w3399, ignore previous (F)=FALSE) -> (notification=w3395:T12, error out=w3394:errorcluster)  [unwired: 2 in, 2 out]
    n1509 = Wait Until Next ms Multiple(millisecond multiple=u32 33) -> ()  [unwired: 1 out]
    n1510 = Tick Count (ms)() -> (millisecond timer value=w3390:u32)
    n1511 = Subtract(x=w3390, y=w3397) -> (x-y=→"display loop timing(ms)":u32)
    n1512 = case shown="No Error" w3394 {
      tunnel: w3395 -> [w3463 _]
      tunnel: w3391 -> [w3422 w3515]
      tunnel: [w3424 w3515] -> w3392
      tunnel: w3390 -> [w3421 _]
      frame No Error {
        w3460 = 0 ("index (row)")
        n1513 = Subtract(x=w3421, y=w3422) -> (x-y=w3423:u32)
        n1514 = Unbundle(w3463) -> ("CH1"=w3456:dbl[][], "CH2"=w3454:dbl[][], "CH3"=w3451:dbl[][], "Gain cluster"=w3428:cluster{"V1":dbl, "V2":dbl, "V3":dbl})
        n1515 = Index Array(array=w3456, index (row)=w3460) -> (element=w3430:dbl[])  [unwired: 1 in]
        n1516 = Index Array(array=w3454, index (row)=w3460) -> (element=w3427:dbl[])  [unwired: 1 in]
        n1517 = Index Array(array=w3451, index (row)=w3460) -> (element=w3429:dbl[])  [unwired: 1 in]
        n1518 = Unbundle By Name(w3428) -> ("V1"=w3417:dbl, "V2"=w3415:dbl, "V3"=w3413:dbl)
        n1519 = Greater?(x=w3423, y=u32 200) -> (0:w3425:bool)
        n1520 = call "CtrlVtoGain.vi"("CtrlV(V)"=w3417, "Channel"=enum16{"Ch1", "Ch2", "Ch3"}."Ch1") -> ("Gain"=w3411:dbl)  [unwired: 8 in, 1 out]
        n1521 = call "RemoveDCBG.vi"("Channel"=enum16{"DC Only", "Ch1", "Ch2", "Ch3"}."Ch1", "WF in"=w3430) -> ("DC"=w3458:dbl, "WF out"=w3418:dbl[])  [unwired: 7 in, 1 out]
        n1522 = call "RemoveDCBG.vi"("Channel"=enum16{"DC Only", "Ch1", "Ch2", "Ch3"}."Ch2", "WF in"=w3427) -> ("DC"=w3453:dbl, "WF out"=w3419:dbl[])  [unwired: 7 in, 1 out]
        n1523 = call "CtrlVtoGain.vi"("CtrlV(V)"=w3415, "Channel"=enum16{"Ch1", "Ch2", "Ch3"}."Ch2") -> ("Gain"=w3406:dbl)  [unwired: 8 in, 1 out]
        n1524 = call "RemoveDCBG.vi"("Channel"=enum16{"DC Only", "Ch1", "Ch2", "Ch3"}."Ch3", "WF in"=w3429) -> ("DC"=w3450:dbl, "WF out"=w3420:dbl[])  [unwired: 7 in, 1 out]
        n1525 = call "CtrlVtoGain.vi"("CtrlV(V)"=w3413, "Channel"=enum16{"Ch1", "Ch2", "Ch3"}."Ch3") -> ("Gain"=w3402:dbl)  [unwired: 8 in, 1 out]
        n1526 = case shown="True" w3425 {
          tunnel: w3418 -> [_ w3478]
          tunnel: w3419 -> [_ w3482]
          tunnel: w3420 -> [_ w3481]
          tunnel: w3421 -> [_ w3498]
          tunnel: [w3470 w3498] -> w3424
          tunnel: w3422 -> [w3470 _]
          tunnel: w3411 -> [_ w3473]
          tunnel: w3406 -> [_ w3472]
          tunnel: w3402 -> [_ w3471]
          frame False {
          }
          frame True {
            n1527 = call "GetSNR(SubVI).vi"("Waveform"=w3478) -> ("SNR"=→"SNR1":dbl)  [unwired: 10 in]
            n1528 = Array Size(array=w3478) -> (size(s)=w3480:i32)
            n1529 = call "GetSNR(SubVI).vi"("Waveform"=w3482) -> ("SNR"=→"SNR2":dbl)  [unwired: 10 in]
            n1530 = call "GetSNR(SubVI).vi"("Waveform"=w3481) -> ("SNR"=→"SNR3":dbl)  [unwired: 10 in]
            n1531 = global read "GlobalVariables.vi" "BG Idx2"() -> (w3479:i32)
            n1532 = Subtract(x=w3480, y=w3479) -> (x-y=w3477:i32)
            n1533 = Array Subset(array=w3478, index=w3479, length=w3477) -> (w3486:dbl[])
            n1534 = Array Subset(array=w3482, index=w3479, length=w3477) -> (w3488:dbl[])
            n1535 = Array Subset(array=w3481, index=w3479, length=w3477) -> (w3490:dbl[])
            n1536 = Add Array Elements(numeric array=w3486) -> (sum=w3487:dbl)
            n1537 = Add Array Elements(numeric array=w3488) -> (sum=w3489:dbl)
            n1538 = Add Array Elements(numeric array=w3490) -> (sum=w3491:dbl)
            n1539 = Divide(x=w3487, y=w3473) -> (x/y=w3492:dbl)
            n1540 = Divide(x=w3489, y=w3472) -> (x/y=w3493:dbl)
            n1541 = Divide(x=w3491, y=w3471) -> (x/y=w3494:dbl)
            n1542 = Build Array(w3492, w3493, w3494) -> (w3495:dbl[])
            n1543 = Add Array Elements(numeric array=w3495) -> (sum=w3496:dbl)
            n1544 = Divide(x=w3495, y=w3496) -> (x/y=w3497:dbl[])
            n1545 = Index Array(array=w3497, index=2) -> (element=→"IntR3":dbl)
            n1546 = Index Array(array=w3497, index=1) -> (element=→"IntR2":dbl)
            n1547 = Index Array(array=w3497, index=0) -> (element=→"IntR1":dbl)
          }
        }
        n1548 = Add(x=w3418, y=w3458) -> (x+y=w3455:dbl[])
        n1549 = Add(x=w3419, y=w3453) -> (x+y=w3452:dbl[])
        n1550 = Add(x=w3420, y=w3450) -> (x+y=w3449:dbl[])
        n1551 = Less?(x=w3411, y=1.2 ("x")) -> (x < y?=w3409:bool)
        n1552 = Less?(x=w3406, y=1.2 ("x")) -> (x < y?=w3405:bool)
        n1553 = Less?(x=w3402, y=1.2 ("x")) -> (x < y?=w3401:bool)
        n1554 = case shown="False" w3401 {
          tunnel: [u32 16448250 ("Plot.Plot Color") u32 16711680 ("Plot.Plot Color")] -> w3400
          frame False {
          }
          frame True {
          }
        }
        n1555 = case shown="True" "Show BG removed?" {
          tunnel: w3456 -> [w3504 w3513]
          tunnel: w3455 -> [_ w3512]
          tunnel: [w3504 w3511] -> w3448
          tunnel: w3454 -> [w3503 w3510]
          tunnel: [w3503 w3509] -> w3442
          tunnel: w3452 -> [_ w3508]
          tunnel: w3451 -> [w3502 w3507]
          tunnel: [w3502 w3506] -> w3435
          tunnel: w3449 -> [_ w3505]
          frame False {
          }
          frame True {
            n1556 = Build Array (concatenate)(w3507, w3505) -> (w3506:dbl[][])
            n1557 = Build Array (concatenate)(w3513, w3512) -> (w3511:dbl[][])
            n1558 = Build Array (concatenate)(w3510, w3508) -> (w3509:dbl[][])
          }
        }
        "Channel 1" <- w3448
        "Channel 2" <- w3442
        "Channel 3" <- w3435
        n1559 = case shown="False" w3409 {
          tunnel: [u32 16448250 ("Plot.Plot Color") u32 16711680 ("Plot.Plot Color")] -> w3408
          frame False {
          }
          frame True {
          }
        }
        n1560 = case shown="False" w3405 {
          tunnel: [u32 16448250 ("Plot.Plot Color") u32 16711680 ("Plot.Plot Color")] -> w3404
          frame False {
          }
          frame True {
          }
        }
        n1561 = Array Size(array=w3435) -> (size(s)=w3436:i32[])
        n1562 = Array Size(array=w3448) -> (size(s)=w3447:i32[])
        n1563 = Array Size(array=w3442) -> (size(s)=w3441:i32[])
        n1564 = Index Array(array=w3436) -> (element=w3434:i32)  [unwired: 1 in]
        n1565 = Index Array(array=w3447) -> (element=w3446:i32)  [unwired: 1 in]
        n1566 = Index Array(array=w3441) -> (element=w3440:i32)  [unwired: 1 in]
        n1567 = property on="Channel 3" class="WFGraph (strict)"("Active Plot"=w3434, "Plot.Plot Color"=u32 16741120, "Plot.Line Style"=u8 1, "Plot.Line Width"=u8 2, "BG Color"=w3400) -> ()  [unwired: 2 in, 2 out]
        n1568 = property on="Channel 1" class="WFGraph (strict)"("Active Plot"=w3446, "Plot.Plot Color"=u32 16741120, "Plot.Line Style"=u8 1, "Plot.Line Width"=u8 2, "BG Color"=w3408) -> ()  [unwired: 2 in, 2 out]
        n1569 = property on="Channel 2" class="WFGraph (strict)"("Active Plot"=w3440, "Plot.Plot Color"=u32 16741120, "Plot.Line Style"=u8 1, "Plot.Line Width"=u8 2, "BG Color"=w3404) -> ()  [unwired: 2 in, 2 out]
      }
      frame Error {
        w3514 = u32 16448250 ("Plot Area:Colors:BG Color")
        n1570 = property on="Channel 1" class="WFGraph (strict)"("BG Color"=w3514) -> ()  [unwired: 2 in, 2 out]
        n1571 = property on="Channel 2" class="WFGraph (strict)"("BG Color"=w3514) -> ()  [unwired: 2 in, 2 out]
        n1572 = property on="Channel 3" class="WFGraph (strict)"("BG Color"=w3514) -> ()  [unwired: 2 in, 2 out]
      }
    }
    "DisplayLoop" <- w3393
  }
  n1573 = disable-structure "Diagram Disable Structure" shown="Disabled" {
    frame Disabled {
      w3516 = T51 {"Horizontal"=500, "Vertical"=100}  # Top Left Corner
      n1574 = Control Help Window(0:w3516, 1:TRUE ("Show")) -> ()
      n1575 = call <vilib>:"TDMS - File Viewer.vi"() -> ()  [unwired: 6 in, 2 out]
    }
    frame Enabled {
    }
  }
  n1576 = while {
    tunnel: w18 -> [w3554]
    shift-right: [w3527] -> _
    shift-left: _ -> [w3549]
    i -> [w3529]
    stop <- w3518 stop-if-true
    # "Channel 3"
    # "Channel 2"
    # "Channel 1"
    # "use FGV for gain value"
    # "stop on error"
    # "Gain adjustment and Data processing"
    n1577 = Tick Count (ms)() -> (millisecond timer value=w3527:u32)
    n1578 = Wait on Notification(notifier=w3554, ignore previous (F)=TRUE) -> (notification=w3521:T13, error out=w3522:errorcluster)  [unwired: 2 in, 2 out]
    n1579 = Subtract(x=w3527, y=w3549) -> (x-y=→"PID loop timing(ms)":u32)
    n1580 = Unbundle(w3521) -> ("CH1&2"=w3541:dbl[][], "CH3"=w3540:dbl[][])  [unwired: 2 out]
    n1581 = call "SeperateChanData.vi"("Input (Ch1&2)"=w3541) -> ("Ch1"=w3536:dbl[][], "Ch2"=w3534:dbl[][])
    n1582 = call "SeperateChanData.vi"("Input (Ch1&2)"=w3540) -> ("Ch1"=w3528:dbl[][])  [unwired: 1 out]
    n1583 = call "AvgArrayTimeCritical.vi"("2D array"=w3536) -> ("1D Avg"=w3535:dbl[])  [unwired: 10 in]
    n1584 = call "AvgArrayTimeCritical.vi"("2D array"=w3534) -> ("1D Avg"=w3547:dbl[])  [unwired: 10 in]
    n1585 = call "AvgArrayTimeCritical.vi"("2D array"=w3528) -> ("1D Avg"=w3542:dbl[])  [unwired: 10 in]
    n1586 = Array Max & Min(array=w3535) -> (max value=w3533:dbl)  [unwired: 3 out]
    n1587 = Array Max & Min(array=w3547) -> (max value=w3532:dbl)  [unwired: 3 out]
    n1588 = Array Max & Min(array=w3542) -> (max value=w3530:dbl)  [unwired: 3 out]
    n1589 = local read "Auto gain ch1"() -> (w3539:bool)
    n1590 = local read "Auto gain ch2"() -> (w3538:bool)
    n1591 = local read "Auto gain ch3"() -> (w3537:bool)
    n1592 = case shown="True" w3539 {
      tunnel: "V target(1.0)" -> [_ w3568]
      tunnel: w3533 -> [_ w3565]
      tunnel: [0.0 ("CtrlV") w3557] -> w3519
      tunnel: [FALSE w3559] -> w3526
      tunnel: w3522 -> [_ _]
      frame False {
        # "Manual control"
      }
      frame True {
        # "PID control"
        n1593 = global read "GlobalVariables.vi" "Ch1GainLim(Log)"() -> (w3564:cluster{"GainMax":dbl, "GainMin":dbl})
        n1594 = call-poly <vilib>:"PID.vi"("output range"=w3564, "PID gains"="Ch1 PID gains", "process variable"=w3565, "setpoint"=w3568) -> ("output"=w3563:dbl)  [unwired: 6 in, 1 out]
        n1595 = Power Of 10(x=w3563) -> (10^x=w3562:dbl)
        "Gain1" <- w3562
        n1596 = call "V1FGV.vi"("action (write)"=enum16{"write", "read"}."read") -> ("Error Out"=w3558:errorcluster, "V1 out"=w3560:dbl)  [unwired: 9 in]
        n1597 = call "GainToCtrlV.vi"("Gain"=w3562, "Channel"=enum16{"Ch1", "Ch2", "Ch3"}."Ch1") -> ("CtrlV"=w3557:dbl)  [unwired: 8 in, 1 out]
        n1598 = local write "V 1"(w3557) -> ()
        n1599 = call "V1FGV.vi"("Error In"=w3558, "V1 in"=w3557) -> ()  [unwired: 8 in, 2 out]
        n1600 = Not Equal?(x=w3557, y=w3560) -> (x != y?=w3559:bool)
      }
    }
    n1601 = case shown="True" w3538 {
      tunnel: w3532 -> [_ w3617]
      tunnel: "V target(1.0)" -> [_ w3618]
      tunnel: [FALSE w3611] -> w3525
      tunnel: w3522 -> [_ _]
      tunnel: [0.0 ("CtrlV") w3607] -> w3520
      frame False {
        # "Manual control"
      }
      frame True {
        # "PID control"
        n1602 = global read "GlobalVariables.vi" "Ch2GainLim(Log)"() -> (w3615:cluster{"GainMax":dbl, "GainMin":dbl})
        n1603 = call-poly <vilib>:"PID.vi"("output range"=w3615, "PID gains"="Ch2 PID gains", "process variable"=w3617, "setpoint"=w3618) -> ("output"=w3614:dbl)  [unwired: 6 in, 1 out]
        n1604 = Power Of 10(x=w3614) -> (10^x=w3612:dbl)
        "Gain2" <- w3612
        n1605 = call "V2FGV.vi"("action(write)"=enum16{"write", "read"}."read") -> ("Error Out"=w3608:errorcluster, "V2 out"=w3609:dbl)  [unwired: 9 in]
        n1606 = call "GainToCtrlV.vi"("Gain"=w3612, "Channel"=enum16{"Ch1", "Ch2", "Ch3"}."Ch2") -> ("CtrlV"=w3607:dbl)  [unwired: 8 in, 1 out]
        n1607 = local write "V 2"(w3607) -> ()
        n1608 = call "V2FGV.vi"("Error In"=w3608, "V2 in"=w3607) -> ()  [unwired: 8 in, 2 out]
        n1609 = Not Equal?(x=w3607, y=w3609) -> (x != y?=w3611:bool)
      }
    }
    n1610 = case shown="True" w3537 {
      tunnel: w3530 -> [_ w3602]
      tunnel: "V target(1.0)" -> [_ w3599]
      tunnel: w3522 -> [_ _]
      tunnel: [FALSE w3595] -> w3524
      tunnel: [0.0 ("CtrlV") w3593] -> w3523
      frame False {
        # "Manual control"
      }
      frame True {
        # "PID control"
        n1611 = global read "GlobalVariables.vi" "Ch3GainLim(Log)"() -> (w3603:cluster{"GainMax":dbl, "GainMin":dbl})
        n1612 = call-poly <vilib>:"PID.vi"("output range"=w3603, "PID gains"="Ch3 PID gains", "process variable"=w3602, "setpoint"=w3599) -> ("output"=w3601:dbl)  [unwired: 6 in, 1 out]
        n1613 = Power Of 10(x=w3601) -> (10^x=w3598:dbl)
        "Gain3" <- w3598
        n1614 = call "V3FGV.vi"("action(write)"=enum16{"write", "read"}."read") -> ("Error Out"=w3594:errorcluster, "V3 out"=w3596:dbl)  [unwired: 9 in]
        n1615 = call "GainToCtrlV.vi"("Gain"=w3598, "Channel"=enum16{"Ch1", "Ch2", "Ch3"}."Ch3") -> ("CtrlV"=w3593:dbl)  [unwired: 8 in, 1 out]
        n1616 = local write "V 3"(w3593) -> ()
        n1617 = call "V3FGV.vi"("Error In"=w3594, "V3 in"=w3593) -> ()  [unwired: 8 in, 2 out]
        n1618 = Not Equal?(x=w3593, y=w3596) -> (x != y?=w3595:bool)
      }
    }
    n1619 = call "LabJack_FGV.vi"("Operation(Read)"=enum16{"Write", "Read"}."Read" ("Operation"), "error in (no error)"=w3522) -> ("error out"=w3552:errorcluster, "Read data"=w3551:i32)  [unwired: 8 in]
    n1620 = case "Channel 1" shown="True" w3526 {
      tunnel: w3552 -> [w3584 w3590]
      tunnel: w3551 -> [w3583 w3589]
      tunnel: [w3584 w3585] -> w3546
      tunnel: [w3583 w3588] -> w3544
      tunnel: w3519 -> [_ w3586]
      frame False {
        # "Do nothing"
      }
      frame True {
        # "request V\nupdate FGV"
        n1621 = global read "GlobalVariables.vi" "Ch1 LJ pin"() -> (w3587:string)
        n1622 = call "LJM_eWriteName.vi"("Handle In"=w3589, "Name"=w3587, "Value"=w3586, "error in"=w3590) -> ("Handle Out"=w3588:i32, "error out"=w3585:errorcluster)  [unwired: 10 in]
      }
    }
    n1623 = case "Channel 2" shown="True" w3525 {
      tunnel: w3546 -> [w3575 w3582]
      tunnel: [w3575 w3577] -> w3545
      tunnel: w3544 -> [w3576 w3581]
      tunnel: [w3576 w3580] -> w3543
      tunnel: w3520 -> [_ w3578]
      frame False {
        # "Do nothing"
      }
      frame True {
        # "request V\nupdate FGV"
        n1624 = global read "GlobalVariables.vi" "Ch2 LJ pin"() -> (w3579:string)
        n1625 = call "LJM_eWriteName.vi"("Handle In"=w3581, "Name"=w3579, "Value"=w3578, "error in"=w3582) -> ("Handle Out"=w3580:i32, "error out"=w3577:errorcluster)  [unwired: 10 in]
      }
    }
    n1626 = case "Channel 3" shown="True" w3524 {
      tunnel: w3545 -> [w3569 w3574]
      tunnel: [w3569 w3570] -> w3518
      tunnel: w3543 -> [_ w3573]
      tunnel: w3523 -> [_ w3571]
      frame False {
        # "Do nothing"
      }
      frame True {
        # "request V\nupdate FGV"
        n1627 = global read "GlobalVariables.vi" "Ch3 LJ pin"() -> (w3572:string)
        n1628 = call "LJM_eWriteName.vi"("Handle In"=w3573, "Name"=w3572, "Value"=w3571, "error in"=w3574) -> ("error out"=w3570:errorcluster)  [unwired: 10 in, 1 out]
      }
    }
    "PID loop error out" <- w3518
    "PID loop" <- w3529
  }
  n1629 = Release Notifier(notifier=w15, error in (no error)=w48) -> (error out=w49:errorcluster)  [unwired: 1 in, 2 out]
  n1630 = Release Notifier(notifier=w16, error in (no error)=w37) -> (error out=w42:errorcluster)  [unwired: 1 in, 2 out]
  n1631 = call <vilib>:"Simple Error Handler.vi"("error in (no error)"=w49) -> ()  [unwired: 4 in, 5 out]
  n1632 = call <vilib>:"Simple Error Handler.vi"("error in (no error)"=w42) -> ()  [unwired: 4 in, 5 out]
  n1633 = Unregister For Events(event registration refnum=w45, error in=w3) -> (error out=w51:errorcluster)
  n1634 = Destroy User Event(user event=w38, error in=w51) -> (error out=w2:errorcluster)
  n1635 = Close File(refnum=w20, error in=w2) -> ()  [unwired: 2 out]
  n1636 = Release Notifier(notifier=w58, error in (no error)=w57) -> (error out=w56:errorcluster)  [unwired: 1 in, 2 out]
  n1637 = Unregister For Events(event registration refnum=w62, error in=w60) -> (error out=w61:errorcluster)
  n1638 = call <vilib>:"Simple Error Handler.vi"("error in (no error)"=w56) -> ()  [unwired: 4 in, 5 out]
  n1639 = Destroy User Event(user event=w52, error in=w61) -> ()  [unwired: 1 out]
